vi "SBND_TST.vi"() -> ()   [LabVIEW 2014]
uses:
  D:/share/SBND/SBNE_SW/LBNE_DLL/LBNE_DLL/bin/Debug/LBNE_DLL.dll
  LBNE_DLL/LBNE_DLL/bin/Debug/LBNE_DLL.dll
  LBNE_Global .vi
  <vilib>/express/express analysis/Spectral/Block/exnSpectralBlock spectral measurements peak poly.vi
  <vilib>/express/express analysis/Spectral/Block/exnSpectralBlock spectral measurements peak WFM.vi
  <vilib>/express/express analysis/Spectral/XNode/ExpressSpectralMeasurementsBlockNode.xnode
  <vilib>/Analysis/NI_AAL_SigProc.lvlib
  <instrlib>/RIGOL DP1000 Series/RIGOL DP1000 Series.lvlib
panel:
  out "error out":errorcluster={"status"=TRUE, "code"=-1073807343, "source"="VISA Open in RIGOL DP1000 Series.lvlib:Initialize.vi->SBND_TST.vi"}
  out "VISA resource name out":refnum<visa-resource-name>
  out "ADC_hist":u32[][](array[numeric])
  out "FF_B_SHFT 2":u32 format="%x"
  out "TP_RES":u32=39382807
  out "FE RB":u32[](array[numeric])=[3368601800, 3368601800, 3368601800, 3368601800, 3368601800, 3368601800, 3368601800, 3368601800, 3355494400, 3368601800, 3368601800, 3368601800, 3368601800, 3368601800, 3368601800, 3368601800, 13107400, 3368602828, 3368602828, 3368602828, 3368602828, 3368602828, 3368602828, 3368602828, 3368602828, 3355495424, 3368602828, 3368602828, 3368602828, 3368602828, 3368602828, 3368602828, 3368602828, 13107404] format="%x"
  out "Array 2":u32[](array[numeric])=[3368601800, 3368601800, 3368601800, 3368601800, 3368601800, 3368601800, 3368601800, 3368601800, 3355494400, 3368601800, 3368601800, 3368601800, 3368601800, 3368601800, 3368601800, 3368601800, 13107400, 3368602828, 3368602828, 3368602828, 3368602828, 3368602828, 3368602828, 3368602828, 3368602828, 3355495424, 3368602828, 3368602828, 3368602828, 3368602828, 3368602828, 3368602828, 3368602828, 13107404] format="%x"
  out "ADC RB":u32[](array[numeric])=[202116108, 202116108, 202116108, 202116108, 202116620, 202116108, 202116108, 202116108, 422910261, 404232216, 404232216, 404232216, 404232216, 404232216, 404232216, 404232216, 1779984920, 808595506, 808464432, 808464432, 808464432, 808464432, 808464432, 808464432, 808464432, 1691641044, 1616928864, 1616928864, 1616928864, 1616928864, 1616928864, 1616928864, 1616928864, 2824906848, 589833] format="%x"
  out "Array":u32[](array[numeric])=[202116108, 202116108, 202116108, 202116108, 202116620, 202116108, 202116108, 202116108, 422910261, 404232216, 404232216, 404232216, 404232216, 404232216, 404232216, 404232216, 1779984920, 808595506, 808464432, 808464432, 808464432, 808464432, 808464432, 808464432, 808464432, 1691641044, 1616928864, 1616928864, 1616928864, 1616928864, 1616928864, 1616928864, 1616928864, 2824906848, 589833] format="%x"
  out "FF_B_SHFT":u32 format="%x"
  in  "stop":bool
  in  "Tab Control":T1(tab)=enum."UDP CONTROL"
  in  "RESET 6":bool
  in  "samples 3":i32
  in  "CHANNEL":u8(slide)=14
  in  "Tab Control 3":enum32{"CLOCK PHASE CONTROL", "DC CONTROL"}(tab)
  in  "DATA SHIFT":u8[](array[numeric])=[0, 0, 0, 0, 0, 0, 0, 0] format="%x"
  in  "ADC_TM EN":bool
  in  "TEST PAT":u32=273 format="%x"
  in  "TEST EN":u32 format="%x"
  out "result":u32=17891328
  in  "ADC  CLK \nPHASE":bool[](array[boolean])=[FALSE, TRUE, TRUE, TRUE, TRUE, TRUE, TRUE, TRUE]
  in  "ASIC/CHN READOUT":bool=TRUE
  in  "RESTART":bool
  in  "ENABLE/\n DISABLE":bool
  in  "Voltage Level":dbl=1.6160000000000012 caption="Voltage Level (0 V)" format="%.2f"
  in  "Enable Output":bool=TRUE caption="Enable Output (T: Enable)"
  in  "START VOLTAGE":dbl caption="Voltage Level (0 V)" format="%.2f"
  in  "STOP VOLTAGE":dbl=1.6 caption="Voltage Level (0 V)" format="%.2f"
  in  "STEPS":dbl=100.0 caption="Voltage Level (0 V)" format="%.2f"
  out "Elapsed Time (s)":dbl=4.0854082107543945
  in  "Time Target (s)":dbl=4.0
  in  "number_of_samples":u32=10000
  in  "FREQ":u16=600
  in  "DLY":u8=239
  in  "AMPL":u8=23 format="%x"
  in  "CHIP":u8(slide)=1 scale=0.0..7.0
  in  "STOP_DATA":bool
  in  "AUTO SCALE":bool
  in  "x":u32=100
  out "ADC_RMS":dbl=266.1273079482756
  out "ADC_MEAN":dbl=878.6148385161484
  out "ADC_CNT":u32=10001
  out "ADC_PEAK":u32=861
  out "Waveform Graph 4":u32[](graph)
  out "ADC HIST":u32[](graph)=[0, 0, 0, 0, 0, 0, 0, 0, 0, 0, 0, 0, 0, 0, 0, 0, 0, 0, 0, 0, 0, 0, 0, 0, 0, 0, 0, 0, 0, 0, 0, 0, 0, 0, 0, 0, 0, 0, 0, 0, 0, 0, 0, 0, 0, 0, 0, 0, 0, 0, 0, 0, 0, 0, 0, 0, 0, 0, 0, 0, 0, 0, 0, 0, 0, 0, 0, 0, 0, 0, 0, 0, 0, 0, 0, 0, 0, 0, 0, 0, 0, 0, 0, 0, 0, 0, 0, 0, 0, 0, 0, 3, 6, 14, 34, 77, 158, 218, 258, 291, 228, 164, 164, 168, 206, 287, 248, 250, 130, 89, 50, 19, 10, 1, 1, 1, 1, 0, 0, 0, 0, 0, 0, 0, 0, 0, 0, 1192, 0, 0, 0, 0, 13, 22, 54, 224, 504, 905, 1368, 2740, 1873, 2049, 2667, 2499, 2671, 2484, 1903, 2513, 2643, 2551, 4237, 7695, 9164, 11409, 12405, 9832, 11511, 10095, 5591, 4006, 2700, 1449, 1009, 1689, 2755, 2668, 2468, 1996, 1241, 770, 588, 245, 170, 240, 279, 310, 502, 281, 313, 266, 144, 101, 37, 16, 2, 1, 0, 0, 0, 0, 0, 1, 1, 2, 5, 22, 20, 108, 384, 374, 456, 2012, 1429, 1580, 2732, 1877, 2486, 1878, 1144, 1090, 1311, 994, 1135, 1240, 1593, 1908, 1396, 1330, 1168, 892, 905, 814, 483, 295, 160, 89, 33, 46, 24, 4, 2, 2, 0, 0, 0, 0, 0, 0, 0, 0, 0, 0, 0, 0, 0, 0, 0, 0, 0, 0, 0, 0, 0, 0, 0, 0, 0, 0, 0, 0, 0, 0, 0, 0, 0, 0, 0, 0, 0, 0, 0, 0, 0, 0, 0, 0, 0, 0, 0, 0, 0, 0, 0, 0, 0, 0, 0, 0, 0, 0, 0, 0, 0, 0, 0, 0, 0, 0, 0, 0, 0, 0, 0, 0, 0, 0, 0, 0, 0, 0, 0, 0, 0, 0, 0, 0, 0, 0, 0, 0, 0, 0, 0, 0, 0, 0, 0, 0, 0, 0, 0, 2, 0, 0, 0, 5, 5, 7, 13, 24, 53, 59, 57, 93, 90, 175, 151, 197, 231, 224, 185, 146, 154, 201, 194, 224, 298, 282, 356, 374, 409, 536, 727, 778, 721, 849, 740, 553, 700, 735, 1000, 603, 707, 1034, 1109, 821, 927, 785, 595, 567, 564, 330, 366, 679, 55, 1, 1, 1, 0, 0, 0, 0, 0, 0, 0, 0, 0, 0, 0, 0, 0, 0, 0, 0, 0, 0, 0, 0, 0, 0, 0, 0, 0, 0, 0, 0, 0, 0, 0, 0, 0, 0, 0, 0, 0, 0, 0, 0, 0, 0, 1, 0, 0, 0, 0, 0, 2, 2, 5, 4, 9, 7, 10, 26, 46, 40, 90, 1082, 322, 1088, 442, 836, 439, 891, 1626, 760, 547, 1757, 841, 554, 1030, 578, 730, 569, 318, 226, 242, 126, 107, 91, 115, 102, 124, 163, 170, 131, 182, 201, 203, 244, 369, 265, 317, 386, 487, 538, 624, 601, 665, 707, 820, 906, 953, 794, 673, 685, 469, 733, 626, 476, 385, 317, 328, 276, 263, 185, 130, 92, 60, 80, 64, 1093, 4, 168, 88, 166, 112, 193, 168, 236, 209, 214, 209, 218, 117, 119, 109, 117, 211, 200, 177, 224, 226, 217, 201, 197, 187, 254, 261, 262, 331, 401, 412, 458, 653, 682, 552, 817, 940, 903, 979, 991, 965, 1040, 1249, 1244, 1239, 1034, 1100, 711, 784, 894, 1195, 523, 649, 797, 987, 475, 685, 512, 204, 300, 331, 151, 221, 328, 637, 204, 39, 56, 84, 56, 40, 26, 19, 22, 22, 14, 13, 18, 7, 21, 8, 5, 6, 2, 2, 2, 2, 6, 7, 4, 7, 2, 9, 7, 2, 7, 13, 8, 9, 3, 8, 2, 3, 5, 3, 0, 3, 6, 1, 6, 0, 1, 1, 0, 0, 0, 3, 1, 0, 2, 0, 2, 2, 5, 7, 16, 25, 301, 112, 514, 193, 396, 270, 283, 249, 516, 499, 378, 223, 424, 114, 78, 143, 127, 98, 69, 87, 65, 52, 26, 12, 7, 4, 6, 2, 1, 0, 0, 0, 0, 0, 0, 1, 0, 0, 0, 1, 1, 2, 1, 2, 0, 6, 7, 14, 15, 17, 31, 43, 30, 73, 136, 223, 146, 325, 332, 217, 337, 577, 273, 709, 6565, 1020, 4028, 3190, 2670, 1367, 6064, 12963, 9682, 7447, 16075, 35640, 37568, 39568, 49342, 52439, 69153, 132918, 141159, 153723, 209388, 258329, 308095, 353864, 329546, 357993, 372338, 444794, 403668, 387789, 442035, 387599, 373766, 462530, 389136, 302585, 345607, 255765, 200030, 226602, 175065, 138775, 108854, 98961, 97466, 86035, 74698, 54581, 80731, 88694, 89089, 83800, 71862, 89184, 108548, 56989, 62075, 90008, 45061, 61853, 81792, 60331, 54353, 81241, 387831, 75572, 285158, 53776, 81654, 51495, 48849, 31904, 48817, 41495, 26095, 8387, 15990, 2815, 1498, 2528, 1399, 770, 476, 633, 523, 440, 398, 545, 737, 610, 628, 705, 501, 707, 954, 756, 687, 892, 578, 366, 779, 785, 594, 493, 404, 314, 394, 323, 222, 148, 104, 78, 32, 53, 38, 43, 18, 19, 26, 40, 74, 91, 86, 157, 201, 267, 148, 370, 3626, 628, 4250, 1896, 5374, 3547, 6713, 22196, 17972, 7155, 67075, 46912, 30392, 109706, 81820, 183064, 239866, 194477, 203621, 382631, 283708, 321162, 314384, 400619, 514366, 420790, 401774, 447681, 293012, 410139, 518465, 380312, 343262, 406642, 246054, 155890, 298769, 294920, 178359, 144732, 107398, 76592, 77281, 62194, 38478, 24710, 14754, 13399, 4397, 5646, 3688, 4994, 1182, 1748, 1773, 1489, 533, 710, 378, 154, 142, 250, 39, 119, 127, 0, 5, 2, 3, 0, 1, 1, 0, 0, 0, 0, 0, 0, 0, 0, 0, 0, 0, 0, 0, 0, 0, 0, 1, 0, 1, 2, 3, 1, 3, 7, 6, 24, 18, 20, 45, 83, 82, 108, 169, 158, 247, 377, 420, 467, 449, 601, 297, 575, 492, 1091, 351, 673, 974, 1000, 586, 969, 753, 351, 480, 821, 277, 691, 1794, 308, 823, 168, 281, 172, 140, 129, 176, 156, 74, 36, 78, 6, 7, 9, 5, 1, 0, 0, 0, 0, 1, 0, 1, 0, 0, 0, 0, 0, 0, 0, 0, 0, 0, 0, 0, 0, 0, 0, 0, 0, 0, 0, 0, 0, 0, 0, 0, 0, 0, 0, 0, 0, 0, 0, 0, 0, 0, 0, 0, 0, 0, 0, 0, 0, 0, 0, 0, 0, 0, 0, 0, 0, 0, 0, 0, 0, 0, 0, 0, 0, 0, 0, 0, 0, 0, 0, 0, 0, 0, 0, 0, 0, 0, 0, 0, 0, 0, 0, 0, 0, 0, 0, 0, 0, 0, 0, 0, 0, 0, 0, 0, 0, 0, 0, 0, 0, 0, 0, 0, 0, 0, 0, 0, 0, 1, 0, 0, 0, 4, 4, 5, 2, 11, 35, 22, 11, 96, 68, 49, 216, 167, 360, 420, 360, 363, 704, 566, 620, 575, 803, 1006, 863, 755, 814, 508, 817, 1036, 744, 619, 708, 410, 471, 513, 640, 272, 424, 253, 270, 202, 169, 281, 131, 115, 145, 23, 54, 37, 14, 15, 13, 5, 2, 1, 0, 0, 0, 0, 0, 0, 0, 0, 246, 0, 0, 0, 0, 0, 0, 0, 0, 0, 0, 0, 0, 0, 0, 2, 1, 2, 2, 2, 2, 4, 5, 10, 13, 13, 32, 39, 33, 100, 107, 123, 199, 247, 104, 202, 500, 531, 442, 602, 482, 531, 910, 885, 879, 695, 717, 824, 233, 845, 682, 592, 350, 602, 716, 348, 386, 444, 165, 113, 228, 76, 97, 257, 13, 87, 31, 102, 74, 83, 116, 249, 260, 175, 99, 458, 136, 101, 225, 148, 70, 38, 30, 22, 12, 4, 2, 2, 0, 1, 0, 0, 0, 0, 0, 0, 0, 0, 0, 0, 0, 0, 0, 0, 0, 0, 1, 0, 0, 0, 1, 0, 1, 2, 0, 1, 2, 2, 7, 4, 6, 3, 9, 12, 12, 16, 18, 746, 35, 1, 1, 0, 0, 2, 12, 22, 34, 80, 39, 36, 62, 54, 31, 22, 17, 16, 20, 7, 6, 6, 3, 2, 2, 1, 0, 0, 1, 1, 1, 8, 5, 10, 28, 28, 17, 10, 14, 13, 12, 7, 6, 6, 7, 8, 14, 19, 32, 38, 68, 83, 121, 141, 123, 159, 234, 100, 171, 193, 121, 142, 77, 160, 33, 0, 0, 0, 2, 0, 0, 0, 0, 0, 0, 0, 0, 0, 0, 0, 0, 0, 0, 0, 0, 0, 0, 0, 1, 0, 0, 1, 0, 0, 2, 4, 4, 9, 2, 3, 9, 16, 2, 21, 9, 5, 18, 23, 29, 44, 43, 50, 39, 63, 78, 44, 56, 114, 42, 97, 115, 139, 217, 156, 181, 203, 199, 6573, 195, 474, 303, 528, 388, 594, 913, 708, 452, 1655, 1032, 861, 2033, 1520, 2054, 2506, 1797, 2083, 1860, 1482, 1666, 1297, 1236, 1046, 827, 506, 401, 328, 258, 210, 80, 68, 82, 45, 21, 33, 65, 64, 68, 60, 73, 100, 65, 108, 115, 87, 134, 47, 115, 97, 81, 32, 39, 40, 47, 21, 19, 19, 1, 1, 5, 0, 0, 438, 0, 0, 0, 0, 1, 0, 0, 1, 1, 0, 0, 0, 0, 0, 0, 0, 0, 0, 0, 0, 0, 3, 3, 1, 11, 28, 30, 16, 23, 52, 20, 13, 8, 7, 8, 4, 6, 2, 1, 1, 0, 0, 0, 0, 0, 0, 0, 0, 0, 0, 0, 0, 0, 0, 0, 0, 0, 0, 0, 0, 0, 0, 0, 0, 0, 0, 0, 0, 0, 0, 0, 0, 0, 0, 0, 0, 0, 0, 0, 0, 0, 0, 0, 0, 0, 0, 0, 0, 0, 0, 0, 0, 0, 0, 0, 0, 0, 0, 0, 0, 0, 0, 0, 0, 0, 0, 0, 0, 0, 0, 0, 0, 0, 0, 0, 0, 0, 0, 0, 0, 0, 0, 0, 0, 0, 0, 0, 0, 0, 0, 0, 0, 0, 0, 0, 0, 0, 0, 0, 0, 0, 0, 0, 0, 0, 0, 0, 0, 0, 0, 0, 0, 0, 0, 0, 0, 0, 0, 0, 0, 0, 0, 0, 0, 0, 0, 0, 0, 0, 0, 0, 0, 0, 0, 0, 0, 0, 0, 1, 3, 3, 2, 10, 18, 17, 36, 108, 93, 76, 123, 184, 1105, 44, 250, 103, 200, 80, 74, 38, 45, 19, 14, 4, 4, 0, 0, 0, 1, 0, 0, 0, 0, 0, 0, 0, 0, 0, 0, 0, 0, 0, 0, 0, 0, 0, 0, 0, 0, 0, 0, 0, 0, 0, 0, 0, 0, 0, 0, 0, 0, 0, 0, 0, 0, 0, 0, 0, 0, 0, 0, 0, 0, 0, 0, 0, 0, 0, 0, 0, 0, 0, 0, 0, 0, 0, 0, 0, 0, 0, 0, 0, 0, 0, 0, 0, 0, 0, 0, 0, 0, 0, 0, 0, 0, 0, 0, 0, 0, 0, 0, 0, 0, 0, 0, 0, 0, 0, 0, 0, 0, 0, 0, 0, 0, 0, 0, 0, 0, 0, 0, 0, 0, 0, 0, 0, 0, 0, 0, 0, 0, 0, 0, 0, 0, 0, 0, 0, 0, 0, 0, 0, 0, 0, 0, 0, 0, 0, 0, 0, 0, 0, 0, 0, 0, 0, 0, 0, 0, 0, 0, 0, 0, 0, 0, 0, 0, 0, 0, 0, 0, 0, 0, 0, 0, 0, 0, 0, 0, 0, 0, 0, 0, 0, 0, 0, 0, 0, 0, 0, 0, 0, 0, 0, 0, 0, 0, 0, 0, 0, 0, 0, 0, 0, 0, 0, 0, 0, 0, 0, 0, 0, 0, 0, 0, 0, 0, 0, 0, 0, 0, 0, 0, 0, 0, 2, 0, 3, 1, 2, 1, 6, 6, 10, 17, 16, 24, 43, 70, 81, 111, 129, 99, 183, 228, 308, 225, 340, 615, 420, 565, 770, 492, 411, 825, 587, 642, 768, 1922, 498, 1701, 459, 688, 331, 449, 425, 210, 81, 282, 80, 35, 115, 29, 27, 15, 10, 5, 10, 3, 2, 3, 0, 1, 0, 0, 2, 0, 0, 0, 0, 0, 0, 0, 0, 0, 0, 0, 0, 0, 0, 0, 0, 0, 0, 0, 0, 0, 0, 0, 0, 0, 0, 0, 0, 0, 0, 0, 0, 0, 0, 0, 0, 0, 0, 0, 0, 0, 0, 0, 0, 0, 0, 0, 0, 0, 0, 0, 0, 0, 0, 0, 0, 0, 0, 0, 0, 0, 0, 0, 0, 0, 0, 0, 0, 0, 0, 0, 0, 0, 0, 0, 0, 0, 0, 0, 0, 0, 0, 0, 0, 0, 0, 0, 0, 0, 0, 0, 0, 0, 0, 0, 0, 0, 0, 0, 0, 0, 0, 0, 0, 0, 0, 0, 0, 0, 0, 0, 0, 0, 0, 0, 0, 0, 0, 0, 0, 0, 0, 0, 0, 0, 0, 0, 0, 0, 0, 0, 0, 0, 0, 0, 0, 0, 0, 0, 0, 0, 0, 0, 0, 0, 0, 0, 0, 0, 0, 0, 0, 0, 0, 0, 0, 0, 0, 0, 0, 0, 0, 0, 0, 0, 0, 0, 0, 0, 0, 0, 0, 0, 1, 0, 1, 0, 0, 1, 2, 14, 21, 19, 28, 52, 27, 97, 51, 62, 48, 83, 280, 155, 116, 308, 154, 96, 152, 63, 249, 131, 189, 21, 91, 30, 59, 16, 8, 17, 9, 3, 2, 3, 0, 1, 2, 7, 1, 7, 27, 22, 24, 60, 43, 33, 110, 112, 103, 3825, 0, 3, 12, 148, 194, 204, 1207, 883, 225, 887, 902, 399, 918, 329, 362, 991, 949, 364, 541, 316, 228, 206, 176, 210, 107, 85, 51, 49, 12, 16, 13, 5, 4, 4, 1, 0, 0, 0, 0, 0, 1, 0, 0, 0, 0, 0, 0, 0, 0, 0, 0, 0, 0, 0, 0, 0, 0, 0, 0, 0, 0, 0, 0, 0, 0, 0, 0, 0, 0, 0, 0, 0, 0, 0, 0, 0, 0, 0, 0, 0, 0, 0, 0, 0, 0, 0, 0, 0, 0, 0, 0, 0, 0, 0, 0, 0, 0, 0, 0, 0, 0, 0, 0, 1, 0, 1, 3, 4, 5, 11, 11, 15, 33, 45, 40, 97, 100, 103, 140, 244, 227, 223, 365, 242, 156, 125, 127, 256, 21, 49, 7, 2, 1, 0, 0, 1, 0, 0, 0, 0, 0, 0, 0, 0, 0, 0, 0, 0, 0, 0, 0, 0, 0, 0, 0, 0, 0, 0, 0, 0, 0, 0, 0, 0, 0, 0, 0, 0, 0, 0, 0, 0, 0, 0, 0, 0, 0, 0, 0, 0, 0, 0, 0, 0, 0, 0, 0, 0, 0, 0, 0, 0, 0, 0, 0, 0, 0, 0, 0, 0, 0, 0, 0, 0, 0, 0, 0, 0, 0, 0, 0, 0, 0, 0, 0, 0, 0, 0, 0, 0, 0, 0, 0, 0, 0, 0, 0, 0, 0, 0, 0, 0, 0, 0, 0, 0, 0, 0, 0, 0, 0, 0, 0, 0, 0, 0, 0, 0, 0, 0, 0, 0, 0, 0, 0, 0, 0, 0, 0, 0, 0, 0, 0, 0, 0, 0, 0, 0, 0, 0, 0, 0, 0, 0, 0, 0, 0, 0, 0, 0, 0, 0, 0, 0, 0, 0, 0, 0, 0, 0, 0, 0, 0, 0, 0, 0, 0, 0, 0, 0, 0, 0, 0, 0, 0, 0, 0, 0, 0, 0, 0, 0, 0, 0, 0, 0, 0, 0, 0, 0, 0, 0, 0, 0, 0, 0, 0, 0, 0, 0, 0, 0, 0, 0, 0, 0, 0, 0, 0, 0, 0, 0, 0, 0, 0, 0, 0, 0, 0, 0, 0, 0, 0, 0, 0, 0, 0, 0, 0, 0, 0, 0, 0, 0, 0, 0, 0, 0, 0, 0, 0, 0, 0, 0, 0, 0, 0, 0, 0, 0, 0, 0, 0, 0, 0, 0, 0, 2, 0, 1, 1, 4, 4, 18, 10, 23, 52, 54, 87, 124, 139, 164, 334, 266, 411, 354, 452, 682, 602, 649, 783, 633, 852, 980, 728, 603, 1049, 726, 563, 791, 782, 491, 475, 324, 240, 236, 186, 131, 116, 80, 37, 23, 36, 38, 16, 8, 8, 8, 1, 3, 0, 0, 0, 2, 1, 0, 1, 0, 0, 0, 0, 0, 0, 0, 0, 0, 0, 0, 0, 0, 0, 0, 0, 0, 0, 0, 0, 0, 0, 0, 0, 0, 0, 0, 0, 0, 0, 0, 0, 0, 0, 0, 0, 0, 0, 0, 0, 0, 0, 0, 0, 0, 0, 0, 0, 0, 0, 0, 0, 0, 0, 0, 0, 0, 0, 0, 0, 0, 0, 0, 0, 0, 0, 0, 0, 0, 0, 0, 0, 0, 0, 0, 0, 0, 0, 0, 0, 0, 0, 0, 0, 0, 0, 0, 0, 0, 0, 0, 0, 0, 0, 0, 0, 0, 0, 0, 0, 0, 0, 0, 0, 0, 0, 0, 0, 0, 0, 0, 0, 0, 0, 0, 0, 0, 0, 0, 0, 0, 0, 0, 0, 0, 0, 0, 0, 0, 0, 0, 0, 0, 0, 0, 0, 0, 0, 0, 0, 0, 0, 0, 0, 0, 0, 0, 0, 0, 0, 0, 0, 0, 0, 0, 0, 0, 0, 0, 0, 0, 0, 0, 0, 0, 0, 0, 0, 0, 0, 0, 0, 0, 0, 0, 0, 0, 0, 0, 0, 0, 0, 0, 0, 0, 0, 0, 0, 0, 0, 0, 0, 0, 0, 0, 0, 0, 0, 0, 0, 0, 0, 0, 0, 0, 0, 0, 0, 0, 0, 0, 0, 0, 0, 0, 0, 0, 0, 0, 0, 0, 0, 0, 0, 0, 0, 0, 0, 0, 0, 0, 0, 0, 0, 0, 0, 0, 0, 0, 0, 0, 0, 0, 0, 0, 0, 0, 0, 0, 0, 0, 0, 0, 0, 0, 0, 0, 0, 0, 0, 0, 0, 0, 0, 0, 0, 0, 0, 0, 0, 0, 0, 0, 0, 0, 0, 0, 0, 0, 0, 0, 0, 0, 0, 0, 0, 0, 0, 0, 0, 0, 0, 0, 0, 0, 0, 0, 0, 0, 0, 0, 0, 0, 0, 0, 0, 0, 0, 0, 0, 0, 0, 0, 0, 0, 0, 0, 0, 0, 0, 0, 0, 0, 0, 0, 0, 0, 0, 0, 0, 0, 0, 0, 0, 0, 0, 0, 0, 0, 0, 0, 0, 0, 0, 0, 0, 0, 0, 0, 0, 0, 0, 0, 0, 0, 0, 0, 0, 0, 0, 0, 0, 0, 0, 0, 0, 0, 0, 0, 0, 0, 0, 0, 0, 0, 0, 0, 0, 0, 0, 0, 0, 0, 0, 0, 0, 0, 0, 0, 0, 0, 0, 0, 0, 0, 0, 0, 0, 0, 0, 1, 0, 0, 0, 2, 6, 8, 6, 8, 18, 32, 39, 55, 124, 123, 166, 182, 171, 328, 273, 185, 182, 190, 181, 158, 87, 55, 16, 35, 7, 5, 7, 2, 1, 1, 0, 0, 0, 0, 1, 0, 0, 0, 0, 0, 0, 0, 0, 0, 0, 0, 0, 0, 0, 0, 0, 0, 0, 0, 0, 0, 0, 0, 0, 0, 0, 0, 0, 0, 0, 0, 0, 0, 0, 0, 0, 0, 0, 0, 0, 0, 0, 0, 0, 0, 0, 0, 0, 0, 0, 0, 0, 0, 0, 0, 0, 0, 0, 0, 0, 0, 0, 0, 0, 0, 0, 0, 0, 0, 0, 0, 0, 0, 0, 0, 0, 0, 0, 0, 0, 0, 0, 0, 0, 0, 0, 0, 0, 0, 0, 0, 0, 0, 0, 0, 0, 0, 0, 0, 0, 0, 0, 0, 0, 0, 0, 0, 0, 0, 0, 0, 0, 0, 0, 0, 0, 0, 0, 0, 0, 0, 0, 0, 0, 0, 0, 0, 0, 0, 0, 0, 0, 0, 0, 0, 0, 0, 0, 0, 0, 0, 0, 0, 0, 0, 0, 0, 0, 0, 0, 0, 0, 0, 0, 0, 0, 0, 0, 0, 0, 0, 1, 1, 0, 2, 1, 2, 11, 6, 16, 23, 81, 60, 89, 35, 105, 88, 176, 155, 118, 73, 40, 21, 25, 19, 14, 23, 13, 17, 26, 16, 12, 22, 12, 10, 3, 3, 0, 0, 1, 1, 1334, 0, 0, 0, 0, 0, 0, 0, 0, 0, 0, 0, 0, 0, 1, 1, 0, 0, 0, 0, 3, 0, 3, 4, 5, 8, 7, 14, 19, 38, 61, 56, 121, 142, 100, 173, 400, 369, 439, 502, 469, 510, 711, 666, 742, 727, 657, 732, 528, 689, 931, 474, 523, 813, 758, 410, 541, 490, 242, 235, 377, 136, 223, 732, 6, 417, 182, 734, 363, 366, 1072, 708, 292, 1128, 642, 507, 914, 663, 730, 1017, 636, 477, 925, 662, 530, 402, 375, 398, 255, 168, 158, 85, 61, 46, 32, 6, 11, 7, 3, 4, 3, 0, 0, 1, 0, 0, 0, 0, 0, 0, 0, 0, 0, 0, 0, 0, 0, 0, 0, 0, 0, 0, 0, 0, 0, 0, 0, 0, 0, 0, 0, 0, 0, 0, 0, 0, 0, 0, 0, 0, 0, 0, 0, 0, 0, 0, 0, 0, 0, 0, 0, 0, 0, 0, 0, 0, 0, 0, 0, 0, 0, 0, 0, 0, 0, 0, 0, 0, 0, 0, 0, 0, 0, 0, 0, 0, 0, 0, 0, 0, 0, 0, 0, 0, 0, 0, 0, 0, 0, 0, 0, 0, 0, 0, 0, 0, 0, 0, 0, 0, 0, 0, 0, 0, 0, 0, 0, 0, 0, 0, 0, 0, 0, 0, 0, 0, 0, 0, 0, 0, 1, 1, 1, 1, 5, 6, 5, 8, 16, 14, 22, 25, 38, 32, 40, 66, 77, 102, 103, 139, 184, 208, 262, 325, 297, 416, 420, 508, 481, 490, 370, 327, 238, 170, 165, 408, 867, 1745, 773, 605, 219, 189, 508, 231, 96, 57, 80, 63, 35, 17, 21, 7, 11, 5, 0, 1, 1, 1, 0, 0, 0, 0, 0, 0, 0, 0, 1, 0, 1, 0, 0, 0, 2, 2, 6, 2, 6, 16, 15, 15, 25, 33, 42, 45, 62, 56, 57, 43, 114, 109, 121, 180, 151, 148, 163, 113, 70, 36, 23, 60, 106, 441, 119, 48, 39, 42, 19, 17, 15, 16, 17, 7, 26, 20, 32, 117, 80, 126, 181, 151, 137, 140, 91, 203, 111, 45, 21, 18, 13, 3, 3, 1, 0, 0, 0, 1, 0, 0, 0, 0, 0, 0, 0, 0, 0, 0, 0, 0, 0, 0, 0, 0, 0, 0, 2, 1, 4, 9, 7, 19, 22, 30, 36, 191, 8, 249, 245, 354, 223, 260, 131, 211, 176, 129, 83, 122, 50, 23, 33, 23, 9, 2, 2, 0, 1, 0, 0, 0, 0, 0, 0, 0, 0, 0, 0, 0, 0, 0, 0, 0, 0, 0, 0, 0, 0, 0, 0, 0, 0, 0, 0, 0, 0, 0, 0, 0, 0, 0, 0, 0, 0, 0, 0, 0, 0, 0, 0, 0, 0, 0, 0, 0, 0, 0, 0, 0, 0, 0, 0, 0, 0, 0, 0, 0, 0, 0, 0, 0, 0, 0, 0, 0, 0, 0, 0, 0, 0, 0, 0, 0, 0, 0, 0, 0, 0, 0, 0, 0, 0, 0, 0, 0, 0, 0, 0, 0, 0, 0, 0, 0, 0, 0, 0, 0, 0, 0, 0, 0, 0, 0, 0, 0, 0, 0, 0, 0, 0, 1, 0, 4, 7, 18, 11, 51, 44, 55, 108, 152, 195, 154, 271, 267, 214, 259, 158, 179, 110, 143, 97, 33, 42, 39, 24, 10, 4, 2, 3, 0, 0, 0, 0, 0, 0, 0, 0, 0, 0, 0, 0, 0, 0, 0, 0, 0, 0, 0, 0, 0, 0, 0, 0, 0, 0, 0, 0, 1602, 0, 0, 0, 0, 0, 0, 0, 0, 0, 0, 0, 0, 0, 0, 0, 0, 0, 0, 0, 0, 0, 0, 0, 0, 0, 0, 1, 1, 3, 5, 1, 5, 12, 14, 5, 24, 42, 57, 57, 63, 78, 77, 100, 134, 195, 211, 170, 257, 278, 435, 412, 391, 475, 570, 447, 610, 593, 420, 373, 807, 443, 533, 508, 1825, 1306, 158, 165, 384, 133, 112, 202, 66, 13, 52, 16, 7, 6, 1, 0, 0, 0, 1, 0, 0, 0, 1, 1, 8, 11, 19, 38, 27, 45, 70, 95, 93, 247, 326, 307, 537, 854, 728, 587, 381, 262, 129, 74, 41, 55, 73, 71, 87, 79, 135, 108, 98, 104, 119, 82, 141, 140, 84, 51, 95, 46, 28, 22, 46, 9358, 1, 4, 1, 1, 2, 0, 0, 0, 0, 0, 0, 0, 0, 0, 0, 0, 0, 0, 0, 0, 0, 0, 0, 0, 0, 0, 0, 0, 0, 0, 0, 0, 0, 0, 0, 0, 0, 0, 0, 0, 0, 0, 0, 0, 0, 0, 0, 0, 0, 0, 0, 0, 0, 0, 0, 0, 0, 0, 0, 0, 0, 0, 0, 0, 0, 0, 0, 0, 0, 0, 0, 0, 0, 0, 0, 0, 0, 0, 0, 0, 0, 0, 0, 0, 0, 0, 0, 0, 0, 0, 0, 0, 0, 0, 0, 0, 0, 0, 0, 0, 0, 0, 0, 0, 0, 0, 0, 0, 0, 0, 0, 0, 0, 0, 0, 0, 0, 0, 0, 0, 0, 0, 0, 0, 0, 0, 0]
  out "samples 4":u32=20161263
  out "Waveform Graph 5":u32[](graph)=[871, 868, 866, 864, 864, 860, 861, 859, 860, 859, 858, 856, 857, 861, 864, 880, 1206, 2194, 3322, 3968, 3903, 3346, 2593, 1918, 1420, 1112, 951, 885, 863, 862, 861, 859, 855, 853, 852, 855, 856, 860, 861]
  in  "length":i32=39 min=10 max=65 step=1
  in  "SYNC":bool=TRUE
  in  "FILE PATH":path=path "C:/Users/jfried/Desktop/New folder (11)"
  in  "FILE NAME 2":string="1459002fff"
  in  "SAVE TO \nFILE":bool
  out "Store_Data":bool
  in  "SYNC 3":bool=TRUE
  out "Waveform Graph":cluster{"f0":dbl, "df":dbl, "magnitude":dbl[]}(graph)={"f0"=0.0, "df"=199.98000199980004, "magnitude"=array[5001 elements]}
  in  "Boolean":bool
  in  "EN peak":bool
  in  "peak upper limit":dbl=800.0
  in  "peak lower limit":dbl=700.0
  in  "EN mean":bool=TRUE
  in  "Start channel":u8
  in  "Start chip":u8
  out "CUR_CHP":u8=5 caption="CHIP"
  out "CUR_CHN":u8=7 caption="CHANNEL"
  in  "Tab Control 2":enum32{"Page 1", "Page 2"}(tab)=enum."Page 2"
  in  "length 2":i32=40 min=10 max=65 step=1
  out "Waveform Graph 6":u32[](graph)=[1526, 1518, 1514, 1520, 1526, 1528, 1520, 1518, 1524, 1526, 1522, 1516, 1516, 1516, 1514, 1512, 1790, 3620, 2450, 4094, 4094, 3966, 2180, 354, 3082, 2248, 1812, 1624, 1568, 1546, 1540, 1534, 1538, 1534, 1520, 1510, 1512, 1514, 1516, 1516]
  in  "AUTO SCALE 2":bool
  in  "x 2":u32=100
  out "ADC_RMS 2":dbl
  out "ADC_MEAN 2":dbl
  out "ADC_CNT 2":u32=6001
  out "ADC_PEAK 2":u32
  out "Waveform Graph 7":u32[](graph)
  out "ADC HIST  2":u32[](graph)=[877735, 0, 0, 0, 0, 0, 0, 0, 0, 0, 0, 0, 0, 0, 0, 0, 0, 0, 0, 0, 0, 0, 0, 0, 0, 0, 0, 0, 0, 0, 0, 0, 0, 0, 0, 0, 0, 0, 0, 0, 0, 0, 0, 0, 0, 0, 0, 0, 0, 0, 0, 0, 0, 0, 0, 0, 0, 0, 0, 0, 0, 0, 0, 0, 0, 0, 0, 0, 0, 0, 0, 0, 0, 0, 0, 0, 0, 0, 0, 0, 0, 0, 0, 0, 0, 0, 0, 0, 0, 0, 0, 0, 0, 0, 0, 0, 0, 0, 0, 0, 0, 0, 0, 0, 0, 0, 0, 0, 0, 0, 0, 0, 0, 0, 0, 0, 0, 0, 0, 0, 0, 0, 0, 0, 0, 0, 0, 0, 0, 0, 0, 0, 0, 0, 0, 0, 0, 0, 0, 0, 0, 0, 0, 0, 0, 0, 0, 0, 0, 0, 0, 0, 0, 0, 0, 0, 0, 0, 0, 0, 0, 0, 0, 0, 0, 0, 0, 0, 0, 0, 0, 0, 0, 0, 0, 0, 0, 0, 0, 0, 0, 0, 0, 0, 0, 0, 0, 0, 0, 0, 0, 0, 0, 0, 0, 0, 0, 0, 0, 0, 0, 0, 0, 0, 0, 0, 0, 0, 0, 0, 0, 0, 0, 0, 0, 0, 0, 0, 0, 0, 0, 0, 0, 0, 0, 0, 0, 0, 0, 0, 0, 0, 0, 0, 0, 0, 0, 0, 0, 0, 0, 0, 0, 0, 0, 0, 0, 0, 0, 0, 0, 0, 0, 0, 0, 0, 0, 0, 0, 0, 0, 0, 0, 0, 0, 0, 0, 0, 0, 0, 0, 0, 0, 0, 0, 0, 0, 0, 0, 0, 0, 0, 0, 0, 0, 0, 0, 0, 0, 0, 0, 0, 0, 0, 0, 0, 0, 0, 0, 0, 0, 0, 0, 0, 0, 0, 0, 0, 0, 0, 0, 0, 0, 0, 0, 0, 0, 0, 0, 0, 0, 0, 0, 0, 0, 0, 0, 0, 0, 0, 0, 0, 0, 0, 0, 0, 0, 0, 0, 0, 0, 0, 0, 0, 0, 0, 0, 0, 0, 0, 0, 0, 0, 0, 0, 0, 0, 0, 0, 0, 0, 0, 0, 0, 0, 0, 0, 0, 0, 0, 0, 0, 0, 0, 0, 0, 0, 0, 0, 0, 0, 0, 0, 0, 0, 0, 0, 0, 0, 0, 0, 0, 0, 0, 0, 0, 0, 0, 0, 0, 0, 0, 0, 0, 0, 0, 0, 0, 0, 0, 0, 0, 0, 0, 0, 0, 0, 0, 0, 0, 0, 0, 0, 0, 0, 0, 0, 0, 0, 0, 0, 0, 0, 0, 0, 0, 0, 0, 0, 0, 0, 0, 0, 0, 0, 0, 0, 0, 0, 0, 0, 0, 0, 0, 0, 0, 0, 0, 0, 0, 0, 0, 0, 0, 0, 0, 0, 0, 0, 0, 0, 0, 0, 0, 0, 0, 0, 0, 0, 0, 0, 0, 0, 0, 0, 0, 0, 0, 0, 0, 0, 0, 0, 0, 0, 0, 0, 0, 0, 0, 0, 0, 0, 0, 0, 0, 0, 0, 0, 0, 0, 0, 0, 0, 0, 0, 0, 0, 0, 0, 0, 0, 0, 0, 0, 0, 0, 0, 0, 0, 0, 0, 0, 0, 0, 0, 0, 0, 0, 0, 0, 0, 0, 0, 0, 0, 0, 0, 0, 0, 0, 0, 0, 0, 0, 0, 0, 0, 0, 0, 0, 0, 0, 0, 0, 0, 0, 0, 0, 0, 0, 0, 0, 0, 0, 0, 0, 0, 0, 0, 0, 0, 0, 0, 0, 0, 0, 0, 0, 0, 0, 0, 0, 0, 0, 0, 0, 0, 0, 0, 0, 0, 0, 0, 0, 0, 0, 0, 0, 0, 0, 0, 0, 0, 0, 0, 0, 0, 0, 0, 0, 0, 0, 0, 0, 0, 0, 0, 0, 0, 0, 0, 0, 0, 0, 0, 0, 0, 0, 0, 0, 0, 0, 0, 0, 0, 0, 0, 0, 0, 0, 0, 0, 0, 0, 0, 0, 0, 0, 0, 0, 0, 0, 0, 0, 0, 0, 0, 0, 0, 0, 0, 0, 0, 0, 0, 0, 0, 0, 0, 0, 0, 0, 0, 0, 0, 0, 0, 0, 0, 0, 0, 0, 0, 0, 0, 0, 0, 0, 0, 0, 0, 0, 0, 0, 0, 0, 0, 0, 0, 0, 0, 0, 0, 0, 0, 0, 0, 0, 0, 0, 0, 0, 0, 0, 0, 0, 0, 0, 0, 0, 0, 0, 0, 0, 0, 0, 0, 0, 0, 0, 0, 0, 0, 0, 0, 0, 0, 0, 0, 0, 0, 0, 0, 0, 0, 0, 0, 0, 0, 0, 0, 0, 0, 0, 0, 0, 0, 0, 0, 0, 0, 0, 0, 0, 0, 0, 0, 0, 0, 0, 0, 0, 0, 0, 0, 0, 0, 0, 0, 0, 0, 0, 0, 0, 0, 0, 0, 0, 0, 0, 0, 0, 0, 0, 0, 0, 0, 0, 0, 0, 0, 0, 0, 0, 0, 0, 0, 0, 0, 0, 0, 0, 0, 0, 0, 0, 0, 0, 0, 0, 0, 0, 0, 0, 0, 0, 0, 0, 0, 0, 0, 0, 0, 0, 0, 0, 0, 0, 0, 0, 0, 0, 0, 0, 0, 0, 0, 0, 0, 0, 0, 0, 0, 0, 0, 0, 0, 0, 0, 0, 0, 0, 0, 0, 0, 0, 0, 0, 0, 0, 0, 0, 0, 0, 0, 0, 0, 0, 0, 0, 0, 0, 0, 0, 0, 0, 0, 0, 0, 0, 0, 0, 0, 0, 0, 0, 0, 0, 0, 0, 0, 0, 0, 0, 0, 0, 0, 0, 0, 0, 0, 0, 0, 0, 0, 0, 0, 0, 0, 0, 0, 0, 0, 0, 0, 0, 0, 0, 0, 0, 0, 0, 0, 0, 0, 0, 0, 0, 0, 0, 0, 0, 0, 0, 0, 0, 0, 0, 0, 0, 0, 0, 0, 0, 0, 0, 0, 0, 0, 0, 0, 0, 0, 0, 0, 0, 0, 0, 0, 0, 0, 0, 0, 0, 0, 0, 0, 0, 0, 0, 0, 0, 0, 0, 0, 0, 0, 0, 0, 0, 0, 0, 0, 0, 0, 0, 0, 0, 0, 0, 0, 0, 0, 0, 0, 0, 0, 0, 0, 0, 0, 0, 0, 0, 0, 0, 0, 0, 0, 0, 0, 0, 0, 0, 0, 0, 0, 0, 0, 0, 0, 0, 0, 0, 0, 0, 0, 0, 0, 0, 0, 0, 0, 0, 0, 0, 0, 0, 0, 0, 0, 0, 0, 0, 0, 0, 0, 0, 0, 0, 0, 0, 0, 0, 0, 0, 0, 0, 0, 0, 0, 0, 0, 0, 0, 0, 0, 0, 0, 0, 0, 0, 0, 0, 0, 0, 0, 0, 0, 0, 0, 0, 0, 0, 0, 0, 0, 0, 0, 0, 0, 0, 0, 0, 0, 0, 0, 0, 0, 0, 0, 0, 0, 0, 0, 0, 0, 0, 0, 0, 0, 0, 0, 0, 0, 0, 0, 0, 0, 0, 0, 0, 0, 0, 0, 0, 0, 0, 0, 0, 0, 0, 0, 0, 0, 0, 0, 0, 0, 0, 0, 0, 0, 0, 0, 0, 0, 0, 0, 0, 0, 0, 0, 0, 0, 0, 0, 0, 0, 0, 0, 0, 0, 0, 0, 0, 0, 0, 0, 0, 0, 0, 0, 0, 0, 0, 0, 0, 0, 0, 0, 0, 0, 0, 0, 0, 0, 0, 0, 0, 0, 0, 0, 0, 0, 0, 0, 0, 0, 0, 0, 0, 0, 0, 0, 0, 0, 0, 0, 0, 0, 0, 0, 0, 0, 0, 0, 0, 0, 0, 0, 0, 0, 0, 0, 0, 0, 0, 0, 0, 0, 0, 0, 0, 0, 0, 0, 0, 0, 0, 0, 0, 0, 0, 0, 0, 0, 0, 0, 0, 0, 0, 0, 0, 0, 0, 0, 0, 0, 0, 0, 0, 0, 0, 0, 0, 0, 0, 0, 0, 0, 0, 0, 0, 0, 0, 0, 0, 0, 0, 0, 0, 0, 0, 0, 0, 0, 0, 0, 0, 0, 0, 0, 0, 0, 0, 0, 0, 0, 0, 0, 0, 0, 0, 0, 0, 0, 0, 0, 0, 0, 0, 0, 0, 0, 0, 0, 0, 0, 0, 0, 0, 0, 0, 0, 0, 0, 0, 0, 0, 0, 0, 0, 0, 0, 0, 0, 0, 0, 0, 0, 0, 0, 0, 0, 0, 0, 0, 0, 0, 0, 0, 0, 0, 0, 0, 0, 0, 0, 0, 0, 0, 0, 0, 0, 0, 0, 0, 0, 0, 0, 0, 0, 0, 0, 0, 0, 0, 0, 0, 0, 0, 0, 0, 0, 0, 0, 0, 0, 0, 0, 0, 0, 0, 0, 0, 0, 0, 0, 0, 0, 0, 0, 0, 0, 0, 0, 0, 0, 0, 0, 0, 0, 0, 0, 0, 0, 0, 0, 0, 0, 0, 0, 0, 0, 0, 0, 0, 0, 0, 0, 0, 0, 0, 0, 0, 0, 0, 0, 0, 0, 0, 0, 0, 0, 0, 0, 0, 0, 0, 0, 0, 0, 0, 0, 0, 0, 0, 0, 0, 0, 0, 0, 0, 0, 0, 0, 0, 0, 0, 0, 0, 0, 0, 0, 0, 0, 0, 0, 0, 0, 0, 0, 0, 0, 0, 0, 0, 0, 0, 0, 0, 0, 0, 0, 0, 0, 0, 0, 0, 0, 0, 0, 0, 0, 0, 0, 0, 0, 0, 0, 0, 0, 0, 0, 0, 0, 0, 0, 0, 0, 0, 0, 0, 0, 0, 0, 0, 0, 0, 0, 0, 0, 0, 0, 0, 0, 0, 0, 0, 0, 0, 0, 0, 0, 0, 0, 0, 0, 0, 0, 0, 0, 0, 0, 0, 0, 0, 0, 0, 0, 0, 0, 0, 0, 0, 0, 0, 0, 0, 0, 0, 0, 0, 0, 0, 0, 0, 0, 0, 0, 0, 0, 0, 0, 0, 0, 0, 0, 0, 0, 0, 0, 0, 0, 0, 0, 0, 0, 0, 0, 0, 0, 0, 0, 0, 0, 0, 0, 0, 0, 0, 0, 0, 0, 0, 0, 0, 0, 0, 0, 0, 0, 0, 0, 0, 0, 0, 0, 0, 0, 0, 0, 0, 0, 0, 0, 0, 0, 0, 0, 0, 0, 0, 0, 0, 0, 0, 0, 0, 0, 0, 0, 0, 0, 0, 0, 0, 0, 0, 0, 0, 0, 0, 0, 0, 0, 0, 0, 0, 0, 0, 0, 0, 0, 0, 0, 0, 0, 0, 0, 0, 0, 0, 0, 0, 0, 0, 0, 0, 0, 0, 0, 0, 0, 0, 0, 0, 0, 0, 0, 0, 0, 0, 0, 0, 0, 0, 0, 0, 0, 0, 0, 0, 0, 0, 0, 0, 0, 0, 0, 0, 0, 0, 0, 0, 0, 0, 0, 0, 0, 0, 0, 0, 0, 0, 0, 0, 0, 0, 0, 0, 0, 0, 0, 0, 0, 0, 0, 0, 0, 0, 0, 0, 0, 0, 0, 0, 0, 0, 0, 0, 0, 0, 0, 0, 0, 0, 0, 0, 0, 0, 0, 0, 0, 0, 0, 0, 0, 0, 0, 0, 0, 0, 0, 0, 0, 0, 0, 0, 0, 0, 0, 0, 0, 0, 0, 0, 0, 0, 0, 0, 0, 0, 0, 0, 0, 0, 0, 0, 0, 0, 0, 0, 0, 0, 0, 0, 0, 0, 0, 0, 0, 0, 0, 0, 0, 0, 0, 0, 0, 0, 0, 0, 0, 0, 0, 0, 0, 0, 0, 0, 0, 0, 0, 0, 0, 0, 0, 0, 0, 0, 0, 0, 0, 0, 0, 0, 0, 0, 0, 0, 0, 0, 0, 0, 0, 0, 0, 0, 0, 0, 0, 0, 0, 0, 0, 0, 0, 0, 0, 0, 0, 0, 0, 0, 0, 0, 0, 0, 0, 0, 0, 0, 0, 0, 0, 0, 0, 0, 0, 0, 0, 0, 0, 0, 0, 0, 0, 0, 0, 0, 0, 0, 0, 0, 0, 0, 0, 0, 0, 0, 0, 0, 0, 0, 0, 0, 0, 0, 0, 0, 0, 0, 0, 0, 0, 0, 0, 0, 0, 0, 0, 0, 0, 0, 0, 0, 0, 0, 0, 0, 0, 0, 0, 0, 0, 0, 0, 0, 0, 0, 0, 0, 0, 0, 0, 0, 0, 0, 0, 0, 0, 0, 0, 0, 0, 0, 0, 0, 0, 0, 0, 0, 0, 0, 0, 0, 0, 0, 0, 0, 0, 0, 0, 0, 0, 0, 0, 0, 0, 0, 0, 0, 0, 0, 0, 0, 0, 0, 0, 0, 0, 0, 0, 0, 0, 0, 0, 0, 0, 0, 0, 0, 0, 0, 0, 0, 0, 0, 0, 0, 0, 0, 0, 0, 0, 0, 0, 0, 0, 0, 0, 0, 0, 0, 0, 0, 0, 0, 0, 0, 0, 0, 0, 0, 0, 0, 0, 0, 0, 0, 0, 0, 0, 0, 0, 0, 0, 0, 0, 0, 0, 0, 0, 0, 0, 0, 0, 0, 0, 0, 0, 0, 0, 0, 0, 0, 0, 0, 0, 0, 0, 0, 0, 0, 0, 0, 0, 0, 0, 0, 0, 0, 0, 0, 0, 0, 0, 0, 0, 0, 0, 0, 0, 0, 0, 0, 0, 0, 0, 0, 0, 0, 0, 0, 0, 0, 0, 0, 0, 0, 0, 0, 0, 0, 0, 0, 0, 0, 0, 0, 0, 0, 0, 0, 0, 0, 0, 0, 0, 0, 0, 0, 0, 0, 0, 0, 0, 0, 0, 0, 0, 0, 0, 0, 0, 0, 0, 0, 0, 0, 0, 0, 0, 0, 0, 0, 0, 0, 0, 0, 0, 0, 0, 0, 0, 0, 0, 0, 0, 0, 0, 0, 0, 0, 0, 0, 0, 0, 0, 0, 0, 0, 0, 0, 0, 0, 0, 0, 0, 0, 0, 0, 0, 0, 0, 0, 0, 0, 0, 0, 0, 0, 0, 0, 0, 0, 0, 0, 0, 0, 0, 0, 0, 0, 0, 0, 0, 0, 0, 0, 0, 0, 0, 0, 0, 0, 0, 0, 0, 0, 0, 0, 0, 0, 0, 0, 0, 0, 0, 0, 0, 0, 0, 0, 0, 0, 0, 0, 0, 0, 0, 0, 0, 0, 0, 0, 0, 0, 0, 0, 0, 0, 0, 0, 0, 0, 0, 0, 0, 0, 0, 0, 0, 0, 0, 0, 0, 0, 0, 0, 0, 0, 0, 0, 0, 0, 0, 0, 0, 0, 0, 0, 0, 0, 0, 0, 0, 0, 0, 0, 0, 0, 0, 0, 0, 0, 0, 0, 0, 0, 0, 0, 0, 0, 0, 0, 0, 0, 0, 0, 0, 0, 0, 0, 0, 0, 0, 0, 0, 0, 0, 0, 0, 0, 0, 0, 0, 0, 0, 0, 0, 0, 0, 0, 0, 0, 0, 0, 0, 0, 0, 0, 0, 0, 0, 0, 0, 0, 0, 0, 0, 0, 0, 0, 0, 0, 0, 0, 0, 0, 0, 0, 0, 0, 0, 0, 0, 0, 0, 0, 0, 0, 0, 0, 0, 0, 0, 0, 0, 0, 0, 0, 0, 0, 0, 0, 0, 0, 0, 0, 0, 0, 0, 0, 0, 0, 0, 0, 0, 0, 0, 0, 0, 0, 0, 0, 0, 0, 0, 0, 0, 0, 0, 0, 0, 0, 0, 0, 0, 0, 0, 0, 0, 0, 0, 0, 0, 0, 0, 0, 0, 0, 0, 0, 0, 0, 0, 0, 0, 0, 0, 0, 0, 0, 0, 0, 0, 0, 0, 0, 0, 0, 0, 0, 0, 0, 0, 0, 0, 0, 0, 0, 0, 0, 0, 0, 0, 0, 0, 0, 0, 0, 0, 0, 0, 0, 0, 0, 0, 0, 0, 0, 0, 0, 0, 0, 0, 0, 0, 0, 0, 0, 0, 0, 0, 0, 0, 0, 0, 0, 0, 0, 0, 0, 0, 0, 0, 0, 0, 0, 0, 0, 0, 0, 0, 0, 0, 0, 0, 0, 0, 0, 0, 0, 0, 0, 0, 0, 0, 0, 0, 0, 0, 0, 0, 0, 0, 0, 0, 0, 0, 0, 0, 0, 0, 0, 0, 0, 0, 0, 0, 0, 0, 0, 0, 0, 0, 0, 0, 0, 0, 0, 0, 0, 0, 0, 0, 0, 0, 0, 0, 0, 0, 0, 0, 0, 0, 0, 0, 0, 0, 0, 0, 0, 0, 0, 0, 0, 0, 0, 0, 0, 0, 0, 0, 0, 0, 0, 0, 0, 0, 0, 0, 0, 0, 0, 0, 0, 0, 0, 0, 0, 0, 0, 0, 0, 0, 0, 0, 0, 0, 0, 0, 0, 0, 0, 0, 0, 0, 0, 0, 0, 0, 0, 0, 0, 0, 0, 0, 0, 0, 0, 0, 0, 0, 0, 0, 0, 0, 0, 0, 0, 0, 0, 0, 0, 0, 0, 0, 0, 0, 0, 0, 0, 0, 0, 0, 0, 0, 0, 0, 0, 0, 0, 0, 0, 0, 0, 0, 0, 0, 0, 0, 0, 0, 0, 0, 0, 0, 0, 0, 0, 0, 0, 0, 0, 0, 0, 0, 0, 0, 0, 0, 0, 0, 0, 0, 0, 0, 0, 0, 0, 0, 0, 0, 0, 0, 0, 0, 0, 0, 0, 0, 0, 0, 0, 0, 0, 0, 0, 0, 0, 0, 0, 0, 0, 0, 0, 0, 0, 0, 0, 0, 0, 0, 0, 0, 0, 0, 0, 0, 0, 0, 0, 0, 0, 0, 0, 0, 0, 0, 0, 0, 0, 0, 0, 0, 0, 0, 0, 0, 0, 0, 0, 0, 0, 0, 0, 0, 0, 0, 0, 0, 0, 0, 0, 0, 0, 0, 0, 0, 0, 0, 0, 0, 0, 0, 0, 0, 0, 0, 0, 0, 0, 0, 0, 0, 0, 0, 0, 0, 0, 0, 0, 0, 0, 0, 0, 0, 0, 0, 0, 0, 0, 0, 0, 0, 0, 0, 0, 0, 0, 0, 0, 0, 0, 0, 0, 0, 0, 0, 0, 0, 0, 0, 0, 0, 0, 0, 0, 0, 0, 0, 0, 0, 0, 0, 0, 0, 0, 0, 0, 0, 0, 0, 0, 0, 0, 0, 0, 0, 0, 0, 0, 0, 0, 0, 0, 0, 0, 0, 0, 0, 0, 0, 0, 0, 0, 0, 0, 0, 0, 0, 0, 0, 0, 0, 0, 0, 0, 0, 0, 0, 0, 0, 0, 0, 0, 0, 0, 0, 0, 0, 0, 0, 0, 0, 0, 0, 0, 0, 0, 0, 0, 0, 0, 0, 0, 0, 0, 0, 0, 0, 0, 0, 0, 0, 0, 0, 0, 0, 0, 0, 0, 0, 0, 0, 0, 0, 0, 0, 0, 0, 0, 0, 0, 0, 0, 0, 0, 0, 0, 0, 0, 0, 0, 0, 0, 0, 0, 0, 0, 0, 0, 0, 0, 0, 0, 0, 0, 0, 0, 0, 0, 0, 0, 0, 0, 0, 0, 0, 0, 0, 0, 0, 0, 0, 0, 0, 0, 0, 0, 0, 0, 0, 0, 0, 0, 0, 0, 0, 0, 0, 0, 0, 0, 0, 0, 0, 0, 0, 0, 0, 0, 0, 0, 0, 0, 0, 0, 0, 0, 0, 0, 0, 0, 0, 0, 0, 0, 0, 0, 0, 0, 0, 0, 0, 0, 0, 0, 0, 0, 0, 0, 0, 0, 0, 0, 0, 0, 0, 0, 0, 0, 0, 0, 0, 0, 0, 0, 0, 0, 0, 0, 0, 0, 0, 0, 0, 0, 0, 0, 0, 0, 0, 0, 0, 0, 0, 0, 0, 0, 0, 0, 0, 0, 0, 0, 0, 0, 0, 0, 0, 0, 0, 0, 0, 0, 0, 0, 0, 0, 0, 0, 0, 0, 0, 0, 0, 0, 0, 0, 0, 0, 0, 0, 0, 0, 0, 0, 0, 0, 0, 0, 0, 0, 0, 0, 0, 0, 0, 0, 0, 0, 0, 0, 0, 0, 0, 0, 0, 0, 0, 0, 0, 0, 0, 0, 0, 0, 0, 0, 0, 0, 0, 0, 0, 0, 0, 0, 0, 0, 0, 0, 0, 0, 0, 0, 0, 0, 0, 0, 0, 0, 0, 0, 0, 0, 0, 0, 0, 0, 0, 0, 0, 0, 0, 0, 0, 0, 0, 0, 0, 0, 0, 0, 0, 0, 0, 0, 0, 0, 0, 0, 0, 0, 0, 0, 0, 0, 0, 0, 0, 0, 0, 0, 0, 0, 0, 0, 0, 0, 0, 0, 0, 0, 0, 0, 0, 0, 0, 0, 0, 0, 0, 0, 0, 0, 0, 0, 0, 0, 0, 0, 0, 0, 0, 0, 0, 0, 0, 0, 0, 0, 0, 0, 0, 0, 0, 0, 0, 0, 0, 0, 0, 0, 0, 0, 0, 0, 0, 0, 0, 0, 0, 0, 0, 0, 0, 0, 0, 0, 0, 0, 0, 0, 0, 0, 0, 0, 0, 0, 0, 0, 0, 0, 0, 0, 0, 0, 0, 0, 0, 0, 0, 0, 0, 0, 0, 0, 0, 0, 0, 0, 0, 0, 0, 0, 0, 0, 0, 0, 0, 0, 0, 0, 0, 0, 0, 0, 0, 0, 0, 0, 0, 0, 0, 0, 0, 0, 0, 0, 0, 0, 0, 0, 0, 0, 0, 0, 0, 0, 0, 0, 0, 0, 0, 0, 0, 0, 0, 0, 0, 0, 0, 0, 0, 0, 0, 0, 0, 0, 0, 0, 0, 0, 0, 0, 0, 0, 0, 0, 0, 0, 0, 0, 0, 0, 0, 0, 0, 0, 0, 0, 0, 0, 0, 0, 0, 0, 0, 0, 0, 0, 0, 0, 0, 0, 0, 0, 0, 0, 0, 0, 0, 0, 0, 0, 0, 0, 0, 0, 0, 0, 0, 0, 0, 0, 0, 0, 0, 0, 0, 0, 0, 0, 0, 0, 0, 0, 0, 0, 0, 0, 0, 0, 0, 0, 0, 0, 0, 0, 0, 0, 0, 0, 0, 0, 0, 0, 0, 0, 0, 0, 0, 0, 0, 0, 0, 0, 0, 0, 0, 0, 0, 0, 0, 0, 0, 0, 0, 0, 0, 0, 0, 0, 0, 0, 0, 0, 0, 0, 0, 0, 0, 0, 0, 0, 0, 0, 0, 0, 0, 0, 0, 0, 0, 0, 0, 0, 0, 0, 0, 0, 0, 0, 0, 0, 0, 0, 0, 0, 0, 0, 0, 0, 0, 0, 0, 0, 0, 0, 0, 0, 0, 0, 0, 0, 0, 0, 0, 0, 0, 0, 0, 0, 0, 0, 0, 0, 0, 0, 0, 0, 0, 0, 0, 0, 0, 0, 0, 0, 0, 0, 0, 0, 0, 0, 0, 0, 0, 0, 0, 0, 0, 0, 0, 0, 0, 0, 0, 0, 0, 0, 0, 0, 0, 0, 0, 0, 0, 0, 0, 0, 0, 0, 0, 0, 0, 0, 0, 0, 0, 0, 0, 0, 0, 0, 0, 0, 0, 0, 0, 0, 0, 0, 0, 0, 0, 0, 0, 0, 0, 0, 0, 0, 0, 0, 0, 0, 0, 0, 0, 0, 0, 0, 0, 0, 0, 0, 0, 0, 0, 0, 0, 0, 0, 0, 0, 0, 0, 0, 0, 0, 0, 0, 0, 0, 0, 0, 0, 0, 0, 0, 0, 0, 0, 0, 0, 0, 0, 0, 0, 0, 0, 0, 0, 0, 0, 0, 0, 0, 0, 0, 0, 0, 0, 0, 0, 0, 0, 0, 0, 0, 0, 0, 0, 0, 0, 0, 0, 0, 0, 0, 0, 0, 0, 0, 0, 0, 0, 0, 0, 0, 0, 0, 0, 0, 0, 0, 0, 0, 0, 0, 0, 0, 0, 0, 0, 0, 0, 0, 0, 0, 0, 0, 0, 0, 0, 0, 0, 0, 0, 0, 0, 0, 0, 0, 0, 0, 0, 0, 0, 0, 0, 0, 0, 0, 0, 0, 0, 0, 0, 0, 0, 0, 0, 0, 0, 0, 0, 0, 0, 0, 0, 0, 0, 0, 0, 0, 0, 0, 0, 0, 0, 0, 0, 0, 0, 0, 0, 0, 0, 0, 0, 0, 0, 0, 0, 0, 0, 0, 0, 0, 0, 0, 0, 0, 0, 0, 0, 0, 0, 0, 0, 0, 0, 0, 0, 0, 0, 0, 0, 0, 0, 0, 0, 0, 0, 0, 0, 0, 0, 0, 0, 0, 0, 0, 0, 0, 0, 0, 0, 0, 0, 0, 0, 0, 0, 0, 0, 0, 0, 0, 0, 0, 0, 0, 0, 0, 0, 0, 0, 0, 0, 0, 0, 0, 0, 0, 0, 0, 0, 0, 0, 0, 0, 0, 0, 0, 0, 0, 0, 0, 0, 0, 0, 0, 0, 0, 0, 0, 0, 0, 0, 0, 0, 0, 0, 0, 0, 0, 0, 0, 0, 0, 0, 0, 0, 0, 0, 0, 0, 0, 0, 0, 0, 0, 0, 0, 0, 0, 0, 0, 0, 0, 0, 0, 0, 0, 0, 0, 0, 0, 0, 0, 0, 0, 0, 0, 0, 0, 0, 0, 0, 0, 0, 0, 0, 0, 0, 0, 0, 0, 0, 0, 0, 0, 0, 0, 0, 0, 0, 0, 0, 0, 0, 0, 0, 0, 0, 0, 0, 0, 0, 0, 0, 0, 0, 0, 0, 0, 0, 0, 0, 0, 0, 0, 0, 0, 0, 0, 0, 0, 0, 0, 0, 0, 0, 0, 0, 0, 0, 0, 0, 0, 0, 0, 0, 0, 0, 0, 0, 0, 0, 0, 0, 0, 0, 0, 0, 0, 0, 0, 0, 0, 0, 0, 0, 0, 0, 0, 0]
  out "PASS FAIL":bool[][](array[boolean])=[[TRUE, TRUE, FALSE, FALSE, FALSE, FALSE, FALSE, FALSE, FALSE, FALSE, FALSE, FALSE, FALSE, FALSE, FALSE, FALSE], [TRUE, TRUE, FALSE, FALSE, FALSE, FALSE, FALSE, FALSE, FALSE, FALSE, FALSE, FALSE, FALSE, FALSE, FALSE, FALSE], [TRUE, TRUE, FALSE, FALSE, FALSE, FALSE, FALSE, FALSE, FALSE, FALSE, FALSE, FALSE, FALSE, FALSE, FALSE, FALSE], [TRUE, TRUE, FALSE, FALSE, FALSE, FALSE, FALSE, FALSE, FALSE, FALSE, FALSE, FALSE, FALSE, FALSE, FALSE, FALSE], [TRUE, TRUE, FALSE, FALSE, FALSE, FALSE, FALSE, FALSE, FALSE, FALSE, FALSE, FALSE, FALSE, FALSE, FALSE, FALSE], [TRUE, TRUE, FALSE, FALSE, FALSE, FALSE, FALSE, FALSE, FALSE, FALSE, FALSE, FALSE, FALSE, FALSE, FALSE, FALSE], [TRUE, TRUE, FALSE, FALSE, FALSE, FALSE, FALSE, FALSE, FALSE, FALSE, FALSE, FALSE, FALSE, FALSE, FALSE, FALSE], [TRUE, TRUE, FALSE, FALSE, FALSE, FALSE, FALSE, FALSE, FALSE, FALSE, FALSE, FALSE, FALSE, FALSE, FALSE, FALSE], [TRUE, TRUE, FALSE, FALSE, FALSE, FALSE, FALSE, FALSE, FALSE, FALSE, FALSE, FALSE, FALSE, FALSE, FALSE, FALSE], [TRUE, FALSE, FALSE, FALSE, FALSE, FALSE, FALSE, FALSE, FALSE, FALSE, FALSE, FALSE, FALSE, FALSE, FALSE, FALSE], [TRUE, TRUE, FALSE, FALSE, FALSE, FALSE, FALSE, FALSE, FALSE, FALSE, FALSE, FALSE, FALSE, FALSE, FALSE, FALSE], [TRUE, TRUE, FALSE, FALSE, FALSE, FALSE, FALSE, FALSE, FALSE, FALSE, FALSE, FALSE, FALSE, FALSE, FALSE, FALSE], [TRUE, TRUE, FALSE, FALSE, FALSE, FALSE, FALSE, FALSE, FALSE, FALSE, FALSE, FALSE, FALSE, FALSE, FALSE, FALSE], [TRUE, TRUE, FALSE, FALSE, FALSE, FALSE, FALSE, FALSE, FALSE, FALSE, FALSE, FALSE, FALSE, FALSE, FALSE, FALSE], [TRUE, TRUE, FALSE, FALSE, FALSE, FALSE, FALSE, FALSE, FALSE, FALSE, FALSE, FALSE, FALSE, FALSE, FALSE, FALSE], [TRUE, TRUE, FALSE, FALSE, FALSE, FALSE, FALSE, FALSE, FALSE, FALSE, FALSE, FALSE, FALSE, FALSE, FALSE, FALSE]]
  out "PEAK":dbl[][](array[numeric])=[[742.0, 742.0, 1534.0, 0.0, 0.0, 0.0, 0.0, 0.0, 0.0, 0.0, 0.0, 0.0, 0.0, 0.0, 0.0, 0.0], [767.0, 732.0, 1534.0, 0.0, 0.0, 0.0, 0.0, 0.0, 0.0, 0.0, 0.0, 0.0, 0.0, 0.0, 0.0, 0.0], [731.0, 745.0, 1530.0, 0.0, 0.0, 0.0, 0.0, 0.0, 0.0, 0.0, 0.0, 0.0, 0.0, 0.0, 0.0, 0.0], [767.0, 761.0, 1534.0, 0.0, 0.0, 0.0, 0.0, 0.0, 0.0, 0.0, 0.0, 0.0, 0.0, 0.0, 0.0, 0.0], [716.0, 734.0, 1460.0, 0.0, 0.0, 0.0, 0.0, 0.0, 0.0, 0.0, 0.0, 0.0, 0.0, 0.0, 0.0, 0.0], [747.0, 736.0, 1466.0, 0.0, 0.0, 0.0, 0.0, 0.0, 0.0, 0.0, 0.0, 0.0, 0.0, 0.0, 0.0, 0.0], [744.0, 734.0, 1468.0, 0.0, 0.0, 0.0, 0.0, 0.0, 0.0, 0.0, 0.0, 0.0, 0.0, 0.0, 0.0, 0.0], [769.0, 767.0, 1466.0, 0.0, 0.0, 0.0, 0.0, 0.0, 0.0, 0.0, 0.0, 0.0, 0.0, 0.0, 0.0, 0.0], [727.0, 767.0, 1414.0, 0.0, 0.0, 0.0, 0.0, 0.0, 0.0, 0.0, 0.0, 0.0, 0.0, 0.0, 0.0, 0.0], [767.0, 769.0, 1534.0, 0.0, 0.0, 0.0, 0.0, 0.0, 0.0, 0.0, 0.0, 0.0, 0.0, 0.0, 0.0, 0.0], [764.0, 777.0, 1442.0, 0.0, 0.0, 0.0, 0.0, 0.0, 0.0, 0.0, 0.0, 0.0, 0.0, 0.0, 0.0, 0.0], [767.0, 769.0, 1456.0, 0.0, 0.0, 0.0, 0.0, 0.0, 0.0, 0.0, 0.0, 0.0, 0.0, 0.0, 0.0, 0.0], [767.0, 767.0, 1546.0, 0.0, 0.0, 0.0, 0.0, 0.0, 0.0, 0.0, 0.0, 0.0, 0.0, 0.0, 0.0, 0.0], [767.0, 775.0, 1466.0, 0.0, 0.0, 0.0, 0.0, 0.0, 0.0, 0.0, 0.0, 0.0, 0.0, 0.0, 0.0, 0.0], [767.0, 766.0, 1450.0, 0.0, 0.0, 0.0, 0.0, 0.0, 0.0, 0.0, 0.0, 0.0, 0.0, 0.0, 0.0, 0.0], [767.0, 725.0, 1488.0, 0.0, 0.0, 0.0, 0.0, 0.0, 0.0, 0.0, 0.0, 0.0, 0.0, 0.0, 0.0, 0.0]] format="%#_6p"
  out "RMS":dbl[][](array[numeric])=[[298.5701670490024, 302.01439686629885, 269.1660046874997, 0.0, 0.0, 0.0, 0.0, 0.0, 0.0, 0.0, 0.0, 0.0, 0.0, 0.0, 0.0, 0.0], [296.32358986552646, 299.978665884578, 268.13383609370084, 0.0, 0.0, 0.0, 0.0, 0.0, 0.0, 0.0, 0.0, 0.0, 0.0, 0.0, 0.0, 0.0], [301.1295103744998, 304.33549026025577, 276.03736966372725, 0.0, 0.0, 0.0, 0.0, 0.0, 0.0, 0.0, 0.0, 0.0, 0.0, 0.0, 0.0, 0.0], [296.55524149157094, 302.7276161750227, 274.81246439064233, 0.0, 0.0, 0.0, 0.0, 0.0, 0.0, 0.0, 0.0, 0.0, 0.0, 0.0, 0.0, 0.0], [300.3116744391091, 304.40784093722453, 275.6037599363065, 0.0, 0.0, 0.0, 0.0, 0.0, 0.0, 0.0, 0.0, 0.0, 0.0, 0.0, 0.0, 0.0], [297.900330420298, 305.0327362592443, 252.25983070233167, 0.0, 0.0, 0.0, 0.0, 0.0, 0.0, 0.0, 0.0, 0.0, 0.0, 0.0, 0.0, 0.0], [297.73678723520777, 303.497552304539, 264.0280972044936, 0.0, 0.0, 0.0, 0.0, 0.0, 0.0, 0.0, 0.0, 0.0, 0.0, 0.0, 0.0, 0.0], [293.8196119756943, 303.4943153875992, 273.2726872616018, 0.0, 0.0, 0.0, 0.0, 0.0, 0.0, 0.0, 0.0, 0.0, 0.0, 0.0, 0.0, 0.0], [300.1502097503072, 302.99025318403187, 270.0357113226809, 0.0, 0.0, 0.0, 0.0, 0.0, 0.0, 0.0, 0.0, 0.0, 0.0, 0.0, 0.0, 0.0], [298.81556953562585, 300.4928974483008, 280.19507618025455, 0.0, 0.0, 0.0, 0.0, 0.0, 0.0, 0.0, 0.0, 0.0, 0.0, 0.0, 0.0, 0.0], [298.0870443658607, 300.4683479751603, 274.4267581087389, 0.0, 0.0, 0.0, 0.0, 0.0, 0.0, 0.0, 0.0, 0.0, 0.0, 0.0, 0.0, 0.0], [297.24491243063284, 301.56680948462514, 275.39640906313224, 0.0, 0.0, 0.0, 0.0, 0.0, 0.0, 0.0, 0.0, 0.0, 0.0, 0.0, 0.0, 0.0], [296.277621525914, 301.7890654303612, 270.8710420601697, 0.0, 0.0, 0.0, 0.0, 0.0, 0.0, 0.0, 0.0, 0.0, 0.0, 0.0, 0.0, 0.0], [292.1989253261964, 300.94942815438094, 263.86363666398046, 0.0, 0.0, 0.0, 0.0, 0.0, 0.0, 0.0, 0.0, 0.0, 0.0, 0.0, 0.0, 0.0], [294.8627337299674, 299.80813966409073, 269.67680487707395, 0.0, 0.0, 0.0, 0.0, 0.0, 0.0, 0.0, 0.0, 0.0, 0.0, 0.0, 0.0, 0.0], [294.41641733583265, 299.9396078283432, 268.81952042425917, 0.0, 0.0, 0.0, 0.0, 0.0, 0.0, 0.0, 0.0, 0.0, 0.0, 0.0, 0.0, 0.0]] format="%#_6p"
  out "MEAN":dbl[][](array[numeric])=[[775.5197467088818, 775.0851524745875, 1512.630228295284, 0.0, 0.0, 0.0, 0.0, 0.0, 0.0, 0.0, 0.0, 0.0, 0.0, 0.0, 0.0, 0.0], [783.0701549741709, 760.5734044325945, 1513.6223962672889, 0.0, 0.0, 0.0, 0.0, 0.0, 0.0, 0.0, 0.0, 0.0, 0.0, 0.0, 0.0, 0.0], [765.5607398766872, 779.3631061489751, 1550.23496083986, 0.0, 0.0, 0.0, 0.0, 0.0, 0.0, 0.0, 0.0, 0.0, 0.0, 0.0, 0.0, 0.0], [777.8606898850192, 794.9476753874354, 1512.9168471921346, 0.0, 0.0, 0.0, 0.0, 0.0, 0.0, 0.0, 0.0, 0.0, 0.0, 0.0, 0.0, 0.0], [747.9770038326945, 769.3799366772205, 1483.886685552408, 0.0, 0.0, 0.0, 0.0, 0.0, 0.0, 0.0, 0.0, 0.0, 0.0, 0.0, 0.0, 0.0], [762.0616563906016, 768.4532577903683, 1496.6902182969504, 0.0, 0.0, 0.0, 0.0, 0.0, 0.0, 0.0, 0.0, 0.0, 0.0, 0.0, 0.0, 0.0], [777.9161806365606, 764.7957007165472, 1463.2621229795034, 0.0, 0.0, 0.0, 0.0, 0.0, 0.0, 0.0, 0.0, 0.0, 0.0, 0.0, 0.0, 0.0], [782.8906848858524, 782.6598900183303, 1487.7260456590568, 0.0, 0.0, 0.0, 0.0, 0.0, 0.0, 0.0, 0.0, 0.0, 0.0, 0.0, 0.0, 0.0], [760.8618563572738, 780.6432261289785, 1432.384602566239, 0.0, 0.0, 0.0, 0.0, 0.0, 0.0, 0.0, 0.0, 0.0, 0.0, 0.0, 0.0, 0.0], [779.0978170304949, 800.7080486585569, 1522.2942842859522, 0.0, 0.0, 0.0, 0.0, 0.0, 0.0, 0.0, 0.0, 0.0, 0.0, 0.0, 0.0, 0.0], [793.2297950341609, 794.5810698216964, 1476.9321779703382, 0.0, 0.0, 0.0, 0.0, 0.0, 0.0, 0.0, 0.0, 0.0, 0.0, 0.0, 0.0, 0.0], [781.4139310114981, 784.02416263956, 1444.9031828028662, 0.0, 0.0, 0.0, 0.0, 0.0, 0.0, 0.0, 0.0, 0.0, 0.0, 0.0, 0.0, 0.0], [795.0498250291618, 798.5709048491918, 1537.3587735377437, 0.0, 0.0, 0.0, 0.0, 0.0, 0.0, 0.0, 0.0, 0.0, 0.0, 0.0, 0.0, 0.0], [785.8066988835194, 792.0828195300783, 1488.6458923512748, 0.0, 0.0, 0.0, 0.0, 0.0, 0.0, 0.0, 0.0, 0.0, 0.0, 0.0, 0.0, 0.0], [781.1281453091151, 798.5714047658723, 1476.8091984669222, 0.0, 0.0, 0.0, 0.0, 0.0, 0.0, 0.0, 0.0, 0.0, 0.0, 0.0, 0.0, 0.0], [784.6795534077654, 756.6367272121313, 1509.0164972504583, 0.0, 0.0, 0.0, 0.0, 0.0, 0.0, 0.0, 0.0, 0.0, 0.0, 0.0, 0.0, 0.0]] format="%#_6p"
  in  "START":bool
  in  "samples 6":i32=1000000 caption="Number  of samples"
  in  "FILE PATH 2":path=path "D:/Users/jfried/Desktop/New folder (18)"
  in  "FILE NAME 3":string="junk_test" caption="FILE NAME 2"
  in  "SAVE TO \nFILE 2":bool
  in  "stop 2":bool
  out "samples 5":u32=889304 caption="SAMPLES"
  in  "SYNC 2":bool
  in  "FREQ 2":u16=600
  in  "DLY 2":u8=255
  in  "AMPL 2":u8=31 format="%x"
  in  "Mean upper limit":dbl=800.0
  in  "Mean lower limit":dbl=710.0
  out "Store_Data 2":bool
  in  "s 11":bool=TRUE
  in  "write_string":bool
  out "SDI 2":u16=16 format="%x"
  out "rst":u16=2
  out "cs":u16=4
  out "ck":u16=8
  out "SDI":u16=1
  in  "OK Button 2":bool
  in  "Slide":u8(slide)=2 scale=0.0..7.0
  in  "channel":T2={"sts"=TRUE, "snc"=TRUE, "SG"=0, "ST"=3, "SDC"=FALSE, "SDF"=FALSE} {"ST" items=["0.5us", "1us", "2us", "3us"]; "SG" items=["4.7 mV/fC", "7.8 mV/fC", "14 mV/fC", "25 mV/fC"]}
  in  "CHANNEL 4":T3={"D_offset"=0, "PDSR"=TRUE, "PCSR"=TRUE, "slp"=FALSE, "tst"=FALSE} {"D_offset" items=["0", "1", "2", "3", "4", "5", "6", "7", "8", "9", "10", "11", "12", "13", "14", "15"]}
  in  "QUICK SET":bool
  in  "s 10":bool=TRUE
  in  "s 9":bool=TRUE
  in  "s 8":bool=TRUE
  in  "s 7":bool=TRUE
  in  "s 6":bool=TRUE
  in  "s 5":bool=TRUE
  in  "s 4":bool=TRUE
  in  "s 3":bool=TRUE
  in  "s 2":bool=TRUE
  in  "s":bool=TRUE
  in  "CHANNEL 3":T4(array[cluster])=[[{"D_offset"=0, "PDSR"=TRUE, "PCSR"=TRUE, "slp"=FALSE, "tst"=FALSE}, {"D_offset"=0, "PDSR"=TRUE, "PCSR"=TRUE, "slp"=FALSE, "tst"=FALSE}, {"D_offset"=0, "PDSR"=TRUE, "PCSR"=TRUE, "slp"=FALSE, "tst"=FALSE}, {"D_offset"=0, "PDSR"=TRUE, "PCSR"=TRUE, "slp"=FALSE, "tst"=FALSE}, {"D_offset"=0, "PDSR"=TRUE, "PCSR"=TRUE, "slp"=FALSE, "tst"=FALSE}, {"D_offset"=0, "PDSR"=TRUE, "PCSR"=TRUE, "slp"=FALSE, "tst"=FALSE}, {"D_offset"=0, "PDSR"=TRUE, "PCSR"=TRUE, "slp"=FALSE, "tst"=FALSE}, {"D_offset"=0, "PDSR"=TRUE, "PCSR"=TRUE, "slp"=FALSE, "tst"=FALSE}], [{"D_offset"=0, "PDSR"=TRUE, "PCSR"=TRUE, "slp"=FALSE, "tst"=FALSE}, {"D_offset"=0, "PDSR"=TRUE, "PCSR"=TRUE, "slp"=FALSE, "tst"=FALSE}, {"D_offset"=0, "PDSR"=TRUE, "PCSR"=TRUE, "slp"=FALSE, "tst"=FALSE}, {"D_offset"=0, "PDSR"=TRUE, "PCSR"=TRUE, "slp"=FALSE, "tst"=FALSE}, {"D_offset"=0, "PDSR"=TRUE, "PCSR"=TRUE, "slp"=FALSE, "tst"=FALSE}, {"D_offset"=0, "PDSR"=TRUE, "PCSR"=TRUE, "slp"=FALSE, "tst"=FALSE}, {"D_offset"=0, "PDSR"=TRUE, "PCSR"=TRUE, "slp"=FALSE, "tst"=FALSE}, {"D_offset"=0, "PDSR"=TRUE, "PCSR"=TRUE, "slp"=FALSE, "tst"=FALSE}], [{"D_offset"=0, "PDSR"=TRUE, "PCSR"=TRUE, "slp"=FALSE, "tst"=FALSE}, {"D_offset"=0, "PDSR"=TRUE, "PCSR"=TRUE, "slp"=FALSE, "tst"=FALSE}, {"D_offset"=0, "PDSR"=TRUE, "PCSR"=TRUE, "slp"=FALSE, "tst"=FALSE}, {"D_offset"=0, "PDSR"=TRUE, "PCSR"=TRUE, "slp"=FALSE, "tst"=FALSE}, {"D_offset"=0, "PDSR"=TRUE, "PCSR"=TRUE, "slp"=FALSE, "tst"=FALSE}, {"D_offset"=0, "PDSR"=TRUE, "PCSR"=TRUE, "slp"=FALSE, "tst"=FALSE}, {"D_offset"=0, "PDSR"=TRUE, "PCSR"=TRUE, "slp"=FALSE, "tst"=FALSE}, {"D_offset"=0, "PDSR"=TRUE, "PCSR"=TRUE, "slp"=FALSE, "tst"=FALSE}], [{"D_offset"=0, "PDSR"=TRUE, "PCSR"=TRUE, "slp"=FALSE, "tst"=FALSE}, {"D_offset"=0, "PDSR"=TRUE, "PCSR"=TRUE, "slp"=FALSE, "tst"=FALSE}, {"D_offset"=0, "PDSR"=TRUE, "PCSR"=TRUE, "slp"=FALSE, "tst"=FALSE}, {"D_offset"=0, "PDSR"=TRUE, "PCSR"=TRUE, "slp"=FALSE, "tst"=FALSE}, {"D_offset"=0, "PDSR"=TRUE, "PCSR"=TRUE, "slp"=FALSE, "tst"=FALSE}, {"D_offset"=0, "PDSR"=TRUE, "PCSR"=TRUE, "slp"=FALSE, "tst"=FALSE}, {"D_offset"=0, "PDSR"=TRUE, "PCSR"=TRUE, "slp"=FALSE, "tst"=FALSE}, {"D_offset"=0, "PDSR"=TRUE, "PCSR"=TRUE, "slp"=FALSE, "tst"=FALSE}], [{"D_offset"=0, "PDSR"=TRUE, "PCSR"=TRUE, "slp"=FALSE, "tst"=FALSE}, {"D_offset"=0, "PDSR"=TRUE, "PCSR"=TRUE, "slp"=FALSE, "tst"=FALSE}, {"D_offset"=0, "PDSR"=TRUE, "PCSR"=TRUE, "slp"=FALSE, "tst"=FALSE}, {"D_offset"=0, "PDSR"=TRUE, "PCSR"=TRUE, "slp"=FALSE, "tst"=FALSE}, {"D_offset"=0, "PDSR"=TRUE, "PCSR"=TRUE, "slp"=FALSE, "tst"=FALSE}, {"D_offset"=0, "PDSR"=TRUE, "PCSR"=TRUE, "slp"=FALSE, "tst"=FALSE}, {"D_offset"=0, "PDSR"=TRUE, "PCSR"=TRUE, "slp"=FALSE, "tst"=FALSE}, {"D_offset"=0, "PDSR"=TRUE, "PCSR"=TRUE, "slp"=FALSE, "tst"=FALSE}], [{"D_offset"=0, "PDSR"=TRUE, "PCSR"=TRUE, "slp"=FALSE, "tst"=FALSE}, {"D_offset"=0, "PDSR"=TRUE, "PCSR"=TRUE, "slp"=FALSE, "tst"=FALSE}, {"D_offset"=0, "PDSR"=TRUE, "PCSR"=TRUE, "slp"=FALSE, "tst"=FALSE}, {"D_offset"=0, "PDSR"=TRUE, "PCSR"=TRUE, "slp"=FALSE, "tst"=FALSE}, {"D_offset"=0, "PDSR"=TRUE, "PCSR"=TRUE, "slp"=FALSE, "tst"=FALSE}, {"D_offset"=0, "PDSR"=TRUE, "PCSR"=TRUE, "slp"=FALSE, "tst"=FALSE}, {"D_offset"=0, "PDSR"=TRUE, "PCSR"=TRUE, "slp"=FALSE, "tst"=FALSE}, {"D_offset"=0, "PDSR"=TRUE, "PCSR"=TRUE, "slp"=FALSE, "tst"=FALSE}], [{"D_offset"=0, "PDSR"=TRUE, "PCSR"=TRUE, "slp"=TRUE, "tst"=FALSE}, {"D_offset"=0, "PDSR"=TRUE, "PCSR"=TRUE, "slp"=FALSE, "tst"=FALSE}, {"D_offset"=0, "PDSR"=TRUE, "PCSR"=TRUE, "slp"=FALSE, "tst"=FALSE}, {"D_offset"=0, "PDSR"=TRUE, "PCSR"=TRUE, "slp"=FALSE, "tst"=FALSE}, {"D_offset"=0, "PDSR"=TRUE, "PCSR"=TRUE, "slp"=FALSE, "tst"=FALSE}, {"D_offset"=0, "PDSR"=TRUE, "PCSR"=TRUE, "slp"=FALSE, "tst"=FALSE}, {"D_offset"=0, "PDSR"=TRUE, "PCSR"=TRUE, "slp"=FALSE, "tst"=FALSE}, {"D_offset"=0, "PDSR"=TRUE, "PCSR"=TRUE, "slp"=FALSE, "tst"=FALSE}], [{"D_offset"=0, "PDSR"=TRUE, "PCSR"=TRUE, "slp"=FALSE, "tst"=FALSE}, {"D_offset"=0, "PDSR"=TRUE, "PCSR"=TRUE, "slp"=FALSE, "tst"=FALSE}, {"D_offset"=0, "PDSR"=TRUE, "PCSR"=TRUE, "slp"=FALSE, "tst"=FALSE}, {"D_offset"=0, "PDSR"=TRUE, "PCSR"=TRUE, "slp"=FALSE, "tst"=FALSE}, {"D_offset"=0, "PDSR"=TRUE, "PCSR"=TRUE, "slp"=FALSE, "tst"=FALSE}, {"D_offset"=0, "PDSR"=TRUE, "PCSR"=TRUE, "slp"=FALSE, "tst"=FALSE}, {"D_offset"=0, "PDSR"=TRUE, "PCSR"=TRUE, "slp"=FALSE, "tst"=FALSE}, {"D_offset"=0, "PDSR"=TRUE, "PCSR"=TRUE, "slp"=FALSE, "tst"=FALSE}], [{"D_offset"=0, "PDSR"=TRUE, "PCSR"=TRUE, "slp"=FALSE, "tst"=FALSE}, {"D_offset"=0, "PDSR"=TRUE, "PCSR"=TRUE, "slp"=FALSE, "tst"=FALSE}, {"D_offset"=0, "PDSR"=TRUE, "PCSR"=TRUE, "slp"=FALSE, "tst"=FALSE}, {"D_offset"=0, "PDSR"=TRUE, "PCSR"=TRUE, "slp"=FALSE, "tst"=FALSE}, {"D_offset"=0, "PDSR"=TRUE, "PCSR"=TRUE, "slp"=FALSE, "tst"=FALSE}, {"D_offset"=0, "PDSR"=TRUE, "PCSR"=TRUE, "slp"=FALSE, "tst"=FALSE}, {"D_offset"=0, "PDSR"=TRUE, "PCSR"=TRUE, "slp"=FALSE, "tst"=FALSE}, {"D_offset"=0, "PDSR"=TRUE, "PCSR"=TRUE, "slp"=FALSE, "tst"=FALSE}], [{"D_offset"=0, "PDSR"=TRUE, "PCSR"=TRUE, "slp"=FALSE, "tst"=FALSE}, {"D_offset"=0, "PDSR"=TRUE, "PCSR"=TRUE, "slp"=FALSE, "tst"=FALSE}, {"D_offset"=0, "PDSR"=TRUE, "PCSR"=TRUE, "slp"=FALSE, "tst"=FALSE}, {"D_offset"=0, "PDSR"=TRUE, "PCSR"=TRUE, "slp"=FALSE, "tst"=FALSE}, {"D_offset"=0, "PDSR"=TRUE, "PCSR"=TRUE, "slp"=FALSE, "tst"=FALSE}, {"D_offset"=0, "PDSR"=TRUE, "PCSR"=TRUE, "slp"=FALSE, "tst"=FALSE}, {"D_offset"=0, "PDSR"=TRUE, "PCSR"=TRUE, "slp"=FALSE, "tst"=FALSE}, {"D_offset"=0, "PDSR"=TRUE, "PCSR"=TRUE, "slp"=FALSE, "tst"=FALSE}], [{"D_offset"=0, "PDSR"=TRUE, "PCSR"=TRUE, "slp"=FALSE, "tst"=FALSE}, {"D_offset"=0, "PDSR"=TRUE, "PCSR"=TRUE, "slp"=FALSE, "tst"=FALSE}, {"D_offset"=0, "PDSR"=TRUE, "PCSR"=TRUE, "slp"=FALSE, "tst"=FALSE}, {"D_offset"=0, "PDSR"=TRUE, "PCSR"=TRUE, "slp"=FALSE, "tst"=FALSE}, {"D_offset"=0, "PDSR"=TRUE, "PCSR"=TRUE, "slp"=FALSE, "tst"=FALSE}, {"D_offset"=0, "PDSR"=TRUE, "PCSR"=TRUE, "slp"=FALSE, "tst"=FALSE}, {"D_offset"=0, "PDSR"=TRUE, "PCSR"=TRUE, "slp"=FALSE, "tst"=FALSE}, {"D_offset"=0, "PDSR"=TRUE, "PCSR"=TRUE, "slp"=FALSE, "tst"=FALSE}], [{"D_offset"=0, "PDSR"=TRUE, "PCSR"=TRUE, "slp"=FALSE, "tst"=FALSE}, {"D_offset"=0, "PDSR"=TRUE, "PCSR"=TRUE, "slp"=FALSE, "tst"=FALSE}, {"D_offset"=0, "PDSR"=TRUE, "PCSR"=TRUE, "slp"=FALSE, "tst"=FALSE}, {"D_offset"=0, "PDSR"=TRUE, "PCSR"=TRUE, "slp"=FALSE, "tst"=FALSE}, {"D_offset"=0, "PDSR"=TRUE, "PCSR"=TRUE, "slp"=FALSE, "tst"=FALSE}, {"D_offset"=0, "PDSR"=TRUE, "PCSR"=TRUE, "slp"=FALSE, "tst"=FALSE}, {"D_offset"=0, "PDSR"=TRUE, "PCSR"=TRUE, "slp"=FALSE, "tst"=FALSE}, {"D_offset"=0, "PDSR"=TRUE, "PCSR"=TRUE, "slp"=FALSE, "tst"=FALSE}], [{"D_offset"=0, "PDSR"=TRUE, "PCSR"=TRUE, "slp"=FALSE, "tst"=FALSE}, {"D_offset"=0, "PDSR"=TRUE, "PCSR"=TRUE, "slp"=FALSE, "tst"=FALSE}, {"D_offset"=0, "PDSR"=TRUE, "PCSR"=TRUE, "slp"=FALSE, "tst"=FALSE}, {"D_offset"=0, "PDSR"=TRUE, "PCSR"=TRUE, "slp"=FALSE, "tst"=FALSE}, {"D_offset"=0, "PDSR"=TRUE, "PCSR"=TRUE, "slp"=FALSE, "tst"=FALSE}, {"D_offset"=0, "PDSR"=TRUE, "PCSR"=TRUE, "slp"=FALSE, "tst"=FALSE}, {"D_offset"=0, "PDSR"=TRUE, "PCSR"=TRUE, "slp"=FALSE, "tst"=FALSE}, {"D_offset"=0, "PDSR"=TRUE, "PCSR"=TRUE, "slp"=FALSE, "tst"=FALSE}], [{"D_offset"=0, "PDSR"=TRUE, "PCSR"=TRUE, "slp"=FALSE, "tst"=FALSE}, {"D_offset"=0, "PDSR"=TRUE, "PCSR"=TRUE, "slp"=FALSE, "tst"=FALSE}, {"D_offset"=0, "PDSR"=TRUE, "PCSR"=TRUE, "slp"=FALSE, "tst"=FALSE}, {"D_offset"=0, "PDSR"=TRUE, "PCSR"=TRUE, "slp"=FALSE, "tst"=FALSE}, {"D_offset"=0, "PDSR"=TRUE, "PCSR"=TRUE, "slp"=FALSE, "tst"=FALSE}, {"D_offset"=0, "PDSR"=TRUE, "PCSR"=TRUE, "slp"=FALSE, "tst"=FALSE}, {"D_offset"=0, "PDSR"=TRUE, "PCSR"=TRUE, "slp"=FALSE, "tst"=FALSE}, {"D_offset"=0, "PDSR"=TRUE, "PCSR"=TRUE, "slp"=FALSE, "tst"=FALSE}], [{"D_offset"=0, "PDSR"=TRUE, "PCSR"=TRUE, "slp"=FALSE, "tst"=FALSE}, {"D_offset"=0, "PDSR"=TRUE, "PCSR"=TRUE, "slp"=FALSE, "tst"=FALSE}, {"D_offset"=0, "PDSR"=TRUE, "PCSR"=TRUE, "slp"=FALSE, "tst"=FALSE}, {"D_offset"=0, "PDSR"=TRUE, "PCSR"=TRUE, "slp"=FALSE, "tst"=FALSE}, {"D_offset"=0, "PDSR"=TRUE, "PCSR"=TRUE, "slp"=FALSE, "tst"=FALSE}, {"D_offset"=0, "PDSR"=TRUE, "PCSR"=TRUE, "slp"=FALSE, "tst"=FALSE}, {"D_offset"=0, "PDSR"=TRUE, "PCSR"=TRUE, "slp"=FALSE, "tst"=FALSE}, {"D_offset"=0, "PDSR"=TRUE, "PCSR"=TRUE, "slp"=FALSE, "tst"=FALSE}], [{"D_offset"=0, "PDSR"=TRUE, "PCSR"=TRUE, "slp"=FALSE, "tst"=FALSE}, {"D_offset"=0, "PDSR"=TRUE, "PCSR"=TRUE, "slp"=FALSE, "tst"=FALSE}, {"D_offset"=0, "PDSR"=TRUE, "PCSR"=TRUE, "slp"=FALSE, "tst"=FALSE}, {"D_offset"=0, "PDSR"=TRUE, "PCSR"=TRUE, "slp"=FALSE, "tst"=FALSE}, {"D_offset"=0, "PDSR"=TRUE, "PCSR"=TRUE, "slp"=FALSE, "tst"=FALSE}, {"D_offset"=0, "PDSR"=TRUE, "PCSR"=TRUE, "slp"=FALSE, "tst"=FALSE}, {"D_offset"=0, "PDSR"=TRUE, "PCSR"=TRUE, "slp"=FALSE, "tst"=FALSE}, {"D_offset"=0, "PDSR"=TRUE, "PCSR"=TRUE, "slp"=FALSE, "tst"=FALSE}]] {"D_offset" items=["0", "1", "2", "3", "4", "5", "6", "7", "8", "9", "10", "11", "12", "13", "14", "15"]}
  out "ADC ARRAY":bool[](array[boolean])=[FALSE, FALSE, TRUE, TRUE, FALSE, FALSE, FALSE, FALSE, FALSE, FALSE, TRUE, TRUE, FALSE, FALSE, FALSE, FALSE, FALSE, FALSE, TRUE, TRUE, FALSE, FALSE, FALSE, FALSE, FALSE, FALSE, TRUE, TRUE, FALSE, FALSE, FALSE, FALSE, FALSE, FALSE, TRUE, TRUE, FALSE, FALSE, FALSE, FALSE, FALSE, FALSE, TRUE, TRUE, FALSE, FALSE, FALSE, FALSE, FALSE, FALSE, TRUE, TRUE, FALSE, FALSE, FALSE, FALSE, FALSE, FALSE, TRUE, TRUE, FALSE, FALSE, FALSE, FALSE, FALSE, FALSE, TRUE, TRUE, FALSE, FALSE, FALSE, FALSE, FALSE, TRUE, TRUE, TRUE, FALSE, FALSE, FALSE, FALSE, FALSE, FALSE, TRUE, TRUE, FALSE, FALSE, FALSE, FALSE, FALSE, FALSE, TRUE, TRUE, FALSE, FALSE, FALSE, FALSE, FALSE, FALSE, TRUE, TRUE, FALSE, FALSE, FALSE, FALSE, FALSE, FALSE, TRUE, TRUE, FALSE, FALSE, FALSE, FALSE, FALSE, FALSE, TRUE, TRUE, FALSE, FALSE, FALSE, FALSE, FALSE, FALSE, TRUE, TRUE, FALSE, FALSE, FALSE, FALSE, TRUE, FALSE, TRUE, FALSE, TRUE, TRUE, FALSE, FALSE, TRUE, FALSE, FALSE, TRUE, TRUE, FALSE, FALSE, FALSE, FALSE, FALSE, FALSE, TRUE, TRUE, FALSE, FALSE, FALSE, FALSE, FALSE, FALSE, TRUE, TRUE, FALSE, FALSE, FALSE, FALSE, FALSE, FALSE, TRUE, TRUE, FALSE, FALSE, FALSE, FALSE, FALSE, FALSE, TRUE, TRUE, FALSE, FALSE, FALSE, FALSE, FALSE, FALSE, TRUE, TRUE, FALSE, FALSE, FALSE, FALSE, FALSE, FALSE, TRUE, TRUE, FALSE, FALSE, FALSE, FALSE, FALSE, FALSE, TRUE, TRUE, FALSE, FALSE, FALSE, FALSE, FALSE, FALSE, TRUE, TRUE, FALSE, FALSE, FALSE, FALSE, FALSE, FALSE, TRUE, TRUE, FALSE, FALSE, FALSE, FALSE, FALSE, FALSE, TRUE, TRUE, FALSE, FALSE, FALSE, FALSE, FALSE, FALSE, TRUE, TRUE, FALSE, FALSE, FALSE, FALSE, FALSE, FALSE, TRUE, TRUE, FALSE, FALSE, FALSE, FALSE, FALSE, FALSE, TRUE, TRUE, FALSE, FALSE, FALSE, FALSE, FALSE, FALSE, TRUE, TRUE, FALSE, FALSE, FALSE, FALSE, FALSE, FALSE, TRUE, TRUE, FALSE, FALSE, FALSE, FALSE, TRUE, FALSE, TRUE, FALSE, TRUE, TRUE, FALSE, FALSE, TRUE, FALSE, FALSE, TRUE, TRUE, FALSE, FALSE, FALSE, FALSE, FALSE, FALSE, TRUE, TRUE, FALSE, FALSE, FALSE, FALSE, FALSE, FALSE, TRUE, TRUE, FALSE, FALSE, FALSE, FALSE, FALSE, FALSE, TRUE, TRUE, FALSE, FALSE, FALSE, FALSE, FALSE, FALSE, TRUE, TRUE, FALSE, FALSE, FALSE, FALSE, FALSE, FALSE, TRUE, TRUE, FALSE, FALSE, FALSE, FALSE, FALSE, FALSE, TRUE, TRUE, FALSE, FALSE, FALSE, FALSE, FALSE, FALSE, TRUE, TRUE, FALSE, FALSE, FALSE, FALSE, FALSE, FALSE, TRUE, TRUE, FALSE, FALSE, FALSE, FALSE, FALSE, FALSE, TRUE, TRUE, FALSE, FALSE, FALSE, FALSE, FALSE, FALSE, TRUE, TRUE, FALSE, FALSE, FALSE, FALSE, FALSE, FALSE, TRUE, TRUE, FALSE, FALSE, FALSE, FALSE, FALSE, FALSE, TRUE, TRUE, FALSE, FALSE, FALSE, FALSE, FALSE, FALSE, TRUE, TRUE, FALSE, FALSE, FALSE, FALSE, FALSE, FALSE, TRUE, TRUE, FALSE, FALSE, FALSE, FALSE, FALSE, FALSE, TRUE, TRUE, FALSE, FALSE, FALSE, FALSE, TRUE, FALSE, TRUE, FALSE, TRUE, TRUE, FALSE, FALSE, TRUE, FALSE, FALSE, TRUE, TRUE, FALSE, FALSE, FALSE, FALSE, FALSE, FALSE, TRUE, TRUE, FALSE, FALSE, FALSE, FALSE, FALSE, FALSE, TRUE, TRUE, FALSE, FALSE, FALSE, FALSE, FALSE, FALSE, TRUE, TRUE, FALSE, FALSE, FALSE, FALSE, FALSE, FALSE, TRUE, TRUE, FALSE, FALSE, FALSE, FALSE, FALSE, FALSE, TRUE, TRUE, FALSE, FALSE, FALSE, FALSE, FALSE, FALSE, TRUE, TRUE, FALSE, FALSE, FALSE, FALSE, FALSE, FALSE, TRUE, TRUE, FALSE, FALSE, FALSE, FALSE, FALSE, FALSE, TRUE, TRUE, FALSE, FALSE, FALSE, FALSE, FALSE, FALSE, TRUE, TRUE, FALSE, FALSE, FALSE, FALSE, FALSE, FALSE, TRUE, TRUE, FALSE, FALSE, FALSE, FALSE, FALSE, FALSE, TRUE, TRUE, FALSE, FALSE, FALSE, FALSE, FALSE, FALSE, TRUE, TRUE, FALSE, FALSE, FALSE, FALSE, FALSE, FALSE, TRUE, TRUE, FALSE, FALSE, FALSE, FALSE, FALSE, FALSE, TRUE, TRUE, FALSE, FALSE, FALSE, FALSE, FALSE, FALSE, TRUE, TRUE, FALSE, FALSE, FALSE, FALSE, TRUE, FALSE, TRUE, FALSE, TRUE, TRUE, FALSE, FALSE, TRUE, FALSE, FALSE, TRUE, TRUE, FALSE, FALSE, FALSE, FALSE, FALSE, FALSE, TRUE, TRUE, FALSE, FALSE, FALSE, FALSE, FALSE, FALSE, TRUE, TRUE, FALSE, FALSE, FALSE, FALSE, FALSE, FALSE, TRUE, TRUE, FALSE, FALSE, FALSE, FALSE, FALSE, FALSE, TRUE, TRUE, FALSE, FALSE, FALSE, FALSE, FALSE, FALSE, TRUE, TRUE, FALSE, FALSE, FALSE, FALSE, FALSE, FALSE, TRUE, TRUE, FALSE, FALSE, FALSE, FALSE, FALSE, FALSE, TRUE, TRUE, FALSE, FALSE, FALSE, FALSE, FALSE, FALSE, TRUE, TRUE, FALSE, FALSE, FALSE, FALSE, FALSE, FALSE, TRUE, TRUE, FALSE, FALSE, FALSE, FALSE, FALSE, FALSE, TRUE, TRUE, FALSE, FALSE, FALSE, FALSE, FALSE, FALSE, TRUE, TRUE, FALSE, FALSE, FALSE, FALSE, FALSE, FALSE, TRUE, TRUE, FALSE, FALSE, FALSE, FALSE, FALSE, FALSE, TRUE, TRUE, FALSE, FALSE, FALSE, FALSE, FALSE, FALSE, TRUE, TRUE, FALSE, FALSE, FALSE, FALSE, FALSE, FALSE, TRUE, TRUE, FALSE, FALSE, FALSE, FALSE, TRUE, FALSE, TRUE, FALSE, TRUE, TRUE, FALSE, FALSE, TRUE, FALSE, FALSE, TRUE, TRUE, FALSE, FALSE, FALSE, FALSE, FALSE, FALSE, TRUE, TRUE, FALSE, FALSE, FALSE, FALSE, FALSE, FALSE, TRUE, TRUE, FALSE, FALSE, FALSE, FALSE, FALSE, FALSE, TRUE, TRUE, FALSE, FALSE, FALSE, FALSE, FALSE, FALSE, TRUE, TRUE, FALSE, FALSE, FALSE, FALSE, FALSE, FALSE, TRUE, TRUE, FALSE, FALSE, FALSE, FALSE, FALSE, FALSE, TRUE, TRUE, FALSE, FALSE, FALSE, FALSE, FALSE, FALSE, TRUE, TRUE, FALSE, FALSE, FALSE, FALSE, FALSE, FALSE, TRUE, TRUE, FALSE, FALSE, FALSE, FALSE, FALSE, FALSE, TRUE, TRUE, FALSE, FALSE, FALSE, FALSE, FALSE, FALSE, TRUE, TRUE, FALSE, FALSE, FALSE, FALSE, FALSE, FALSE, TRUE, TRUE, FALSE, FALSE, FALSE, FALSE, FALSE, FALSE, TRUE, TRUE, FALSE, FALSE, FALSE, FALSE, FALSE, FALSE, TRUE, TRUE, FALSE, FALSE, FALSE, FALSE, FALSE, FALSE, TRUE, TRUE, FALSE, FALSE, FALSE, FALSE, FALSE, FALSE, TRUE, TRUE, FALSE, FALSE, FALSE, FALSE, TRUE, FALSE, TRUE, FALSE, TRUE, TRUE, FALSE, FALSE, TRUE, FALSE, FALSE, TRUE, TRUE, FALSE, FALSE, FALSE, FALSE, FALSE, FALSE, TRUE, TRUE, FALSE, FALSE, FALSE, FALSE, FALSE, FALSE, TRUE, TRUE, FALSE, FALSE, FALSE, FALSE, FALSE, FALSE, TRUE, TRUE, FALSE, FALSE, FALSE, FALSE, FALSE, FALSE, TRUE, TRUE, FALSE, FALSE, FALSE, FALSE, FALSE, FALSE, TRUE, TRUE, FALSE, FALSE, FALSE, FALSE, FALSE, FALSE, TRUE, TRUE, FALSE, FALSE, FALSE, FALSE, FALSE, FALSE, TRUE, TRUE, FALSE, FALSE, FALSE, FALSE, FALSE, FALSE, TRUE, TRUE, FALSE, FALSE, FALSE, FALSE, FALSE, FALSE, TRUE, TRUE, FALSE, FALSE, FALSE, FALSE, FALSE, FALSE, TRUE, TRUE, FALSE, FALSE, FALSE, FALSE, FALSE, FALSE, TRUE, TRUE, FALSE, FALSE, FALSE, FALSE, FALSE, FALSE, TRUE, TRUE, FALSE, FALSE, FALSE, FALSE, FALSE, FALSE, TRUE, TRUE, FALSE, FALSE, FALSE, FALSE, FALSE, FALSE, TRUE, TRUE, FALSE, FALSE, FALSE, FALSE, FALSE, FALSE, TRUE, TRUE, FALSE, FALSE, FALSE, FALSE, TRUE, FALSE, TRUE, FALSE, TRUE, TRUE, FALSE, FALSE, TRUE, FALSE, FALSE, TRUE, TRUE, FALSE, FALSE, FALSE, FALSE, FALSE, FALSE, TRUE, TRUE, FALSE, FALSE, FALSE, FALSE, FALSE, FALSE, TRUE, TRUE, FALSE, FALSE, FALSE, FALSE, FALSE, FALSE, TRUE, TRUE, FALSE, FALSE, FALSE, FALSE, FALSE, FALSE, TRUE, TRUE, FALSE, FALSE, FALSE, FALSE, FALSE, FALSE, TRUE, TRUE, FALSE, FALSE, FALSE, FALSE, FALSE, FALSE, TRUE, TRUE, FALSE, FALSE, FALSE, FALSE, FALSE, FALSE, TRUE, TRUE, FALSE, FALSE, FALSE, FALSE, FALSE, FALSE, TRUE, TRUE, FALSE, FALSE, FALSE, FALSE, FALSE, FALSE, TRUE, TRUE, FALSE, FALSE, FALSE, FALSE, FALSE, FALSE, TRUE, TRUE, FALSE, FALSE, FALSE, FALSE, FALSE, FALSE, TRUE, TRUE, FALSE, FALSE, FALSE, FALSE, FALSE, FALSE, TRUE, TRUE, FALSE, FALSE, FALSE, FALSE, FALSE, FALSE, TRUE, TRUE, FALSE, FALSE, FALSE, FALSE, FALSE, FALSE, TRUE, TRUE, FALSE, FALSE, FALSE, FALSE, FALSE, FALSE, TRUE, TRUE, FALSE, FALSE, FALSE, FALSE, TRUE, FALSE, TRUE, FALSE, TRUE, TRUE, FALSE, FALSE, TRUE]
  out "FE ARRAY":bool[](array[boolean])=[FALSE, FALSE, FALSE, TRUE, FALSE, FALSE, TRUE, TRUE, FALSE, FALSE, FALSE, TRUE, FALSE, FALSE, TRUE, TRUE, FALSE, FALSE, FALSE, TRUE, FALSE, FALSE, TRUE, TRUE, FALSE, FALSE, FALSE, TRUE, FALSE, FALSE, TRUE, TRUE, FALSE, FALSE, FALSE, TRUE, FALSE, FALSE, TRUE, TRUE, FALSE, FALSE, FALSE, TRUE, FALSE, FALSE, TRUE, TRUE, FALSE, FALSE, FALSE, TRUE, FALSE, FALSE, TRUE, TRUE, FALSE, FALSE, FALSE, TRUE, FALSE, FALSE, TRUE, TRUE, FALSE, FALSE, FALSE, TRUE, FALSE, FALSE, TRUE, TRUE, FALSE, FALSE, FALSE, TRUE, FALSE, FALSE, TRUE, TRUE, FALSE, FALSE, FALSE, TRUE, FALSE, FALSE, TRUE, TRUE, FALSE, FALSE, FALSE, TRUE, FALSE, FALSE, TRUE, TRUE, FALSE, FALSE, FALSE, TRUE, FALSE, FALSE, TRUE, TRUE, FALSE, FALSE, FALSE, TRUE, FALSE, FALSE, TRUE, TRUE, FALSE, FALSE, FALSE, TRUE, FALSE, FALSE, TRUE, TRUE, FALSE, FALSE, FALSE, TRUE, FALSE, FALSE, TRUE, TRUE, FALSE, FALSE, FALSE, FALSE, FALSE, FALSE, FALSE, FALSE, FALSE, FALSE, FALSE, TRUE, FALSE, FALSE, TRUE, TRUE, FALSE, FALSE, FALSE, TRUE, FALSE, FALSE, TRUE, TRUE, FALSE, FALSE, FALSE, TRUE, FALSE, FALSE, TRUE, TRUE, FALSE, FALSE, FALSE, TRUE, FALSE, FALSE, TRUE, TRUE, FALSE, FALSE, FALSE, TRUE, FALSE, FALSE, TRUE, TRUE, FALSE, FALSE, FALSE, TRUE, FALSE, FALSE, TRUE, TRUE, FALSE, FALSE, FALSE, TRUE, FALSE, FALSE, TRUE, TRUE, FALSE, FALSE, FALSE, TRUE, FALSE, FALSE, TRUE, TRUE, FALSE, FALSE, FALSE, TRUE, FALSE, FALSE, TRUE, TRUE, FALSE, FALSE, FALSE, TRUE, FALSE, FALSE, TRUE, TRUE, FALSE, FALSE, FALSE, TRUE, FALSE, FALSE, TRUE, TRUE, FALSE, FALSE, FALSE, TRUE, FALSE, FALSE, TRUE, TRUE, FALSE, FALSE, FALSE, TRUE, FALSE, FALSE, TRUE, TRUE, FALSE, FALSE, FALSE, TRUE, FALSE, FALSE, TRUE, TRUE, FALSE, FALSE, FALSE, TRUE, FALSE, FALSE, TRUE, TRUE, FALSE, FALSE, FALSE, TRUE, FALSE, FALSE, TRUE, TRUE, FALSE, FALSE, FALSE, FALSE, FALSE, FALSE, FALSE, FALSE, FALSE, FALSE, TRUE, TRUE, FALSE, FALSE, TRUE, TRUE, FALSE, FALSE, TRUE, TRUE, FALSE, FALSE, TRUE, TRUE, FALSE, FALSE, TRUE, TRUE, FALSE, FALSE, TRUE, TRUE, FALSE, FALSE, TRUE, TRUE, FALSE, FALSE, TRUE, TRUE, FALSE, FALSE, TRUE, TRUE, FALSE, FALSE, TRUE, TRUE, FALSE, FALSE, TRUE, TRUE, FALSE, FALSE, TRUE, TRUE, FALSE, FALSE, TRUE, TRUE, FALSE, FALSE, TRUE, TRUE, FALSE, FALSE, TRUE, TRUE, FALSE, FALSE, TRUE, TRUE, FALSE, FALSE, TRUE, TRUE, FALSE, FALSE, TRUE, TRUE, FALSE, FALSE, TRUE, TRUE, FALSE, FALSE, TRUE, TRUE, FALSE, FALSE, TRUE, TRUE, FALSE, FALSE, TRUE, TRUE, FALSE, FALSE, TRUE, TRUE, FALSE, FALSE, TRUE, TRUE, FALSE, FALSE, TRUE, TRUE, FALSE, FALSE, TRUE, TRUE, FALSE, FALSE, TRUE, TRUE, FALSE, FALSE, TRUE, TRUE, FALSE, FALSE, TRUE, TRUE, FALSE, FALSE, TRUE, TRUE, FALSE, FALSE, TRUE, TRUE, FALSE, FALSE, TRUE, TRUE, FALSE, FALSE, FALSE, FALSE, FALSE, FALSE, FALSE, FALSE, FALSE, FALSE, TRUE, TRUE, FALSE, FALSE, TRUE, TRUE, FALSE, FALSE, TRUE, TRUE, FALSE, FALSE, TRUE, TRUE, FALSE, FALSE, TRUE, TRUE, FALSE, FALSE, TRUE, TRUE, FALSE, FALSE, TRUE, TRUE, FALSE, FALSE, TRUE, TRUE, FALSE, FALSE, TRUE, TRUE, FALSE, FALSE, TRUE, TRUE, FALSE, FALSE, TRUE, TRUE, FALSE, FALSE, TRUE, TRUE, FALSE, FALSE, TRUE, TRUE, FALSE, FALSE, TRUE, TRUE, FALSE, FALSE, TRUE, TRUE, FALSE, FALSE, TRUE, TRUE, FALSE, FALSE, TRUE, TRUE, FALSE, FALSE, TRUE, TRUE, FALSE, FALSE, TRUE, TRUE, FALSE, FALSE, TRUE, TRUE, FALSE, FALSE, TRUE, TRUE, FALSE, FALSE, TRUE, TRUE, FALSE, FALSE, TRUE, TRUE, FALSE, FALSE, TRUE, TRUE, FALSE, FALSE, TRUE, TRUE, FALSE, FALSE, TRUE, TRUE, FALSE, FALSE, TRUE, TRUE, FALSE, FALSE, TRUE, TRUE, FALSE, FALSE, TRUE, TRUE, FALSE, FALSE, TRUE, TRUE, FALSE, FALSE, TRUE, TRUE, FALSE, FALSE, TRUE, TRUE, FALSE, FALSE, FALSE, FALSE, FALSE, FALSE, FALSE, FALSE, FALSE, FALSE, FALSE, TRUE, FALSE, FALSE, TRUE, TRUE, FALSE, FALSE, FALSE, TRUE, FALSE, FALSE, TRUE, TRUE, FALSE, FALSE, FALSE, TRUE, FALSE, FALSE, TRUE, TRUE, FALSE, FALSE, FALSE, TRUE, FALSE, FALSE, TRUE, TRUE, FALSE, FALSE, FALSE, TRUE, FALSE, FALSE, TRUE, TRUE, FALSE, FALSE, FALSE, TRUE, FALSE, FALSE, TRUE, TRUE, FALSE, FALSE, FALSE, TRUE, FALSE, FALSE, TRUE, TRUE, FALSE, FALSE, FALSE, TRUE, FALSE, FALSE, TRUE, TRUE, FALSE, FALSE, FALSE, TRUE, FALSE, FALSE, TRUE, TRUE, FALSE, FALSE, FALSE, TRUE, FALSE, FALSE, TRUE, TRUE, FALSE, FALSE, FALSE, TRUE, FALSE, FALSE, TRUE, TRUE, FALSE, FALSE, FALSE, TRUE, FALSE, FALSE, TRUE, TRUE, FALSE, FALSE, FALSE, TRUE, FALSE, FALSE, TRUE, TRUE, FALSE, FALSE, FALSE, TRUE, FALSE, FALSE, TRUE, TRUE, FALSE, FALSE, FALSE, TRUE, FALSE, FALSE, TRUE, TRUE, FALSE, FALSE, FALSE, TRUE, FALSE, FALSE, TRUE, TRUE, FALSE, FALSE, FALSE, FALSE, FALSE, FALSE, FALSE, FALSE, FALSE, FALSE, FALSE, TRUE, FALSE, FALSE, TRUE, TRUE, FALSE, FALSE, FALSE, TRUE, FALSE, FALSE, TRUE, TRUE, FALSE, FALSE, FALSE, TRUE, FALSE, FALSE, TRUE, TRUE, FALSE, FALSE, FALSE, TRUE, FALSE, FALSE, TRUE, TRUE, FALSE, FALSE, FALSE, TRUE, FALSE, FALSE, TRUE, TRUE, FALSE, FALSE, FALSE, TRUE, FALSE, FALSE, TRUE, TRUE, FALSE, FALSE, FALSE, TRUE, FALSE, FALSE, TRUE, TRUE, FALSE, FALSE, FALSE, TRUE, FALSE, FALSE, TRUE, TRUE, FALSE, FALSE, FALSE, TRUE, FALSE, FALSE, TRUE, TRUE, FALSE, FALSE, FALSE, TRUE, FALSE, FALSE, TRUE, TRUE, FALSE, FALSE, FALSE, TRUE, FALSE, FALSE, TRUE, TRUE, FALSE, FALSE, FALSE, TRUE, FALSE, FALSE, TRUE, TRUE, FALSE, FALSE, FALSE, TRUE, FALSE, FALSE, TRUE, TRUE, FALSE, FALSE, FALSE, TRUE, FALSE, FALSE, TRUE, TRUE, FALSE, FALSE, FALSE, TRUE, FALSE, FALSE, TRUE, TRUE, FALSE, FALSE, FALSE, TRUE, FALSE, FALSE, TRUE, TRUE, FALSE, FALSE, FALSE, FALSE, FALSE, FALSE, FALSE, FALSE, FALSE, FALSE, FALSE, TRUE, FALSE, FALSE, TRUE, TRUE, FALSE, FALSE, FALSE, TRUE, FALSE, FALSE, TRUE, TRUE, FALSE, FALSE, FALSE, TRUE, FALSE, FALSE, TRUE, TRUE, FALSE, FALSE, FALSE, TRUE, FALSE, FALSE, TRUE, TRUE, FALSE, FALSE, FALSE, TRUE, FALSE, FALSE, TRUE, TRUE, FALSE, FALSE, FALSE, TRUE, FALSE, FALSE, TRUE, TRUE, FALSE, FALSE, FALSE, TRUE, FALSE, FALSE, TRUE, TRUE, FALSE, FALSE, FALSE, TRUE, FALSE, FALSE, TRUE, TRUE, FALSE, FALSE, FALSE, TRUE, FALSE, FALSE, TRUE, TRUE, FALSE, FALSE, FALSE, TRUE, FALSE, FALSE, TRUE, TRUE, FALSE, FALSE, FALSE, TRUE, FALSE, FALSE, TRUE, TRUE, FALSE, FALSE, FALSE, TRUE, FALSE, FALSE, TRUE, TRUE, FALSE, FALSE, FALSE, TRUE, FALSE, FALSE, TRUE, TRUE, FALSE, FALSE, FALSE, TRUE, FALSE, FALSE, TRUE, TRUE, FALSE, FALSE, FALSE, TRUE, FALSE, FALSE, TRUE, TRUE, FALSE, FALSE, FALSE, TRUE, FALSE, FALSE, TRUE, TRUE, FALSE, FALSE, FALSE, FALSE, FALSE, FALSE, FALSE, FALSE, FALSE, FALSE, FALSE, TRUE, FALSE, FALSE, TRUE, TRUE, FALSE, FALSE, FALSE, TRUE, FALSE, FALSE, TRUE, TRUE, FALSE, FALSE, FALSE, TRUE, FALSE, FALSE, TRUE, TRUE, FALSE, FALSE, FALSE, TRUE, FALSE, FALSE, TRUE, TRUE, FALSE, FALSE, FALSE, TRUE, FALSE, FALSE, TRUE, TRUE, FALSE, FALSE, FALSE, TRUE, FALSE, FALSE, TRUE, TRUE, FALSE, FALSE, FALSE, TRUE, FALSE, FALSE, TRUE, TRUE, FALSE, FALSE, FALSE, TRUE, FALSE, FALSE, TRUE, TRUE, FALSE, FALSE, FALSE, TRUE, FALSE, FALSE, TRUE, TRUE, FALSE, FALSE, FALSE, TRUE, FALSE, FALSE, TRUE, TRUE, FALSE, FALSE, FALSE, TRUE, FALSE, FALSE, TRUE, TRUE, FALSE, FALSE, FALSE, TRUE, FALSE, FALSE, TRUE, TRUE, FALSE, FALSE, FALSE, TRUE, FALSE, FALSE, TRUE, TRUE, FALSE, FALSE, FALSE, TRUE, FALSE, FALSE, TRUE, TRUE, FALSE, FALSE, FALSE, TRUE, FALSE, FALSE, TRUE, TRUE, FALSE, FALSE, FALSE, TRUE, FALSE, FALSE, TRUE, TRUE, FALSE, FALSE, FALSE, FALSE, FALSE, FALSE, FALSE, FALSE]
  in  "SLK":bool
  in  "STB":u16(ring) items=["Monitor Analog"=0, "Monitor Temp"=1, "Monitor Bandgap"=3]
  in  "Array 3":T5(array[cluster])=[[{"sts"=TRUE, "snc"=TRUE, "SG"=0, "ST"=1, "SDC"=FALSE, "SDF"=FALSE}, {"sts"=TRUE, "snc"=TRUE, "SG"=0, "ST"=1, "SDC"=FALSE, "SDF"=FALSE}, {"sts"=TRUE, "snc"=TRUE, "SG"=0, "ST"=3, "SDC"=FALSE, "SDF"=FALSE}, {"sts"=TRUE, "snc"=TRUE, "SG"=0, "ST"=3, "SDC"=FALSE, "SDF"=FALSE}, {"sts"=TRUE, "snc"=TRUE, "SG"=0, "ST"=1, "SDC"=FALSE, "SDF"=FALSE}, {"sts"=TRUE, "snc"=TRUE, "SG"=0, "ST"=1, "SDC"=FALSE, "SDF"=FALSE}, {"sts"=TRUE, "snc"=TRUE, "SG"=0, "ST"=1, "SDC"=FALSE, "SDF"=FALSE}, {"sts"=TRUE, "snc"=TRUE, "SG"=0, "ST"=1, "SDC"=FALSE, "SDF"=FALSE}], [{"sts"=TRUE, "snc"=TRUE, "SG"=0, "ST"=1, "SDC"=FALSE, "SDF"=FALSE}, {"sts"=TRUE, "snc"=TRUE, "SG"=0, "ST"=1, "SDC"=FALSE, "SDF"=FALSE}, {"sts"=TRUE, "snc"=TRUE, "SG"=0, "ST"=3, "SDC"=FALSE, "SDF"=FALSE}, {"sts"=TRUE, "snc"=TRUE, "SG"=0, "ST"=3, "SDC"=FALSE, "SDF"=FALSE}, {"sts"=TRUE, "snc"=TRUE, "SG"=0, "ST"=1, "SDC"=FALSE, "SDF"=FALSE}, {"sts"=TRUE, "snc"=TRUE, "SG"=0, "ST"=1, "SDC"=FALSE, "SDF"=FALSE}, {"sts"=TRUE, "snc"=TRUE, "SG"=0, "ST"=1, "SDC"=FALSE, "SDF"=FALSE}, {"sts"=TRUE, "snc"=TRUE, "SG"=0, "ST"=1, "SDC"=FALSE, "SDF"=FALSE}], [{"sts"=TRUE, "snc"=TRUE, "SG"=0, "ST"=1, "SDC"=FALSE, "SDF"=FALSE}, {"sts"=TRUE, "snc"=TRUE, "SG"=0, "ST"=1, "SDC"=FALSE, "SDF"=FALSE}, {"sts"=TRUE, "snc"=TRUE, "SG"=0, "ST"=3, "SDC"=FALSE, "SDF"=FALSE}, {"sts"=TRUE, "snc"=TRUE, "SG"=0, "ST"=3, "SDC"=FALSE, "SDF"=FALSE}, {"sts"=TRUE, "snc"=TRUE, "SG"=0, "ST"=1, "SDC"=FALSE, "SDF"=FALSE}, {"sts"=TRUE, "snc"=TRUE, "SG"=0, "ST"=1, "SDC"=FALSE, "SDF"=FALSE}, {"sts"=TRUE, "snc"=TRUE, "SG"=0, "ST"=1, "SDC"=FALSE, "SDF"=FALSE}, {"sts"=TRUE, "snc"=TRUE, "SG"=0, "ST"=1, "SDC"=FALSE, "SDF"=FALSE}], [{"sts"=TRUE, "snc"=TRUE, "SG"=0, "ST"=1, "SDC"=FALSE, "SDF"=FALSE}, {"sts"=TRUE, "snc"=TRUE, "SG"=0, "ST"=1, "SDC"=FALSE, "SDF"=FALSE}, {"sts"=TRUE, "snc"=TRUE, "SG"=0, "ST"=3, "SDC"=FALSE, "SDF"=FALSE}, {"sts"=TRUE, "snc"=TRUE, "SG"=0, "ST"=3, "SDC"=FALSE, "SDF"=FALSE}, {"sts"=TRUE, "snc"=TRUE, "SG"=0, "ST"=1, "SDC"=FALSE, "SDF"=FALSE}, {"sts"=TRUE, "snc"=TRUE, "SG"=0, "ST"=1, "SDC"=FALSE, "SDF"=FALSE}, {"sts"=TRUE, "snc"=TRUE, "SG"=0, "ST"=1, "SDC"=FALSE, "SDF"=FALSE}, {"sts"=TRUE, "snc"=TRUE, "SG"=0, "ST"=1, "SDC"=FALSE, "SDF"=FALSE}], [{"sts"=TRUE, "snc"=TRUE, "SG"=0, "ST"=1, "SDC"=FALSE, "SDF"=FALSE}, {"sts"=TRUE, "snc"=TRUE, "SG"=0, "ST"=1, "SDC"=FALSE, "SDF"=FALSE}, {"sts"=TRUE, "snc"=TRUE, "SG"=0, "ST"=3, "SDC"=FALSE, "SDF"=FALSE}, {"sts"=TRUE, "snc"=TRUE, "SG"=0, "ST"=3, "SDC"=FALSE, "SDF"=FALSE}, {"sts"=TRUE, "snc"=TRUE, "SG"=0, "ST"=1, "SDC"=FALSE, "SDF"=FALSE}, {"sts"=TRUE, "snc"=TRUE, "SG"=0, "ST"=1, "SDC"=FALSE, "SDF"=FALSE}, {"sts"=TRUE, "snc"=TRUE, "SG"=0, "ST"=1, "SDC"=FALSE, "SDF"=FALSE}, {"sts"=TRUE, "snc"=TRUE, "SG"=0, "ST"=1, "SDC"=FALSE, "SDF"=FALSE}], [{"sts"=TRUE, "snc"=TRUE, "SG"=0, "ST"=1, "SDC"=FALSE, "SDF"=FALSE}, {"sts"=TRUE, "snc"=TRUE, "SG"=0, "ST"=1, "SDC"=FALSE, "SDF"=FALSE}, {"sts"=TRUE, "snc"=TRUE, "SG"=0, "ST"=3, "SDC"=FALSE, "SDF"=FALSE}, {"sts"=TRUE, "snc"=TRUE, "SG"=0, "ST"=3, "SDC"=FALSE, "SDF"=FALSE}, {"sts"=TRUE, "snc"=TRUE, "SG"=0, "ST"=1, "SDC"=FALSE, "SDF"=FALSE}, {"sts"=TRUE, "snc"=TRUE, "SG"=0, "ST"=1, "SDC"=FALSE, "SDF"=FALSE}, {"sts"=TRUE, "snc"=TRUE, "SG"=0, "ST"=1, "SDC"=FALSE, "SDF"=FALSE}, {"sts"=TRUE, "snc"=TRUE, "SG"=0, "ST"=1, "SDC"=FALSE, "SDF"=FALSE}], [{"sts"=TRUE, "snc"=TRUE, "SG"=0, "ST"=1, "SDC"=FALSE, "SDF"=FALSE}, {"sts"=TRUE, "snc"=TRUE, "SG"=0, "ST"=1, "SDC"=FALSE, "SDF"=FALSE}, {"sts"=TRUE, "snc"=TRUE, "SG"=0, "ST"=3, "SDC"=FALSE, "SDF"=FALSE}, {"sts"=TRUE, "snc"=TRUE, "SG"=0, "ST"=3, "SDC"=FALSE, "SDF"=FALSE}, {"sts"=TRUE, "snc"=TRUE, "SG"=0, "ST"=1, "SDC"=FALSE, "SDF"=FALSE}, {"sts"=TRUE, "snc"=TRUE, "SG"=0, "ST"=1, "SDC"=FALSE, "SDF"=FALSE}, {"sts"=TRUE, "snc"=TRUE, "SG"=0, "ST"=1, "SDC"=FALSE, "SDF"=FALSE}, {"sts"=TRUE, "snc"=TRUE, "SG"=0, "ST"=1, "SDC"=FALSE, "SDF"=FALSE}], [{"sts"=TRUE, "snc"=TRUE, "SG"=0, "ST"=1, "SDC"=FALSE, "SDF"=FALSE}, {"sts"=TRUE, "snc"=TRUE, "SG"=0, "ST"=1, "SDC"=FALSE, "SDF"=FALSE}, {"sts"=TRUE, "snc"=TRUE, "SG"=0, "ST"=3, "SDC"=FALSE, "SDF"=FALSE}, {"sts"=TRUE, "snc"=TRUE, "SG"=0, "ST"=3, "SDC"=FALSE, "SDF"=FALSE}, {"sts"=TRUE, "snc"=TRUE, "SG"=0, "ST"=1, "SDC"=FALSE, "SDF"=FALSE}, {"sts"=TRUE, "snc"=TRUE, "SG"=0, "ST"=1, "SDC"=FALSE, "SDF"=FALSE}, {"sts"=TRUE, "snc"=TRUE, "SG"=0, "ST"=1, "SDC"=FALSE, "SDF"=FALSE}, {"sts"=TRUE, "snc"=TRUE, "SG"=0, "ST"=1, "SDC"=FALSE, "SDF"=FALSE}], [{"sts"=TRUE, "snc"=TRUE, "SG"=0, "ST"=1, "SDC"=FALSE, "SDF"=FALSE}, {"sts"=TRUE, "snc"=TRUE, "SG"=0, "ST"=1, "SDC"=FALSE, "SDF"=FALSE}, {"sts"=TRUE, "snc"=TRUE, "SG"=0, "ST"=3, "SDC"=FALSE, "SDF"=FALSE}, {"sts"=TRUE, "snc"=TRUE, "SG"=0, "ST"=3, "SDC"=FALSE, "SDF"=FALSE}, {"sts"=TRUE, "snc"=TRUE, "SG"=0, "ST"=1, "SDC"=FALSE, "SDF"=FALSE}, {"sts"=TRUE, "snc"=TRUE, "SG"=0, "ST"=1, "SDC"=FALSE, "SDF"=FALSE}, {"sts"=TRUE, "snc"=TRUE, "SG"=0, "ST"=1, "SDC"=FALSE, "SDF"=FALSE}, {"sts"=TRUE, "snc"=TRUE, "SG"=0, "ST"=1, "SDC"=FALSE, "SDF"=FALSE}], [{"sts"=TRUE, "snc"=TRUE, "SG"=0, "ST"=1, "SDC"=FALSE, "SDF"=FALSE}, {"sts"=TRUE, "snc"=TRUE, "SG"=0, "ST"=1, "SDC"=FALSE, "SDF"=FALSE}, {"sts"=TRUE, "snc"=TRUE, "SG"=0, "ST"=3, "SDC"=FALSE, "SDF"=FALSE}, {"sts"=TRUE, "snc"=TRUE, "SG"=0, "ST"=3, "SDC"=FALSE, "SDF"=FALSE}, {"sts"=TRUE, "snc"=TRUE, "SG"=0, "ST"=1, "SDC"=FALSE, "SDF"=FALSE}, {"sts"=TRUE, "snc"=TRUE, "SG"=0, "ST"=1, "SDC"=FALSE, "SDF"=FALSE}, {"sts"=TRUE, "snc"=TRUE, "SG"=0, "ST"=1, "SDC"=FALSE, "SDF"=FALSE}, {"sts"=TRUE, "snc"=TRUE, "SG"=0, "ST"=1, "SDC"=FALSE, "SDF"=FALSE}], [{"sts"=TRUE, "snc"=TRUE, "SG"=0, "ST"=1, "SDC"=FALSE, "SDF"=FALSE}, {"sts"=TRUE, "snc"=TRUE, "SG"=0, "ST"=1, "SDC"=FALSE, "SDF"=FALSE}, {"sts"=TRUE, "snc"=TRUE, "SG"=0, "ST"=3, "SDC"=FALSE, "SDF"=FALSE}, {"sts"=TRUE, "snc"=TRUE, "SG"=0, "ST"=3, "SDC"=FALSE, "SDF"=FALSE}, {"sts"=TRUE, "snc"=TRUE, "SG"=0, "ST"=1, "SDC"=FALSE, "SDF"=FALSE}, {"sts"=TRUE, "snc"=TRUE, "SG"=0, "ST"=1, "SDC"=FALSE, "SDF"=FALSE}, {"sts"=TRUE, "snc"=TRUE, "SG"=0, "ST"=1, "SDC"=FALSE, "SDF"=FALSE}, {"sts"=TRUE, "snc"=TRUE, "SG"=0, "ST"=1, "SDC"=FALSE, "SDF"=FALSE}], [{"sts"=TRUE, "snc"=TRUE, "SG"=0, "ST"=1, "SDC"=FALSE, "SDF"=FALSE}, {"sts"=TRUE, "snc"=TRUE, "SG"=0, "ST"=1, "SDC"=FALSE, "SDF"=FALSE}, {"sts"=TRUE, "snc"=TRUE, "SG"=0, "ST"=3, "SDC"=FALSE, "SDF"=FALSE}, {"sts"=TRUE, "snc"=TRUE, "SG"=0, "ST"=3, "SDC"=FALSE, "SDF"=FALSE}, {"sts"=TRUE, "snc"=TRUE, "SG"=0, "ST"=1, "SDC"=FALSE, "SDF"=FALSE}, {"sts"=TRUE, "snc"=TRUE, "SG"=0, "ST"=1, "SDC"=FALSE, "SDF"=FALSE}, {"sts"=TRUE, "snc"=TRUE, "SG"=0, "ST"=1, "SDC"=FALSE, "SDF"=FALSE}, {"sts"=TRUE, "snc"=TRUE, "SG"=0, "ST"=1, "SDC"=FALSE, "SDF"=FALSE}], [{"sts"=TRUE, "snc"=TRUE, "SG"=0, "ST"=1, "SDC"=FALSE, "SDF"=FALSE}, {"sts"=TRUE, "snc"=TRUE, "SG"=0, "ST"=1, "SDC"=FALSE, "SDF"=FALSE}, {"sts"=TRUE, "snc"=TRUE, "SG"=0, "ST"=3, "SDC"=FALSE, "SDF"=FALSE}, {"sts"=TRUE, "snc"=TRUE, "SG"=0, "ST"=3, "SDC"=FALSE, "SDF"=FALSE}, {"sts"=TRUE, "snc"=TRUE, "SG"=0, "ST"=1, "SDC"=FALSE, "SDF"=FALSE}, {"sts"=TRUE, "snc"=TRUE, "SG"=0, "ST"=1, "SDC"=FALSE, "SDF"=FALSE}, {"sts"=TRUE, "snc"=TRUE, "SG"=0, "ST"=1, "SDC"=FALSE, "SDF"=FALSE}, {"sts"=TRUE, "snc"=TRUE, "SG"=0, "ST"=1, "SDC"=FALSE, "SDF"=FALSE}], [{"sts"=TRUE, "snc"=TRUE, "SG"=0, "ST"=1, "SDC"=FALSE, "SDF"=FALSE}, {"sts"=TRUE, "snc"=TRUE, "SG"=0, "ST"=1, "SDC"=FALSE, "SDF"=FALSE}, {"sts"=TRUE, "snc"=TRUE, "SG"=0, "ST"=3, "SDC"=FALSE, "SDF"=FALSE}, {"sts"=TRUE, "snc"=TRUE, "SG"=0, "ST"=3, "SDC"=FALSE, "SDF"=FALSE}, {"sts"=TRUE, "snc"=TRUE, "SG"=0, "ST"=1, "SDC"=FALSE, "SDF"=FALSE}, {"sts"=TRUE, "snc"=TRUE, "SG"=0, "ST"=1, "SDC"=FALSE, "SDF"=FALSE}, {"sts"=TRUE, "snc"=TRUE, "SG"=0, "ST"=1, "SDC"=FALSE, "SDF"=FALSE}, {"sts"=TRUE, "snc"=TRUE, "SG"=0, "ST"=1, "SDC"=FALSE, "SDF"=FALSE}], [{"sts"=TRUE, "snc"=TRUE, "SG"=0, "ST"=1, "SDC"=FALSE, "SDF"=FALSE}, {"sts"=TRUE, "snc"=TRUE, "SG"=0, "ST"=1, "SDC"=FALSE, "SDF"=FALSE}, {"sts"=TRUE, "snc"=TRUE, "SG"=0, "ST"=3, "SDC"=FALSE, "SDF"=FALSE}, {"sts"=TRUE, "snc"=TRUE, "SG"=0, "ST"=3, "SDC"=FALSE, "SDF"=FALSE}, {"sts"=TRUE, "snc"=TRUE, "SG"=0, "ST"=1, "SDC"=FALSE, "SDF"=FALSE}, {"sts"=TRUE, "snc"=TRUE, "SG"=0, "ST"=1, "SDC"=FALSE, "SDF"=FALSE}, {"sts"=TRUE, "snc"=TRUE, "SG"=0, "ST"=1, "SDC"=FALSE, "SDF"=FALSE}, {"sts"=TRUE, "snc"=TRUE, "SG"=0, "ST"=1, "SDC"=FALSE, "SDF"=FALSE}], [{"sts"=TRUE, "snc"=TRUE, "SG"=0, "ST"=1, "SDC"=FALSE, "SDF"=FALSE}, {"sts"=TRUE, "snc"=TRUE, "SG"=0, "ST"=1, "SDC"=FALSE, "SDF"=FALSE}, {"sts"=TRUE, "snc"=TRUE, "SG"=0, "ST"=3, "SDC"=FALSE, "SDF"=FALSE}, {"sts"=TRUE, "snc"=TRUE, "SG"=0, "ST"=3, "SDC"=FALSE, "SDF"=FALSE}, {"sts"=TRUE, "snc"=TRUE, "SG"=0, "ST"=1, "SDC"=FALSE, "SDF"=FALSE}, {"sts"=TRUE, "snc"=TRUE, "SG"=0, "ST"=1, "SDC"=FALSE, "SDF"=FALSE}, {"sts"=TRUE, "snc"=TRUE, "SG"=0, "ST"=1, "SDC"=FALSE, "SDF"=FALSE}, {"sts"=TRUE, "snc"=TRUE, "SG"=0, "ST"=1, "SDC"=FALSE, "SDF"=FALSE}]] {"ST" items=["0.5us", "1us", "2us", "3us"]; "SG" items=["4.7 mV/fC", "7.8 mV/fC", "14 mV/fC", "25 mV/fC"]}
  out "size(s)":i32=1096
  out "size(s) 2":i32=1088
  out "ADC SPI OK":bool=TRUE
  out "FE SPI OK":bool=TRUE
  out "ADC FIFO SYNC":u16 format="%016b"
  in  "Array 4":T6(array[cluster])=[{"EN_GR"=0, "CLKG"=2, "FRQC"=1, "F2"=0, "F1"=0}, {"EN_GR"=0, "CLKG"=2, "FRQC"=1, "F2"=0, "F1"=0}, {"EN_GR"=0, "CLKG"=2, "FRQC"=1, "F2"=0, "F1"=0}, {"EN_GR"=0, "CLKG"=2, "FRQC"=1, "F2"=1, "F1"=0}, {"EN_GR"=0, "CLKG"=2, "FRQC"=1, "F2"=0, "F1"=0}, {"EN_GR"=0, "CLKG"=2, "FRQC"=1, "F2"=0, "F1"=0}, {"EN_GR"=0, "CLKG"=2, "FRQC"=1, "F2"=0, "F1"=0}, {"EN_GR"=0, "CLKG"=2, "FRQC"=1, "F2"=0, "F1"=0}] {"F1" items=["FIFO write clock is the ADC write clock", "FIFO write clock is on pin IdxMp/n.  "]; "F2" items=["FIFO clock generator off", "FIFO clock generator  on."]; "FRQC" items=["1 MHz", "2 MHz "]; "CLKG" items=["ADC clocks from monostable", "External clocks", "ADC clocks from digital generator of FIFO", "ADC clocks from monostable"]; "EN_GR" items=["Disables offset current absorption", "Enables the offset current absorption"]}
  in  "EN V6":bool=TRUE
  in  "UDP READ":bool
  in  "UDP WRITE":bool
  out "DATA 3":u32=2031872 format="%x"
  in  "ADDRESS 3":u16=257 format="%x"
  in  "DATA":u32=305419896 format="%x"
  in  "ADDRESS":u16=514 format="%x"
  in  "Remote Host":string="192.168.121.1"
  out "start_udp_IO":string="OK"
  out "UDP_CLEANUP":string="ok"
  in  "ADDRESS 4":u16=514 format="%x"
  out "DATA 4":u32=290 format="%x"
  in  "DATA 2":u32=290 format="%x"
  in  "ADDRESS 2":u16=514 format="%x"
  in  "SBND I2C WRITE":bool
  in  "SBND I2C READ":bool
  in  "UDP/I2C":bool
  in  "LBNE READ BLK":bool
  in  "BLK ADDRESS":u16=8
  out "BLK RD DATA":u32[](array[numeric]) format="%x"
  out "LBNE_DLL_VERSION":u32=102
  in  "Voltage Level (0.0 V) 3":dbl caption="Voltage Level (0.0 V)" format="%.2f"
  in  "Channel (0: +6V Channel)":i32(ring) caption="Channel (0: +6V)" items=["+6V Channel", "+25V Channel", "-25V Channel"]
  in  "Enable OVP (T: Enable)":bool=TRUE
  in  "Behavior (0: Regulate)":u16(ring) items=["Regulate", "Trip"]
  in  "Voltage Limit (0V)":dbl=1.75 format="%.2f"
  in  "Current Limit (0A)":dbl format="%.2f"
  in  "VISA resource name":refnum<visa-resource-name>="USB0::0x1AB1::0x0E10::DP1A154500408::INSTR"
  out "FIMWARE VERSION":u32 format="%x"
  in  "Tab Control 4":T7(tab)
  in  "program \nFLASH":bool
  in  "Numeric":i32
  out "Meter":dbl(knob) scale=0.0..100.0
  out "PAGE 3":i32=15217
  out "READ ARRAY 2":u32[](array[numeric])=[0, 0, 0, 0, 0, 0, 0, 0, 0, 0, 17, 0, 268501009, 268500992, 4352, 268500992, 0, 0, 0, 1114112, 0, 0, 0, 0, 0, 0, 0, 4097, 0, 0, 0, 0, 0, 0, 0, 0, 0, 0, 0, 0, 0, 0, 0, 0, 0, 0, 0, 0, 49346, 3752002095, 1846345728, 0, 2961253394, 1410483634, 2170847556, 2219156004, 304223960, 313009179, 1210598437, 1361318696, 1363678808, 608862849, 1652632961, 1108584484] format="%x"
  out "WRITE ARRAY":u32[](array[numeric])=[2236879429, 310464840, 374875202, 715203606, 3625093268, 2169131592, 626074644, 709969942, 411345938, 1247969573, 2705857704, 612701202, 1410476625, 1209419940, 1210753316, 304159560, 763447890, 1210336293, 2702344466, 2243199396, 306872897, 2994852882, 672421924, 2236879402, 1099452744, 457712194, 709960731, 1210941768, 2219135560, 622944897, 709969947, 1210599466, 1361318744, 311059585, 1163020321, 672573458, 2234810698, 2722638417, 605102474, 1686193490, 1210337890, 2167017881, 2166039579, 1209733701, 1376855178, 1686192513, 1168253974, 2819757512, 2166039579, 1209209428, 323334785, 1686193284, 1168253970, 571922450, 2820938568, 675554641, 605235281, 1209423908, 1250066786, 2167243074, 330842450, 1211453732, 428364104, 374875202] format="%x"
  out "x = y?":bool
  out "pages 2":dbl=15292.25390625
  in  "LOAD RPD":bool
  out "DATA 5":u32 format="%x"
  in  "READ STATUS":bool
  in  "erase flash":bool
  in  "START FROM":i32=15217
  in  "STOP WRITE":bool
  out "DATA 6":u32 format="%x"
  out "NUM ATTEMP":i32=15217
  out "ONE_MORE":i32=15217
  out "x = y? 3":bool
  in  "verify\nFLASH":bool
  out "Meter 2":dbl(knob) scale=0.0..100.0
  out "PAGE 2":i32=15217
  out "READ ARRAY 3":u32[](array[numeric])=[0, 0, 0, 0, 0, 0, 0, 0, 0, 0, 17, 0, 268501009, 268500992, 4352, 268500992, 0, 0, 0, 1114112, 0, 0, 0, 0, 0, 0, 0, 4097, 0, 0, 0, 0, 0, 0, 0, 0, 0, 0, 0, 0, 0, 0, 0, 0, 0, 0, 0, 0, 49346, 3752002095, 1846345728, 0, 2961253394, 1410483634, 2170847556, 2219156004, 304223960, 313009179, 1210598437, 1361318696, 1363678808, 608862849, 1652632961, 1108584484] format="%x"
  out "WRITE ARRAY 2":u32[](array[numeric])=[2236879429, 310464840, 374875202, 715203606, 3625093268, 2169131592, 626074644, 709969942, 411345938, 1247969573, 2705857704, 612701202, 1410476625, 1209419940, 1210753316, 304159560, 763447890, 1210336293, 2702344466, 2243199396, 306872897, 2994852882, 672421924, 2236879402, 1099452744, 457712194, 709960731, 1210941768, 2219135560, 622944897, 709969947, 1210599466, 1361318744, 311059585, 1163020321, 672573458, 2234810698, 2722638417, 605102474, 1686193490, 1210337890, 2167017881, 2166039579, 1209733701, 1376855178, 1686192513, 1168253974, 2819757512, 2166039579, 1209209428, 323334785, 1686193284, 1168253970, 571922450, 2820938568, 675554641, 605235281, 1209423908, 1250066786, 2167243074, 330842450, 1211453732, 428364104, 374875202] format="%x"
  out "x = y? 2":bool
  in  "STOP VERIFY":bool
  in  "blank check":bool
  in  "start from":i32=15217
  in  "read flash":bool
  in  "P OFFSET":i32=15210
  in  "PAGES":i32=10
  out "PAGE":i32=104
  out "READ FROM FLASH":u32[][](array[numeric]) format="%x"
  out "FROM FILE":u32[][](array[numeric]) format="%x"
  in  "SAVE FLASH DATA":bool
  out "error out 2":errorcluster
  # "RAW \nBIN FILE"
  # "1"
  # "1"
  # "2"
  # "2"
  # "3"
  # "3"
  # "4"
  # "4"
  # "5"
  # "5"
  # "6"
  # "6"
  # "7"
  # "7"
  # "8"
  # "8"
  # "STATUS"
  # "0"
  # "1"
  # "2"
  # "3"
  # "4"
  # "5"
  # "6"
  # "7"
  # "8"
  # "9"
  # "10"
  # "11"
  # "12"
  # "13"
  # "14"
  # "15"
  # "STEP 1"
  # "STEP 2"
  # "STEP 3"
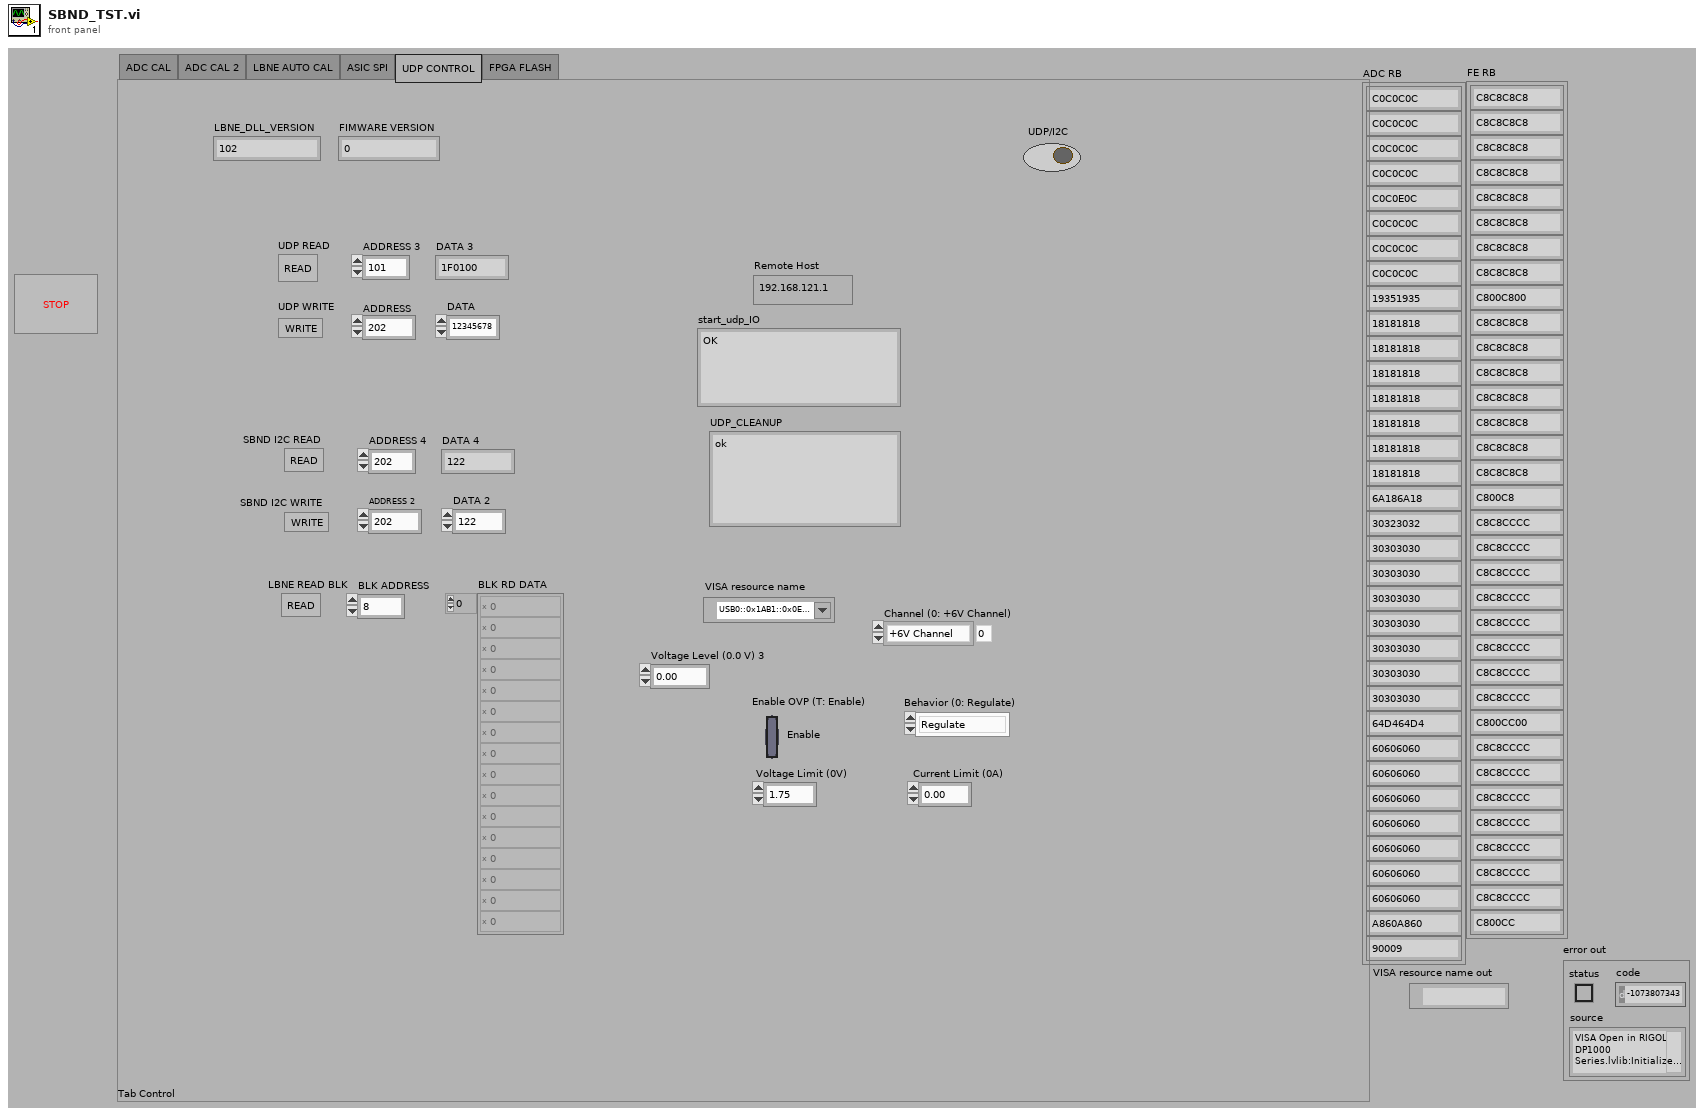
[diagram p1: front panel]
types:
  T1 = enum32{"ADC CAL", "ADC CAL 2", "LBNE AUTO CAL", "ASIC SPI", "UDP CONTROL", "FPGA FLASH"}
  T2 = cluster{"sts":bool, "snc":bool, "SG":u16, "ST":u16, "SDC":bool, "SDF":bool}
  T3 = cluster{"D_offset":u16, "PDSR":bool, "PCSR":bool, "slp":bool, "tst":bool}
  T4 = cluster{"D_offset":u16, "PDSR":bool, "PCSR":bool, "slp":bool, "tst":bool}[][]
  T5 = cluster{"sts":bool, "snc":bool, "SG":u16, "ST":u16, "SDC":bool, "SDF":bool}[][]
  T6 = cluster{"EN_GR":u16, "CLKG":u16, "FRQC":u16, "F2":u16, "F1":u16}[]
  T7 = enum32{"PROGRAM FPGA", "VERIFY FPGA", "READ BACK AND SAVE"}
  T8 = cluster{"averaging mode":u16, "weighting mode":u16, "number of averages":u32}
  T9 = cluster{"dB On (F)":bool, "unwrap phase (F)":bool, "convert to degree (F)":bool}
  T10 = enum16{"open", "replace", "create", "open or create", "replace or create", "replace or create with confirmation"}
  T11 = enum16{"deny read/write", "deny write-only", "deny none"}
  T12 = cluster{"D_offset":u16, "PDSR":bool, "PCSR":bool, "slp":bool, "tst":bool}[]
  T13 = cluster{"sts":bool, "snc":bool, "SG":u16, "ST":u16, "SDC":bool, "SDF":bool}[]
  T14 = cluster{"EN_GR":u16, "CLKG":u16, "FRQC":u16, "F2":u16, "F1":u16}
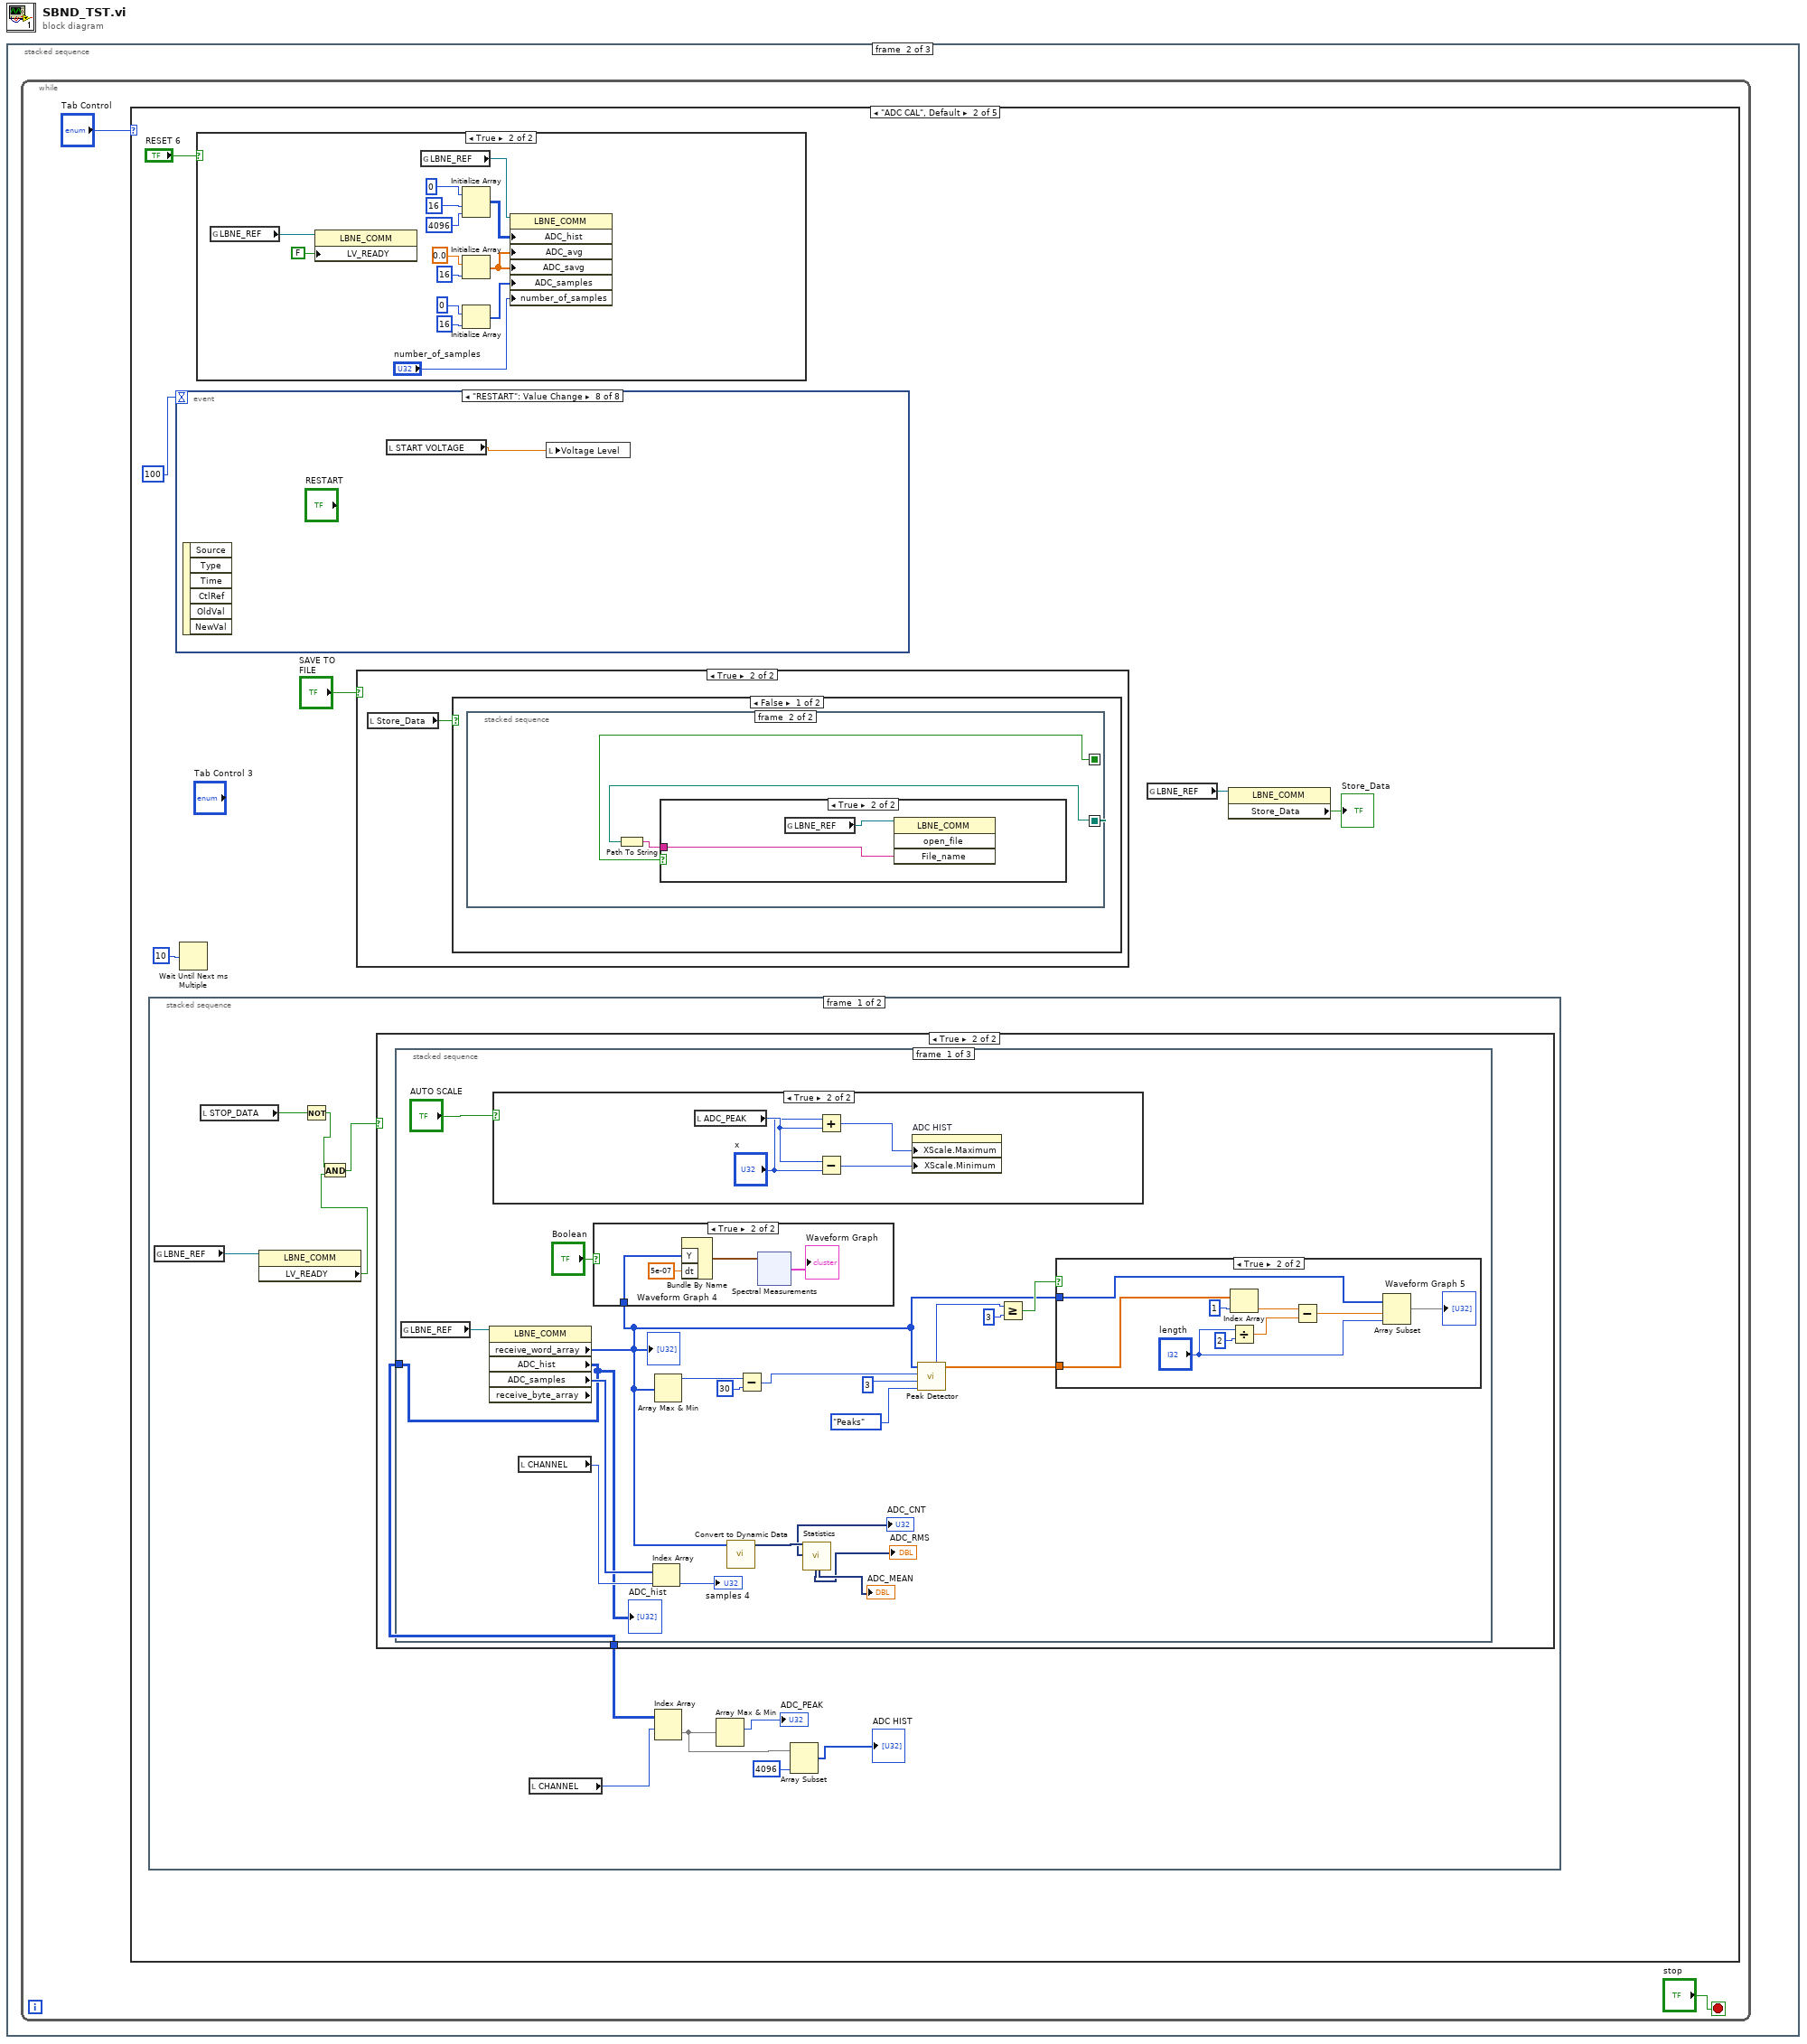
[diagram p0: block diagram]
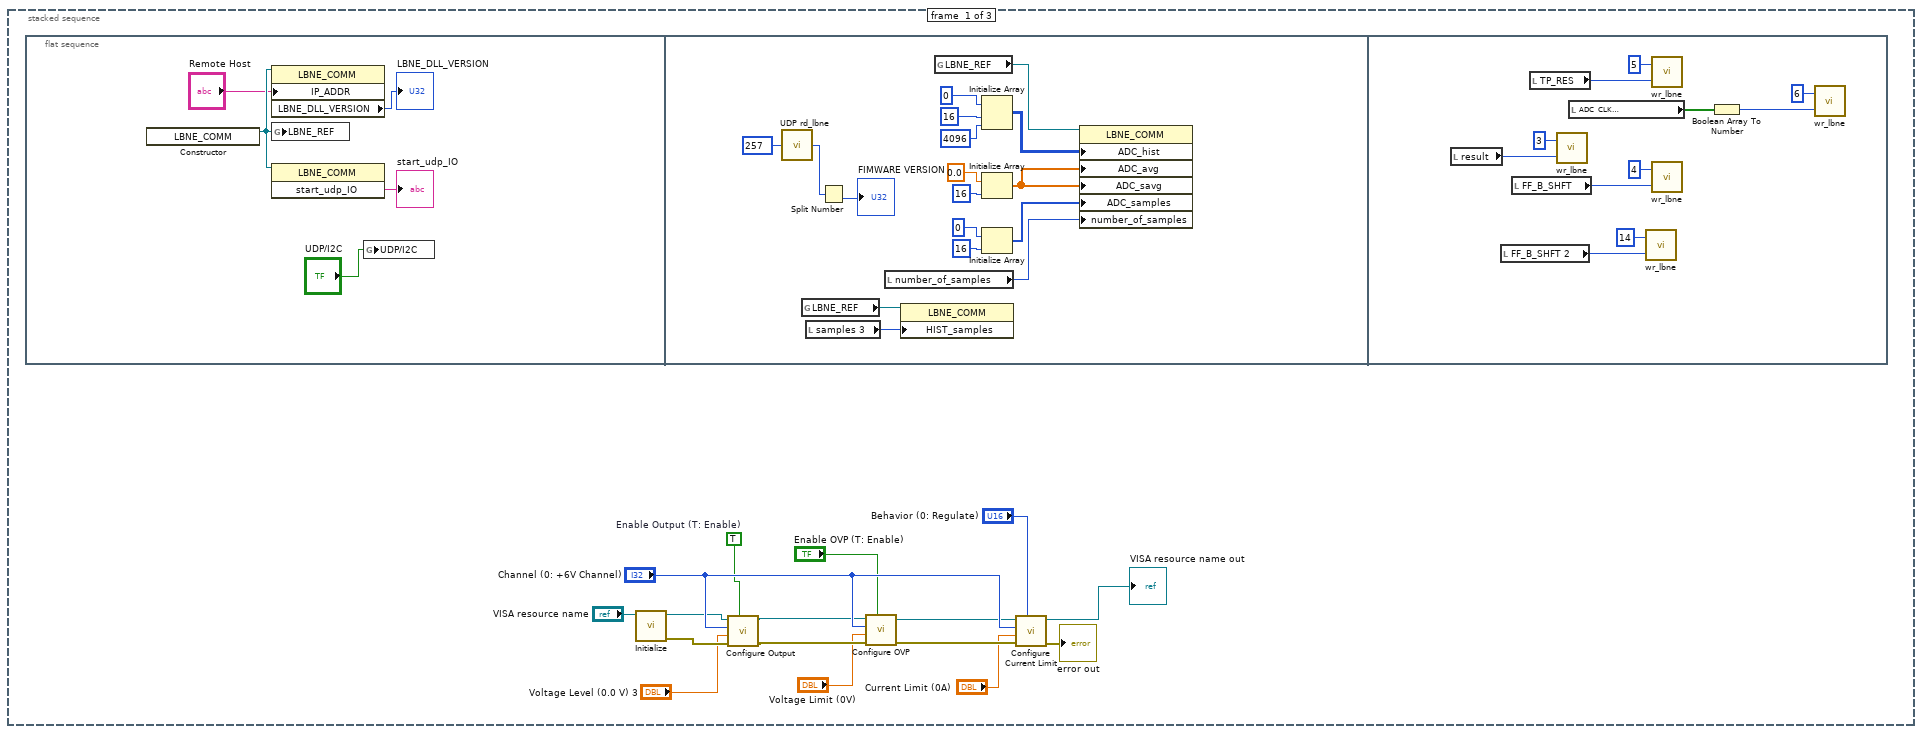
[diagram p2: hidden frame]
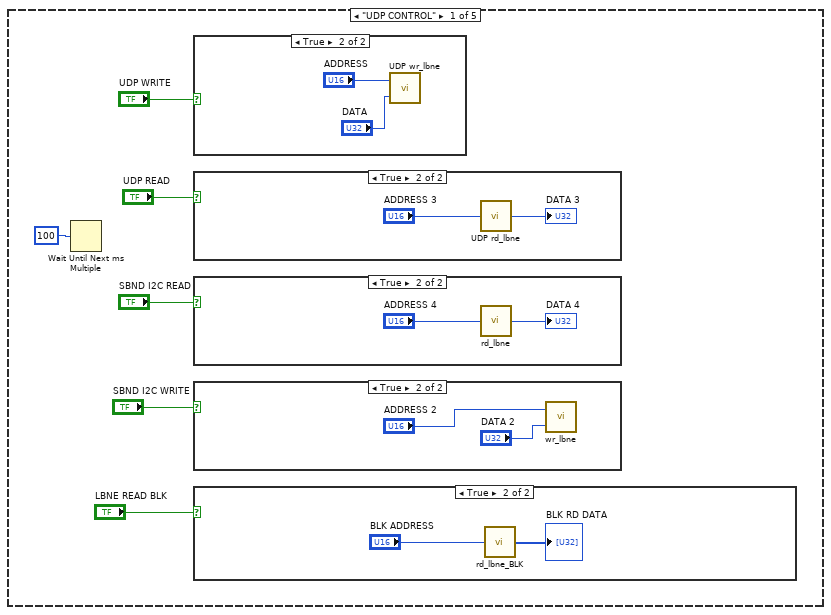
[diagram p3: hidden frame]
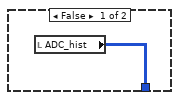
[diagram p9: hidden frame]
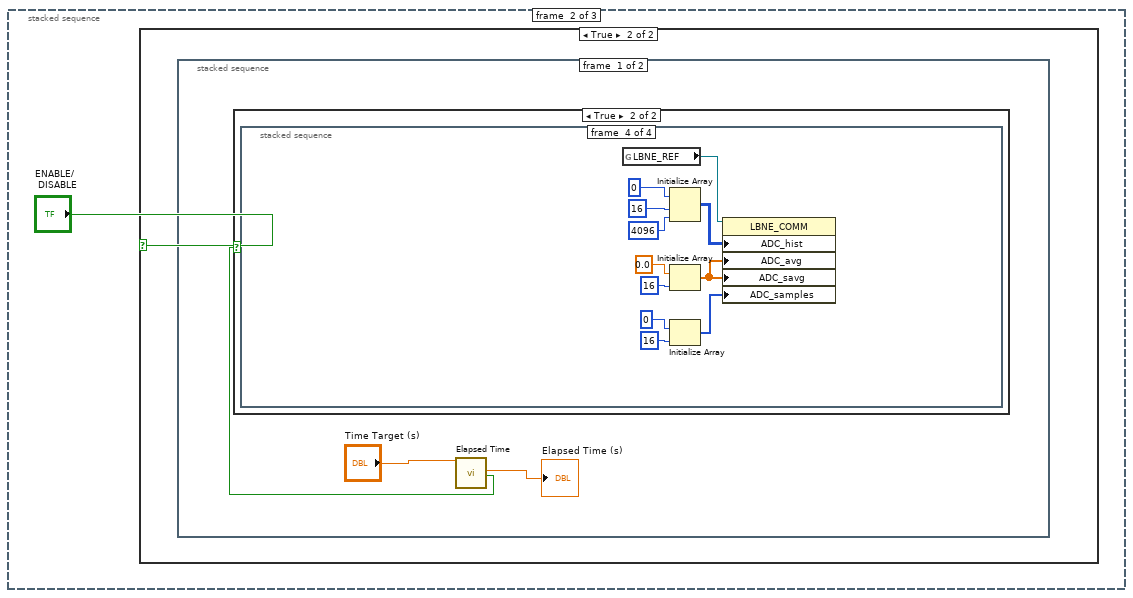
[diagram p13: hidden frame]
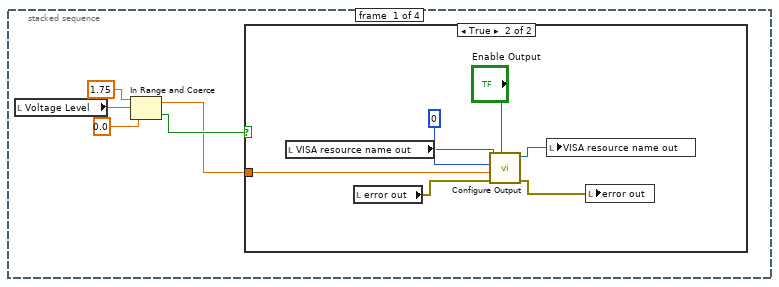
[diagram p16: hidden frame]
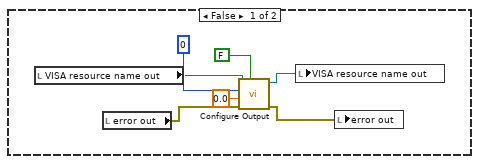
[diagram p17: hidden frame]
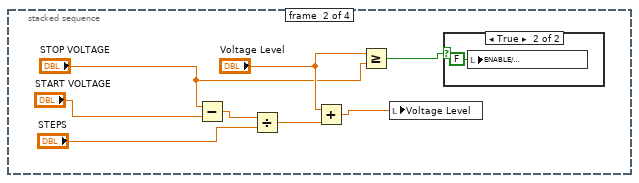
[diagram p18: hidden frame]
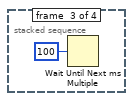
[diagram p20: hidden frame]
diagram:
  n1 = stacked-sequence {
    frame #0 {
      w10 = TRUE  # Enable Output (T: Enable)
      n2 = flat-sequence {
        frame #0 {
          n3 = constructor class="LBNE_COMM"() -> (reference out=w21:refnum<k24>)  [unwired: 3 in, 2 out]
          n4 = property class="LBNE_COMM"(reference=w21, "IP_ADDR"="Remote Host") -> ("LBNE_DLL_VERSION"=→"LBNE_DLL_VERSION":u32)  [unwired: 1 in, 2 out]
          n5 = global write "LBNE_Global .vi" "LBNE_REF"(w21) -> ()
          n6 = invoke class="LBNE_COMM" method="start_udp_IO"(reference=w21) -> ("start_udp_IO"=→"start_udp_IO":string)  [unwired: 2 in, 2 out]
          n7 = global write "LBNE_Global .vi" "UDP/I2C"("UDP/I2C") -> ()
        }
        frame #1 {
          n8 = call "UDP rd_lbne.vi"("ADDRESS 2"=i16 257) -> ("DATA 2"=w22:u32)
          n9 = global read "LBNE_Global .vi" "LBNE_REF"() -> (w37:refnum<k24>)
          n10 = local read "samples 3"() -> (w38:i32)
          n11 = Split Number(x=w22) -> (lo(x)=→"FIMWARE VERSION":u16)  [unwired: 1 out]
          n12 = local read "number_of_samples"() -> (w36:u32)
          n13 = property class="LBNE_COMM"(reference=w37, "HIST_samples"=w38) -> ()  [unwired: 1 in, 2 out]
          n14 = global read "LBNE_Global .vi" "LBNE_REF"() -> (w25:refnum<k24>)
          n15 = Initialize Array(u32 0 ("element"), 16 ("dimension size"), 4096 ("dimension size")) -> (w29:u32[][])
          n16 = Initialize Array(0.0 ("element"), 16 ("dimension size")) -> (w32:dbl[])
          n17 = Initialize Array(u32 0 ("element"), 16 ("dimension size")) -> (w34:u32[])
          n18 = property class="LBNE_COMM"(reference=w25, "ADC_hist"=w29, "ADC_avg"=w32, "ADC_savg"=w32, "ADC_samples"=w34, "number_of_samples"=w36) -> ()  [unwired: 1 in, 2 out]
        }
        frame #2 {
          n19 = local read "result"() -> (w46:u32)
          n20 = local read "FF_B_SHFT 2"() -> (w40:u32)
          n21 = local read "FF_B_SHFT"() -> (w49:u32)
          n22 = local read "TP_RES"() -> (w41:u32)
          n23 = call "wr_lbne.vi"("DATA"=w46, "ADDRESS"=u16 3) -> ()  [unwired: 1 out]
          n24 = local read "ADC  CLK \nPHASE"() -> (w43:bool[])
          n25 = call "wr_lbne.vi"("DATA"=w40, "ADDRESS"=u16 14) -> ()  [unwired: 1 out]
          n26 = call "wr_lbne.vi"("DATA"=w41, "ADDRESS"=u16 5) -> ()  [unwired: 1 out]
          n27 = call "wr_lbne.vi"("DATA"=w49, "ADDRESS"=u16 4) -> ()  [unwired: 1 out]
          n28 = Boolean Array To Number(Boolean array=w43) -> (number=w45:u32)
          n29 = call "wr_lbne.vi"("DATA"=w45, "ADDRESS"=u16 6 ("address")) -> ()  [unwired: 1 out]
        }
      }
      n30 = call <instrlib>:"Initialize.vi"("VISA resource name"="VISA resource name") -> ("error out"=w14:errorcluster, "VISA resource name out"=w15:refnum<visa-resource-name>)  [unwired: 4 in, 5 out]
      n31 = call <instrlib>:"Configure Output.vi"("Enable Output (T: Enable)"=w10, "error in (no error)"=w14, "Voltage Level (0.0 V)"="Voltage Level (0.0 V) 3", "Channel (0: +6V Channel)"="Channel (0: +6V Channel)", "VISA resource name"=w15) -> ("error out"=w13:errorcluster, "VISA resource name out"=w12:refnum<visa-resource-name>)  [unwired: 5 out]
      n32 = call <instrlib>:"Configure OVP.vi"("Enable OVP (T: Enable)"="Enable OVP (T: Enable)", "error in (no error)"=w13, "Voltage Limit (6.5 V)"="Voltage Limit (0V)", "Channel (0: +6V Channel)"="Channel (0: +6V Channel)", "VISA resource name"=w12) -> ("error out"=w5:errorcluster, "VISA resource name out"=w6:refnum<visa-resource-name>)  [unwired: 5 out]
      n33 = call <instrlib>:"Configure Current Limit.vi"("Behavior (0: Regulate)"="Behavior (0: Regulate)", "error in (no error)"=w5, "Current Limit (5.0 A)"="Current Limit (0A)", "Channel (0: +6V Channel)"="Channel (0: +6V Channel)", "VISA resource name"=w6) -> ("error out"=→"error out":errorcluster, "VISA resource name out"=→"VISA resource name out":refnum<visa-resource-name>)  [unwired: 5 out]
    }
    frame #1 {
      n34 = while {
        stop <- "stop" stop-if-true
        n35 = case shown="\"ADC CAL\", Default" "Tab Control" {
          frame "UDP CONTROL" {
            n36 = Wait Until Next ms Multiple(millisecond multiple=u32 100) -> ()  [unwired: 1 out]
            n37 = case shown="True" "UDP WRITE" {
              frame False {
              }
              frame True {
                n38 = call "UDP wr_lbne.vi"("DATA"="DATA", "ADDRESS"="ADDRESS") -> ()  [unwired: 1 out]
              }
            }
            n39 = case shown="True" "UDP READ" {
              frame False {
              }
              frame True {
                n40 = call "UDP rd_lbne.vi"("ADDRESS 2"="ADDRESS 3") -> ("DATA 2"=→"DATA 3":u32)
              }
            }
            n41 = case shown="True" "SBND I2C READ" {
              frame False {
              }
              frame True {
                n42 = call "rd_lbne.vi"("ADDRESS 2"="ADDRESS 4") -> ("DATA 2"=→"DATA 4":u32)
              }
            }
            n43 = case shown="True" "SBND I2C WRITE" {
              frame False {
              }
              frame True {
                n44 = call "wr_lbne.vi"("DATA"="DATA 2", "ADDRESS"="ADDRESS 2") -> ()  [unwired: 1 out]
              }
            }
            n45 = case shown="True" "LBNE READ BLK" {
              frame False {
              }
              frame True {
                n46 = call "rd_lbne_BLK.vi"("ADDRESS 2"="BLK ADDRESS") -> ("Array"=→"BLK RD DATA":u32[])
              }
            }
          }
          frame "ADC CAL", Default {
            n47 = stacked-sequence {
              frame #0 {
                n48 = global read "LBNE_Global .vi" "LBNE_REF"() -> (w77:refnum<k24>)
                n49 = local read "STOP_DATA"() -> (w84:bool)
                n50 = property class="LBNE_COMM"(reference=w77) -> ("LV_READY"=w75:bool)  [unwired: 1 in, 2 out]
                n51 = Not(x=w84) -> (.not. x?=w76:bool)
                n52 = And(x=w76, y=w75) -> (x .and. y?=w74:bool)
                n53 = case shown="True" w74 {
                  tunnel: [w85 w86] -> w78
                  frame False {
                    n54 = local read "ADC_hist"() -> (w85:u32[][])
                  }
                  frame True {
                    n55 = stacked-sequence {
                      tunnel: [w90 _ _] -> w86
                      frame #0 {
                        n56 = global read "LBNE_Global .vi" "LBNE_REF"() -> (w103:refnum<k24>)
                        n57 = property class="LBNE_COMM" props=["receive_word_array", "ADC_hist", "ADC_samples", "receive_byte_array"](reference=w103) -> ("receive_word_array"=w89:u32[], "ADC_hist"=w90:u32[][], "ADC_samples"=w98:u32[])  [unwired: 1 in, 3 out]
                        "Waveform Graph 4" <- w89
                        "ADC_hist" <- w90
                        n58 = case shown="True" "AUTO SCALE" {
                          frame False {
                          }
                          frame True {
                            n59 = local read "ADC_PEAK"() -> (w135:u32)
                            n60 = Add(x="x", y=w135) -> (x+y=w134:u32)
                            n61 = Subtract(x=w135, y="x") -> (x-y=w133:u32)
                            n62 = property on="ADC HIST" class="WFGraph (strict)"("XScale.Maximum"=w134, "XScale.Minimum"=w133) -> ()  [unwired: 2 in, 2 out]
                          }
                        }
                        n63 = local read "CHANNEL"() -> (w97:u8)
                        n64 = case shown="True" "Boolean" {
                          tunnel: w89 -> [_ w110]
                          frame False {
                          }
                          frame True {
                            n65 = Bundle By Name("Y"=w110, "dt"=5e-07) -> (w109:waveform(u32))  [unwired: 1 in]
                            n66 = xnode "Spectral Measurements"("Signals"=w109) -> ("FFT - (Peak)"=→"Waveform Graph":cluster{"f0":dbl, "df":dbl, "magnitude":dbl[]})  [unwired: 2 in, 3 out]
                          }
                        }
                        n67 = Index Array(array=w98, index=w97) -> (element=→"samples 4":u32)
                        n68 = Array Max & Min(array=w89) -> (max value=w104:u32)  [unwired: 3 out]
                        n69 = call "Convert to Dynamic Data"("Array"=w89) -> ("Dynamic Data Type"=w101:dynamicdata)  [unwired: 3 in]
                        n70 = Subtract(x=w104, y=30) -> (x-y=w105:u32)
                        n71 = call "Statistics"("Signals"=w101) -> ("Total Samples"=→"ADC_CNT":dynamicdata, "Standard Dev"=→"ADC_RMS":dynamicdata, "Arithmetic Mean"=→"ADC_MEAN":dynamicdata)  [unwired: 23 in, 1 out]
                        n72 = call <vilib>:"Peak Detector.vi"("peaks/valleys"=enum32{"Peaks", "Valleys"}."Peaks", "width"=3, "threshold"=w105, "X"=w89) -> ("Locations"=w95:dbl[], "# found"=w93:i32)  [unwired: 3 in, 3 out]
                        n73 = Greater Or Equal?(x=w93, y=3 ("x")) -> (x >= y?=w96:bool)
                        n74 = case shown="True" w96 {
                          tunnel: w95 -> [_ w131]
                          tunnel: w89 -> [_ w127]
                          frame False {
                          }
                          frame True {
                            n75 = Index Array(array=w131, index=1) -> (element=w128:dbl)
                            n76 = Divide(x="length", y=2) -> (x/y=w125:dbl)
                            n77 = Subtract(x=w128, y=w125) -> (x-y=w126:dbl)
                            n78 = Array Subset(array=w127, index=w126, length="length") -> (→"Waveform Graph 5":u32[])
                          }
                        }
                      }
                      frame #1 {
                        n79 = case shown="True" "ENABLE/\n DISABLE" {
                          frame False {
                          }
                          frame True {
                            n80 = stacked-sequence {
                              frame #0 {
                                n81 = call "Elapsed Time"("Time Target (s)"="Time Target (s)") -> ("Elapsed Time (s)"=→"Elapsed Time (s)":dbl, "Time has Elapsed"=w137:bool)  [unwired: 11 in, 6 out]
                                n82 = case shown="True" w137 {
                                frame False {
                                }
                                frame True {
                                n83 = stacked-sequence {
                                frame #0 {
                                n84 = local read "Voltage Level"() -> (w141:dbl)
                                n85 = In Range and Coerce(upper limit=1.75, x=w141, lower limit=0.0) -> (coerced(x)=w140:dbl, In Range?=w144:bool)
                                n86 = case shown="True" w144 {
                                tunnel: w140 -> [_ w152]
                                frame False {
                                n87 = local read "VISA resource name out"() -> (w149:refnum<visa-resource-name>)
                                n88 = local read "error out"() -> (w150:errorcluster)
                                n89 = call <instrlib>:"Configure Output.vi"("Enable Output (T: Enable)"=FALSE, "error in (no error)"=w150, "Voltage Level (0.0 V)"=0.0, "Channel (0: +6V Channel)"=0, "VISA resource name"=w149) -> ("error out"=w147:errorcluster, "VISA resource name out"=w148:refnum<visa-resource-name>)  [unwired: 5 out]
                                n90 = local write "VISA resource name out"(w148) -> ()
                                n91 = local write "error out"(w147) -> ()
                                }
                                frame True {
                                n92 = local read "VISA resource name out"() -> (w156:refnum<visa-resource-name>)
                                n93 = local read "error out"() -> (w157:errorcluster)
                                n94 = call <instrlib>:"Configure Output.vi"("Enable Output (T: Enable)"="Enable Output", "error in (no error)"=w157, "Voltage Level (0.0 V)"=w152, "Channel (0: +6V Channel)"=0, "VISA resource name"=w156) -> ("error out"=w153:errorcluster, "VISA resource name out"=w154:refnum<visa-resource-name>)  [unwired: 5 out]
                                n95 = local write "VISA resource name out"(w154) -> ()
                                n96 = local write "error out"(w153) -> ()
                                }
                                }
                                }
                                frame #1 {
                                n97 = Subtract(x="STOP VOLTAGE", y="START VOLTAGE") -> (x-y=w163:dbl)
                                n98 = Divide(x=w163, y="STEPS") -> (x/y=w165:dbl)
                                n99 = Add(x="Voltage Level", y=w165) -> (x+y=w166:dbl)
                                n100 = Greater Or Equal?(x="Voltage Level", y="STOP VOLTAGE") -> (x >= y?=w159:bool)
                                n101 = local write "Voltage Level"(w166) -> ()
                                n102 = case shown="True" w159 {
                                frame False {
                                }
                                frame True {
                                n103 = local write "ENABLE/\n DISABLE"(FALSE ("ENABLE/\n DISABLE")) -> ()
                                }
                                }
                                }
                                frame #2 {
                                n104 = Wait Until Next ms Multiple(millisecond multiple=u32 100) -> ()  [unwired: 1 out]
                                }
                                frame #3 {
                                n105 = global read "LBNE_Global .vi" "LBNE_REF"() -> (w169:refnum<k24>)
                                n106 = Initialize Array(u32 0 ("element"), 16 ("dimension size"), 4096 ("dimension size")) -> (w173:u32[][])
                                n107 = Initialize Array(0.0 ("element"), 16 ("dimension size")) -> (w176:dbl[])
                                n108 = Initialize Array(u32 0 ("element"), 16 ("dimension size")) -> (w178:u32[])
                                n109 = property class="LBNE_COMM"(reference=w169, "ADC_hist"=w173, "ADC_avg"=w176, "ADC_savg"=w176, "ADC_samples"=w178) -> ()  [unwired: 1 in, 2 out]
                                }
                                }
                                }
                                }
                              }
                              frame #1 {
                              }
                            }
                          }
                        }
                      }
                      frame #2 {
                        n110 = global read "LBNE_Global .vi" "LBNE_REF"() -> (w180:refnum<k24>)
                        n111 = property class="LBNE_COMM"(reference=w180, "LV_READY"=FALSE) -> ()  [unwired: 1 in, 2 out]
                      }
                    }
                  }
                }
                n112 = local read "CHANNEL"() -> (w82:u8)
                n113 = Index Array(array=w78, index (row)=w82) -> (element=w83:u32[])  [unwired: 1 in]
                n114 = Array Max & Min(array=w83) -> (max index (indices)=→"ADC_PEAK":i32)  [unwired: 3 out]
                n115 = Array Subset(array=w83, length=4096) -> (→"ADC HIST":u32[])  [unwired: 1 in]
              }
              frame #1 {
              }
            }
            n116 = event shown="[7] \"RESTART\": Value Change" {
              selector: _ -> [_ _ _ _ _ _ _ _]
              dyn-events: _ -> [_ _ _ _ _ _ _ _]
              timeout: 100 -> [_ _ _ _ _ _ _ _]
              event Timeout {
                n117 = event-data() -> ()  [unwired: 1 in, 2 out]
              }
              event "ADC_TM EN", "TEST PAT", "TEST EN", "ADC  CLK \nPHASE", "DATA SHIFT": Value Change {
                n118 = event-data() -> ()  [unwired: 1 in, 6 out]
                n119 = for {
                  tunnel: "DATA SHIFT" -> [w231] mode=indexing
                  shift-right: [w226] -> _
                  shift-left: bool[] [] -> [w228]
                  tunnel: [w227] -> w205
                  tunnel: [w224] -> w203
                  w225 = 32 ("length")
                  n120 = Number To Boolean Array(number=w231) -> (Boolean array=w230:bool[])
                  n121 = Array Subset(array=w230, length=8) -> (w229:bool[])  [unwired: 1 in]
                  n122 = Build Array (concatenate)(w228, w229) -> (w226:bool[])
                  n123 = Array Subset(array=w226, length=w225) -> (w227:bool[])  [unwired: 1 in]
                  n124 = Array Subset(array=w226, index=w225, length=w225) -> (w224:bool[])
                }
                n125 = Boolean Array To Number(Boolean array="ADC  CLK \nPHASE") -> (number=w209:u32)
                n126 = Boolean To (0,1)(Boolean="ADC_TM EN") -> (0, 1=w214:i16)
                n127 = call "wr_lbne.vi"("DATA"=w209, "ADDRESS"=u16 6 ("address")) -> ()  [unwired: 1 out]
                n128 = To Unsigned Long Integer(number=w214) -> (unsigned 32bit integer=w215:u32)
                n129 = Boolean Array To Number(Boolean array=w205) -> (number=w206:u32)
                "FF_B_SHFT" <- w206
                n130 = Boolean Array To Number(Boolean array=w203) -> (number=w202:u32)
                "FF_B_SHFT 2" <- w202
                n131 = Logical Shift(y=i16 16, x="TEST PAT") -> (x << y=w218:u32)
                n132 = Logical Shift(y=i16 31, x=w215) -> (x << y=w217:u32)
                n133 = call "wr_lbne.vi"("DATA"=w206, "ADDRESS"=u16 4 ("address")) -> ()  [unwired: 1 out]
                n134 = call "wr_lbne.vi"("DATA"=w202, "ADDRESS"=u16 14 ("address")) -> ()  [unwired: 1 out]
                n135 = Compound Arithmetic op=OR("TEST EN", w218, w217) -> (w212:u32)
                "result" <- w212
                n136 = call "wr_lbne.vi"("DATA"=w212, "ADDRESS"=u16 3 ("address")) -> ()  [unwired: 1 out]
              }
              event "STOP_DATA": Value Change {
                n137 = event-data() -> ()  [unwired: 1 in, 6 out]
                n138 = Select(t=2.0, s="STOP_DATA", f=0.0) -> (s? t:f=w236:dbl)
                n139 = call "wr_lbne.vi"("DATA"=w236, "ADDRESS"=u16 30 ("address")) -> ()  [unwired: 1 out]
              }
              event "FREQ", "DLY", "AMPL": Value Change {
                n140 = event-data() -> ()  [unwired: 1 in, 6 out]
                n141 = Join Numbers(hi="DLY", lo="AMPL") -> ((hi.lo)=w240:u16)
                n142 = Join Numbers(hi="FREQ", lo=w240) -> ((hi.lo)=w238:u32)
                "TP_RES" <- w238
                n143 = call "wr_lbne.vi"("DATA"=w238, "ADDRESS"=u16 5) -> ()  [unwired: 1 out]
              }
              event "SYNC": Value Change {
                n144 = event-data() -> ()  [unwired: 1 in, 6 out]
                n145 = Boolean To (0,1)(Boolean="SYNC 3") -> (0, 1=w245:i16)
                n146 = Boolean To (0,1)(Boolean="SYNC") -> (0, 1=w247:i16)
                n147 = To Unsigned Byte Integer(number=w247) -> (unsigned 8bit integer=w246:u8)
                n148 = To Unsigned Byte Integer(number=w245) -> (unsigned 8bit integer=w244:u8)
                n149 = Join Numbers(hi=w244, lo=w246) -> ((hi.lo)=w248:u16)
                n150 = call "wr_lbne.vi"("DATA"=w248, "ADDRESS"=u16 16) -> ()  [unwired: 1 out]
              }
              event "samples 3": Value Change {
                n151 = event-data() -> ()  [unwired: 1 in, 6 out]
                n152 = global read "LBNE_Global .vi" "LBNE_REF"() -> (w253:refnum<k24>)
                n153 = property class="LBNE_COMM"(reference=w253, "HIST_samples"="samples 3") -> ()  [unwired: 1 in, 2 out]
              }
              event "CHANNEL", "CHIP", "ASIC/CHN READOUT": Value Change {
                n154 = event-data() -> ()  [unwired: 1 in, 6 out]
                n155 = global read "LBNE_Global .vi" "LBNE_REF"() -> (w258:refnum<k24>)
                n156 = property class="LBNE_COMM"(reference=w258, "CHN_SEL"="CHANNEL") -> ()  [unwired: 1 in, 2 out]
                n157 = Join Numbers(hi="CHANNEL", lo="CHIP") -> ((hi.lo)=w260:u16)
                n158 = Boolean To (0,1)(Boolean="ASIC/CHN READOUT") -> (0, 1=w255:i16)
                n159 = call "wr_lbne.vi"("DATA"=w255, "ADDRESS"=u16 17 ("address")) -> ()  [unwired: 1 out]
                n160 = call "wr_lbne.vi"("DATA"=w260, "ADDRESS"=u16 7 ("address")) -> ()  [unwired: 1 out]
              }
              event "RESTART": Value Change {
                n161 = event-data() -> ()  [unwired: 1 in, 6 out]
                n162 = local read "START VOLTAGE"() -> (w262:dbl)
                n163 = local write "Voltage Level"(w262) -> ()
              }
            }
            n164 = Wait Until Next ms Multiple(millisecond multiple=u32 10) -> ()  [unwired: 1 out]
            n165 = case shown="True" "RESET 6" {
              frame False {
              }
              frame True {
                n166 = global read "LBNE_Global .vi" "LBNE_REF"() -> (w263:refnum<k24>)
                n167 = property class="LBNE_COMM"(reference=w263, "LV_READY"=FALSE) -> ()  [unwired: 1 in, 2 out]
                n168 = global read "LBNE_Global .vi" "LBNE_REF"() -> (w266:refnum<k24>)
                n169 = Initialize Array(u32 0 ("element"), 16 ("dimension size"), 4096 ("dimension size")) -> (w270:u32[][])
                n170 = Initialize Array(0.0 ("element"), 16 ("dimension size")) -> (w273:dbl[])
                n171 = Initialize Array(u32 0 ("element"), 16 ("dimension size")) -> (w275:u32[])
                n172 = property class="LBNE_COMM"(reference=w266, "ADC_hist"=w270, "ADC_avg"=w273, "ADC_savg"=w273, "ADC_samples"=w275, "number_of_samples"="number_of_samples") -> ()  [unwired: 1 in, 2 out]
              }
            }
            n173 = case shown="True" "SAVE TO \nFILE" {
              frame False {
              }
              frame True {
                n174 = local read "Store_Data"() -> (w182:bool)
                n175 = case shown="False" w182 {
                  frame False {
                    n176 = stacked-sequence {
                      seq-local: [w184 _] -> [_ w196]
                      seq-local: [w183 _] -> [_ w195]
                      frame #0 {
                        n177 = Concatenate Strings("FILE NAME 2", ".txt" ("string")) -> (w186:string)
                        n178 = Build Path(base path="FILE PATH", name or relative path=w186) -> (appended path=w184:path)
                        n179 = call <vilib>:"Check if File or Folder Exists.vi"("path"=w184) -> ("file or folder exists?"=w187:bool)  [unwired: 8 in, 2 out]
                        n180 = case shown="False" w187 {
                          tunnel: [TRUE ("T button?") w193] -> w183
                          frame False {
                          }
                          frame True {
                            n181 = Two Button Dialog(message="FILE EXISTS DO YOU \nWANT TO OVERWRITE", 1:"NO" ("F button name (\"Cancel\")"), 2:"YES" ("T button name (\"OK\")")) -> (T button?=w193:bool)
                          }
                        }
                      }
                      frame #1 {
                        n182 = Path To String(path=w196) -> (string=w197:string)
                        n183 = case shown="True" w195 {
                          tunnel: w197 -> [_ w199]
                          frame False {
                          }
                          frame True {
                            n184 = global read "LBNE_Global .vi" "LBNE_REF"() -> (w198:refnum<k24>)
                            n185 = invoke class="LBNE_COMM" method="open_file"(reference=w198, "File_name"=w199) -> ()  [unwired: 2 in, 4 out]
                          }
                        }
                      }
                    }
                  }
                  frame True {
                    n186 = global read "LBNE_Global .vi" "LBNE_REF"() -> (w200:refnum<k24>)
                    n187 = invoke class="LBNE_COMM" method="open_file"(reference=w200, "File_name"="") -> ()  [unwired: 2 in, 4 out]
                  }
                }
              }
            }
            n188 = global read "LBNE_Global .vi" "LBNE_REF"() -> (w70:refnum<k24>)
            n189 = property class="LBNE_COMM"(reference=w70) -> ("Store_Data"=→"Store_Data":bool)  [unwired: 1 in, 2 out]
          }
          frame "LBNE AUTO CAL" {
            n190 = case shown="True" "START" {
              frame False {
                n191 = global read "LBNE_Global .vi" "LBNE_REF"() -> (w279:refnum<k24>)
                n192 = property class="LBNE_COMM"(reference=w279) -> ("Store_Data"=w278:bool)  [unwired: 1 in, 2 out]
                n193 = local write "Store_Data 2"(w278) -> ()
                n194 = case shown="True" w278 {
                  frame False {
                  }
                  frame True {
                    n195 = global read "LBNE_Global .vi" "LBNE_REF"() -> (w281:refnum<k24>)
                    n196 = invoke class="LBNE_COMM" method="open_file"(reference=w281, "File_name"="") -> ()  [unwired: 2 in, 4 out]
                  }
                }
              }
              frame True {
                n197 = stacked-sequence {
                  frame #0 {
                    w284 = 16 ("dimension size")
                    w286 = 16 ("dimension size")
                    n198 = Join Numbers(hi="DLY 2", lo="AMPL 2") -> ((hi.lo)=w293:u16)
                    n199 = Boolean To (0,1)(Boolean="SYNC 2") -> (0, 1=w297:i16)
                    n200 = Join Numbers(hi="FREQ 2", lo=w293) -> ((hi.lo)=w295:u32)
                    n201 = call "wr_lbne.vi"("DATA"=w297, "ADDRESS"=u16 13) -> ()  [unwired: 1 out]
                    n202 = call "wr_lbne.vi"("DATA"=w295, "ADDRESS"=u16 5) -> ()  [unwired: 1 out]
                    n203 = global read "LBNE_Global .vi" "LBNE_REF"() -> (w299:refnum<k24>)
                    n204 = global read "LBNE_Global .vi" "LBNE_REF"() -> (w300:refnum<k24>)
                    n205 = property class="LBNE_COMM"(reference=w299) -> ("Store_Data"=w298:bool)  [unwired: 1 in, 2 out]
                    "Store_Data 2" <- w298
                    n206 = Initialize Array(FALSE ("Store_Data"), w284, w284) -> (w283:bool[][])
                    n207 = Initialize Array(0.0 ("element"), w286, w286) -> (w287:dbl[][])
                    n208 = property class="LBNE_COMM"(reference=w300, "HIST_samples"=u32 0) -> ()  [unwired: 1 in, 2 out]
                    n209 = local write "MEAN"(w287) -> ()
                    n210 = local write "PEAK"(w287) -> ()
                    n211 = local write "RMS"(w287) -> ()
                    n212 = local write "PASS FAIL"(w283) -> ()
                    n213 = case shown="True" w298 {
                      frame False {
                      }
                      frame True {
                        n214 = global read "LBNE_Global .vi" "LBNE_REF"() -> (w304:refnum<k24>)
                        n215 = invoke class="LBNE_COMM" method="open_file"(reference=w304, "File_name"="") -> ()  [unwired: 2 in, 4 out]
                      }
                    }
                    "CUR_CHN" <- "Start channel"
                    "CUR_CHP" <- "Start chip"
                  }
                  frame #1 {
                    n216 = while {
                      stop <- w307 stop-if-true
                      n217 = stacked-sequence {
                        tunnel: [_ _ w346 _ _] -> w306
                        tunnel: [_ _ _ _ w424] -> w305
                        frame #0 {
                          n218 = case shown="True" "SAVE TO \nFILE 2" {
                            frame False {
                            }
                            frame True {
                              n219 = local read "CUR_CHN"() -> (w315:u8)
                              n220 = Equal To 0?(x=w315) -> (x = 0?=w314:bool)
                              n221 = case shown="True" w314 {
                                frame False {
                                }
                                frame True {
                                n222 = stacked-sequence {
                                frame #0 {
                                n223 = global read "LBNE_Global .vi" "LBNE_REF"() -> (w317:refnum<k24>)
                                n224 = property class="LBNE_COMM"(reference=w317) -> ("Store_Data"=w316:bool)  [unwired: 1 in, 2 out]
                                n225 = case shown="True" w316 {
                                frame False {
                                }
                                frame True {
                                n226 = global read "LBNE_Global .vi" "LBNE_REF"() -> (w318:refnum<k24>)
                                n227 = invoke class="LBNE_COMM" method="open_file"(reference=w318, "File_name"="") -> ()  [unwired: 2 in, 4 out]
                                }
                                }
                                }
                                frame #1 {
                                n228 = Wait Until Next ms Multiple(millisecond multiple=u32 100) -> ()  [unwired: 1 out]
                                }
                                frame #2 {
                                n229 = local read "CUR_CHP"() -> (w322:u8)
                                n230 = Format Into String(format string="_CHIP_%d.bin", initial string="FILE NAME 3", w322) -> (resulting string=w324:string)  [unwired: 1 in, 1 out]
                                n231 = Build Path(base path="FILE PATH 2", name or relative path=w324) -> (appended path=w325:path)
                                n232 = global read "LBNE_Global .vi" "LBNE_REF"() -> (w327:refnum<k24>)
                                n233 = Path To String(path=w325) -> (string=w326:string)
                                n234 = invoke class="LBNE_COMM" method="open_file"(reference=w327, "File_name"=w326) -> ()  [unwired: 2 in, 4 out]
                                }
                                frame #3 {
                                n235 = Wait Until Next ms Multiple(millisecond multiple=u32 50) -> ()  [unwired: 1 out]
                                }
                                }
                                }
                              }
                            }
                          }
                          n236 = local read "CUR_CHN"() -> (w310:u8)
                          n237 = local read "CUR_CHP"() -> (w309:u8)
                          n238 = global read "LBNE_Global .vi" "LBNE_REF"() -> (w311:refnum<k24>)
                          n239 = property class="LBNE_COMM"(reference=w311, "CHN_SEL"=w310) -> ()  [unwired: 1 in, 2 out]
                          n240 = Join Numbers(hi=w310, lo=w309) -> ((hi.lo)=w312:u16)
                          n241 = call "wr_lbne.vi"("DATA"=w312, "ADDRESS"=u16 7 ("address")) -> ()  [unwired: 1 out]
                        }
                        frame #1 {
                          n242 = global read "LBNE_Global .vi" "LBNE_REF"() -> (w331:refnum<k24>)
                          n243 = global read "LBNE_Global .vi" "LBNE_REF"() -> (w332:refnum<k24>)
                          n244 = property class="LBNE_COMM"(reference=w331) -> ("Store_Data"=w330:bool)  [unwired: 1 in, 2 out]
                          n245 = global read "LBNE_Global .vi" "LBNE_REF"() -> (w335:refnum<k24>)
                          n246 = Initialize Array(u32 0 ("element"), 16 ("dimension size"), 4096 ("dimension size")) -> (w339:u32[][])
                          n247 = Initialize Array(0.0 ("element"), 16 ("dimension size")) -> (w342:dbl[])
                          n248 = Initialize Array(u32 0 ("element"), 16 ("dimension size")) -> (w344:u32[])
                          n249 = property class="LBNE_COMM"(reference=w332, "LV_READY"=FALSE) -> ()  [unwired: 1 in, 2 out]
                          n250 = property class="LBNE_COMM"(reference=w335, "ADC_hist"=w339, "ADC_avg"=w342, "ADC_savg"=w342, "ADC_samples"=w344, "number_of_samples"=u32 6000 ("number_of_samples 2")) -> ()  [unwired: 1 in, 2 out]
                          n251 = local write "Store_Data 2"(w330) -> ()
                        }
                        frame #2 {
                          n252 = while {
                            tunnel: ["stop 2"] -> w346
                            stop <- w351 stop-if-true
                            n253 = global read "LBNE_Global .vi" "LBNE_REF"() -> (w348:refnum<k24>)
                            n254 = property class="LBNE_COMM"(reference=w348) -> ("LV_READY"=w347:bool)  [unwired: 1 in, 2 out]
                            n255 = case shown="True" w347 {
                              tunnel: [FALSE w353] -> w349
                              frame False {
                              }
                              frame True {
                                n256 = stacked-sequence {
                                tunnel: [w358 _] -> w354
                                frame #0 {
                                n257 = global read "LBNE_Global .vi" "LBNE_REF"() -> (w375:refnum<k24>)
                                n258 = property class="LBNE_COMM"(reference=w375) -> ("receive_word_array"=w357:u32[], "ADC_hist"=w373:u32[][], "ADC_samples"=w367:u32[])  [unwired: 1 in, 2 out]
                                "Waveform Graph 7" <- w357
                                n259 = local read "CUR_CHN"() -> (w359:u8)
                                n260 = Index Array(array=w367, index=w359) -> (element=w358:u32)
                                "samples 5" <- w358
                                n261 = Array Max & Min(array=w357) -> (max value=w376:u32)  [unwired: 3 out]
                                n262 = Index Array(array=w373, index (row)=w359) -> (element=w361:u32[])  [unwired: 1 in]
                                n263 = Array Max & Min(array=w361) -> (max index (indices)=→"ADC_PEAK 2":i32)  [unwired: 3 out]
                                n264 = Subtract(x=w376, y=30) -> (x-y=w377:u32)
                                n265 = Array Subset(array=w361, length=4096) -> (→"ADC HIST  2":u32[])  [unwired: 1 in]
                                n266 = call "Collector"() -> ()  [unwired: 10 in, 2 out]
                                n267 = case shown="True" "AUTO SCALE 2" {
                                frame False {
                                }
                                frame True {
                                n268 = local read "ADC_PEAK 2"() -> (w393:u32)
                                n269 = Add(x="x 2", y=w393) -> (x+y=w392:u32)
                                n270 = Subtract(x=w393, y="x 2") -> (x-y=w391:u32)
                                n271 = property on="ADC HIST  2" class="WFGraph (strict)"("XScale.Maximum"=w392, "XScale.Minimum"=w391) -> ()  [unwired: 2 in, 2 out]
                                }
                                }
                                n272 = call "Convert to Dynamic Data2"("Array"=w357) -> ("Dynamic Data Type"=w371:dynamicdata)  [unwired: 3 in]
                                n273 = call <vilib>:"Peak Detector.vi"("peaks/valleys"=enum32{"Peaks", "Valleys"}."Peaks", "width"=5, "threshold"=w377, "X"=w357) -> ("Locations"=w365:dbl[], "# found"=w363:i32)  [unwired: 3 in, 3 out]
                                n274 = call "Statistics2"("Signals"=w371) -> ("Total Samples"=→"ADC_CNT 2":dynamicdata, "Standard Dev"=→"ADC_RMS 2":dynamicdata, "Arithmetic Mean"=→"ADC_MEAN 2":dynamicdata)  [unwired: 23 in, 1 out]
                                n275 = Greater Or Equal?(x=w363, y=3 ("x")) -> (x >= y?=w366:bool)
                                n276 = case shown="True" w366 {
                                tunnel: w365 -> [_ w389]
                                tunnel: w357 -> [_ w385]
                                frame False {
                                }
                                frame True {
                                n277 = Index Array(array=w389, index=1) -> (element=w386:dbl)
                                n278 = Divide(x="length 2", y=2) -> (x/y=w383:dbl)
                                n279 = Subtract(x=w386, y=w383) -> (x-y=w384:dbl)
                                n280 = Array Subset(array=w385, index=w384, length="length 2") -> (→"Waveform Graph 6":u32[])
                                }
                                }
                                n281 = Wait Until Next ms Multiple(millisecond multiple=u32 10) -> ()  [unwired: 1 out]
                                }
                                frame #1 {
                                n282 = global read "LBNE_Global .vi" "LBNE_REF"() -> (w394:refnum<k24>)
                                n283 = property class="LBNE_COMM"(reference=w394, "LV_READY"=FALSE) -> ()  [unwired: 1 in, 2 out]
                                }
                                }
                                n284 = local read "samples 6"() -> (w355:i32)
                                n285 = Less Or Equal?(x=w355, y=w354) -> (x <= y?=w353:bool)
                              }
                            }
                            n286 = Or(x=w349, y="stop 2") -> (x .or. y?=w351:bool)
                          }
                        }
                        frame #3 {
                          n287 = local read "ADC_PEAK 2"() -> (w401:u32)
                          n288 = local read "ADC_MEAN 2"() -> (w412:dbl)
                          n289 = In Range and Coerce(upper limit="peak upper limit", x=w401, lower limit="peak lower limit") -> (In Range?=w404:bool)  [unwired: 1 out]
                          n290 = In Range and Coerce(upper limit="Mean upper limit", x=w412, lower limit="Mean lower limit") -> (In Range?=w407:bool)  [unwired: 1 out]
                          n291 = Not(x="EN peak") -> (.not. x?=w396:bool)
                          n292 = Not(x="EN mean") -> (.not. x?=w398:bool)
                          n293 = Or(x=w396, y=w404) -> (x .or. y?=w400:bool)
                          n294 = Or(x=w398, y=w407) -> (x .or. y?=w406:bool)
                          n295 = local read "ADC_RMS 2"() -> (w415:dbl)
                          n296 = local read "ADC_PEAK 2"() -> (w416:u32)
                          n297 = local read "ADC_MEAN 2"() -> (w417:dbl)
                          n298 = local read "CUR_CHN"() -> (w408:u8)
                          n299 = local read "CUR_CHP"() -> (w409:u8)
                          n300 = local read "MEAN"() -> (w422:dbl[][])
                          n301 = local read "PASS FAIL"() -> (w413:bool[][])
                          n302 = local read "PEAK"() -> (w421:dbl[][])
                          n303 = Compound Arithmetic op=AND(w406, w400) -> (w405:bool)
                          n304 = local read "RMS"() -> (w419:dbl[][])
                          n305 = Replace Array Subset(array=w422, new element=w417, index (row)=w408, index (col)=w409) -> (→"MEAN":dbl[][])
                          n306 = Replace Array Subset(array=w413, new element=w405, index (row)=w408, index (col)=w409) -> (→"PASS FAIL":bool[][])
                          n307 = Replace Array Subset(array=w421, new element=w416, index (row)=w408, index (col)=w409) -> (→"PEAK":dbl[][])
                          n308 = Replace Array Subset(array=w419, new element=w415, index (row)=w408, index (col)=w409) -> (→"RMS":dbl[][])
                        }
                        frame #4 {
                          n309 = flat-sequence {
                            tunnel: [w434] -> w424
                            frame #0 {
                              n310 = local read "CUR_CHN"() -> (w428:u8)
                              n311 = Increment(x=w428) -> (x+1=w427:u8)
                              n312 = Greater Or Equal?(x=w427, y=u8 16) -> (x >= y?=w426:bool)
                              n313 = case shown="True" w426 {
                                frame False {
                                n314 = local read "CUR_CHN"() -> (w430:u8)
                                n315 = Increment(x=w430) -> (x+1=w429:u8)
                                n316 = local write "CUR_CHN"(w429) -> ()
                                }
                                frame True {
                                n317 = local read "CUR_CHP"() -> (w432:u8)
                                n318 = local write "CUR_CHN"(u8 0 ("CUR_CHN")) -> ()
                                n319 = Increment(x=w432) -> (x+1=w431:u8)
                                n320 = local write "CUR_CHP"(w431) -> ()
                                }
                              }
                            }
                            frame #1 {
                              n321 = local read "CUR_CHP"() -> (w436:u8)
                              n322 = Greater Or Equal?(x=w436, y=u8 8) -> (x >= y?=w434:bool)
                            }
                          }
                        }
                      }
                      n323 = Or(x=w306, y=w305) -> (x .or. y?=w307:bool)
                    }
                  }
                }
              }
            }
          }
          frame "FPGA FLASH" {
            n324 = case shown="False" "verify\nFLASH" {
              frame False {
              }
              frame True {
                n325 = local read "FROM FILE"() -> (w475:u32[][])
                n326 = for {
                  tunnel: w475 -> [w481]
                  tunnel: "start from" -> [w477]
                  tunnel: w475 -> [_] mode=indexing
                  i -> [w479]
                  stop <- w483 continue-if-true
                  n327 = local read "pages 2"() -> (w489:dbl)
                  n328 = Index Array(array=w481) -> (element=w480:u32[])  [unwired: 2 in]
                  n329 = Add(x=w477, y=w479) -> (x+y=w478:i32)
                  "PAGE 2" <- w478
                  n330 = Divide(x=w478, y=w489) -> (x/y=w487:dbl)
                  n331 = Multiply(x=100.0, y=w487) -> (x*y=→"Meter 2":dbl)
                  n332 = Multiply(x=256 ("length"), y=w478) -> (x*y=w491:i32)
                  n333 = stacked-sequence {
                    seq-local: [_ w494 _] -> [_ _ w517]
                    tunnel: w480 -> [_ _ w514]
                    tunnel: w491 -> [w492 _ _]
                    tunnel: [_ _ w518] -> w482
                    frame #0 {
                      n334 = call "wr_lbne.vi"("DATA"=w492, "ADDRESS"=u16 11) -> ()  [unwired: 1 out]
                    }
                    frame #1 {
                      n335 = stacked-sequence {
                        tunnel: [_ _ _ _ w502] -> w494
                        frame #0 {
                          w495 = u32 3  # opcode
                          n336 = call "wr_lbne.vi"("DATA"=w495, "ADDRESS"=u16 10) -> ()  [unwired: 1 out]
                        }
                        frame #1 {
                          w497 = u32 259  # opcode
                          n337 = call "wr_lbne.vi"("DATA"=w497, "ADDRESS"=u16 10) -> ()  [unwired: 1 out]
                        }
                        frame #2 {
                          w499 = u32 0  # opcode
                          n338 = call "wr_lbne.vi"("DATA"=w499, "ADDRESS"=u16 10) -> ()  [unwired: 1 out]
                        }
                        frame #3 {
                          n339 = Wait Until Next ms Multiple(millisecond multiple=u32 10) -> ()  [unwired: 1 out]
                        }
                        frame #4 {
                          n340 = for {
                            N: 4 -> [_]
                            shift-right: [w507] -> w502
                            shift-left: u32[] [] ("DATA") -> [w508]
                            i -> [w510]
                            n341 = Multiply(x=16, y=w510) -> (x*y=w511:i32)
                            n342 = Add(x=u32 128, y=w511) -> (x+y=w506:u32)
                            n343 = call "rd_lbne_BLK.vi"("ADDRESS 2"=w506) -> ("Array"=w505:u32[])
                            n344 = Build Array (concatenate)(w508, w505) -> (w507:u32[])
                          }
                        }
                      }
                    }
                    frame #2 {
                      n345 = Select(t=u32[] [4294967295, 4294967295, 4294967295, 4294967295, 4294967295, 4294967295, 4294967295, 4294967295, 4294967295, 4294967295, 4294967295, 4294967295, 4294967295, 4294967295, 4294967295, 4294967295, 4294967295, 4294967295, 4294967295, 4294967295, 4294967295, 4294967295, 4294967295, 4294967295, 4294967295, 4294967295, 4294967295, 4294967295, 4294967295, 4294967295, 4294967295, 4294967295, 4294967295, 4294967295, 4294967295, 4294967295, 4294967295, 4294967295, 4294967295, 4294967295, 4294967295, 4294967295, 4294967295, 4294967295, 4294967295, 4294967295, 4294967295, 4294967295, 4294967295, 4294967295, 4294967295, 4294967295, 4294967295, 4294967295, 4294967295, 4294967295, 4294967295, 4294967295, 4294967295, 4294967295, 4294967295, 4294967295, 4294967295, 4294967295] ("READ ARRAY 4"), s="blank check", f=w514) -> (s? t:f=w516:u32[])
                      "WRITE ARRAY 2" <- w516
                      n346 = Equal?(x=w517, y=w516) -> (x = y?=w518:bool)
                      "x = y? 2" <- w518
                      "READ ARRAY 3" <- w517
                    }
                  }
                  n347 = Not(x="STOP VERIFY") -> (.not. x?=w484:bool)
                  n348 = And(x=w482, y=w484) -> (x .and. y?=w483:bool)
                }
              }
            }
            n349 = case shown="True" "program \nFLASH" {
              frame False {
              }
              frame True {
                n350 = stacked-sequence {
                  frame #0 {
                    n351 = local write "NUM ATTEMP"(0 ("NUM ATTEMP")) -> ()
                    n352 = local write "PAGE 3"("START FROM") -> ()
                    n353 = call "wr_lbne.vi"("DATA"=u32 1, "ADDRESS"=u16 9) -> ()  [unwired: 1 out]
                    n354 = call "wr_lbne.vi"("DATA"=u32 1, "ADDRESS"=u16 13) -> ()  [unwired: 1 out]
                    "ONE_MORE" <- -1 ("ONE_MORE")
                  }
                  frame #1 {
                    n355 = local read "FROM FILE"() -> (w557:u32[][])
                    n356 = while {
                      tunnel: w557 -> [w565]
                      tunnel: "Numeric" -> [w566]
                      stop <- w558 continue-if-true
                      n357 = local read "PAGE 3"() -> (w559:i32)
                      n358 = Divide(x=w559, y=w566) -> (x/y=w568:dbl)
                      n359 = Multiply(x=100.0, y=w568) -> (x*y=→"Meter":dbl)
                      n360 = Index Array(array=w565, index (row)=w559) -> (element=w564:u32[])  [unwired: 1 in]
                      n361 = Multiply(x=256 ("length"), y=w559) -> (x*y=w570:i32)
                      n362 = stacked-sequence {
                        seq-local: [w571 _ _ _ _ _] -> [_ _ _ _ _ w643]
                        seq-local: [_ _ _ _ w621 _] -> [_ _ _ _ _ w642]
                        tunnel: w564 -> [w572 _ _ _ _ _]
                        tunnel: w570 -> [_ _ w599 _ _ _]
                        tunnel: [_ _ _ _ _ w641] -> w563
                        frame #0 {
                          n363 = while {
                            tunnel: w572 -> [w578]
                            tunnel: [w575] -> w571
                            stop <- w573 stop-if-true
                            (unwired) FALSE
                            # "load fifo"
                            n364 = for {
                              tunnel: w578 -> [w588] mode=indexing
                              tunnel: [w588] -> w575 mode=indexing
                              tunnel: [4] -> w574
                              i -> [w590]
                              n365 = Add(x=u32 64, y=w590) -> (x+y=w589:u32)
                              n366 = call "wr_lbne.vi"("DATA"=w588, "ADDRESS"=w589) -> ()  [unwired: 1 out]
                            }
                            n367 = for {
                              N: w574 -> [_]
                              shift-right: [w581] -> w576
                              shift-left: u32[] [] ("DATA") -> [w582]
                              i -> [w584]
                              n368 = Multiply(x=16, y=w584) -> (x*y=w585:i32)
                              n369 = Add(x=u32 64, y=w585) -> (x+y=w579:u32)
                              n370 = call "rd_lbne_BLK.vi"("ADDRESS 2"=w579) -> ("Array"=w580:u32[])
                              n371 = Build Array (concatenate)(w582, w580) -> (w581:u32[])
                            }
                            n372 = Equal?(x=w575, y=w576) -> (x = y?=w573:bool)
                            "x = y? 3" <- w573
                          }
                        }
                        frame #1 {
                          # "set write enable"
                          n373 = flat-sequence {
                            frame #0 {
                              n374 = call "wr_lbne.vi"("DATA"=u32 6, "ADDRESS"=u16 10) -> ()  [unwired: 1 out]
                            }
                            frame #1 {
                              n375 = stacked-sequence {
                                frame #0 {
                                n376 = call "wr_lbne.vi"("DATA"=u32 262, "ADDRESS"=u16 10) -> ()  [unwired: 1 out]
                                }
                                frame #1 {
                                n377 = Wait Until Next ms Multiple(millisecond multiple=u32 1) -> ()  [unwired: 1 out]
                                }
                                frame #2 {
                                n378 = call "wr_lbne.vi"("DATA"=u32 0, "ADDRESS"=u16 10) -> ()  [unwired: 1 out]
                                }
                              }
                            }
                          }
                        }
                        frame #2 {
                          n379 = call "wr_lbne.vi"("DATA"=w599, "ADDRESS"=u16 11) -> ()  [unwired: 1 out]
                        }
                        frame #3 {
                          # "write flash"
                          n380 = flat-sequence {
                            frame #0 {
                              n381 = call "wr_lbne.vi"("DATA"=u32 2, "ADDRESS"=u16 10) -> ()  [unwired: 1 out]
                            }
                            frame #1 {
                              n382 = while {
                                stop <- w605 continue-if-true
                                n383 = stacked-sequence {
                                tunnel: [_ _ w609 _] -> w604
                                frame #0 {
                                n384 = call "wr_lbne.vi"("DATA"=u32 258, "ADDRESS"=u16 10) -> ()  [unwired: 1 out]
                                }
                                frame #1 {
                                n385 = Wait Until Next ms Multiple(millisecond multiple=u32 1) -> ()  [unwired: 1 out]
                                }
                                frame #2 {
                                n386 = stacked-sequence {
                                tunnel: [_ _ w617] -> w609
                                frame #0 {
                                n387 = call "wr_lbne.vi"("DATA"=u32 5, "ADDRESS"=u16 10) -> ()  [unwired: 1 out]
                                }
                                frame #1 {
                                n388 = stacked-sequence {
                                frame #0 {
                                n389 = call "wr_lbne.vi"("DATA"=u32 261, "ADDRESS"=u16 10) -> ()  [unwired: 1 out]
                                }
                                frame #1 {
                                n390 = Wait Until Next ms Multiple(millisecond multiple=u32 1) -> ()  [unwired: 1 out]
                                }
                                frame #2 {
                                n391 = call "wr_lbne.vi"("DATA"=u32 5, "ADDRESS"=u16 10) -> ()  [unwired: 1 out]
                                }
                                }
                                }
                                frame #2 {
                                n392 = call "rd_lbne.vi"("ADDRESS 2"=i16 12) -> ("DATA 2"=w617:u32)
                                "DATA 6" <- w617
                                }
                                }
                                }
                                frame #3 {
                                n393 = call "wr_lbne.vi"("DATA"=u32 2, "ADDRESS"=u16 10) -> ()  [unwired: 1 out]
                                }
                                }
                                n394 = Equal?(x=w604, y=u32 3) -> (x = y?=w605:bool)
                              }
                            }
                          }
                        }
                        frame #4 {
                          n395 = stacked-sequence {
                            tunnel: [_ _ _ _ w629] -> w621
                            frame #0 {
                              w622 = u32 3  # opcode
                              n396 = call "wr_lbne.vi"("DATA"=w622, "ADDRESS"=u16 10) -> ()  [unwired: 1 out]
                            }
                            frame #1 {
                              w624 = u32 259  # opcode
                              n397 = call "wr_lbne.vi"("DATA"=w624, "ADDRESS"=u16 10) -> ()  [unwired: 1 out]
                            }
                            frame #2 {
                              w626 = u32 0  # opcode
                              n398 = call "wr_lbne.vi"("DATA"=w626, "ADDRESS"=u16 10) -> ()  [unwired: 1 out]
                            }
                            frame #3 {
                              n399 = Wait Until Next ms Multiple(millisecond multiple=u32 10) -> ()  [unwired: 1 out]
                            }
                            frame #4 {
                              n400 = for {
                                N: 4 -> [_]
                                shift-right: [w634] -> w629
                                shift-left: u32[] [] ("DATA") -> [w635]
                                i -> [w637]
                                n401 = Multiply(x=16, y=w637) -> (x*y=w638:i32)
                                n402 = Add(x=u32 128, y=w638) -> (x+y=w632:u32)
                                n403 = call "rd_lbne_BLK.vi"("ADDRESS 2"=w632) -> ("Array"=w633:u32[])
                                n404 = Build Array (concatenate)(w635, w633) -> (w634:u32[])
                              }
                            }
                          }
                        }
                        frame #5 {
                          n405 = Equal?(x=w642, y=w643) -> (x = y?=w640:bool)
                          "x = y?" <- w640
                          n406 = case shown="True" w640 {
                            tunnel: [TRUE ("x = y? 3") w647] -> w641
                            frame False {
                              n407 = local read "NUM ATTEMP"() -> (w646:i32)
                              n408 = Increment(x=w646) -> (x+1=w644:i32)
                              n409 = local write "NUM ATTEMP"(w644) -> ()
                            }
                            frame True {
                              n410 = local read "NUM ATTEMP"() -> (w650:i32)
                              n411 = local read "ONE_MORE"() -> (w649:i32)
                              n412 = Equal?(x=w650, y=w649) -> (x = y?=w648:bool)
                              n413 = case shown="True" w648 {
                                tunnel: [TRUE ("x = y? 3") w656] -> w647
                                frame False {
                                n414 = local read "NUM ATTEMP"() -> (w652:i32)
                                n415 = local write "ONE_MORE"(w652) -> ()
                                }
                                frame True {
                                n416 = local read "PAGE 3"() -> (w660:i32)
                                n417 = local read "Numeric"() -> (w653:i32)
                                n418 = local write "ONE_MORE"(-1 ("ONE_MORE")) -> ()
                                n419 = Increment(x=w660) -> (x+1=w658:i32)
                                "PAGE 3" <- w658
                                n420 = Equal?(x=w658, y=w653) -> (x = y?=w657:bool)
                                n421 = Select(t=FALSE ("x = y? 3"), s=w657, f=TRUE ("x = y? 3")) -> (s? t:f=w656:bool)
                                "NUM ATTEMP" <- 0 ("NUM ATTEMP")
                                }
                              }
                            }
                          }
                          "WRITE ARRAY" <- w643
                          "READ ARRAY 2" <- w642
                        }
                      }
                      n422 = Not(x="STOP WRITE") -> (.not. x?=w562:bool)
                      n423 = And(x=w563, y=w562) -> (x .and. y?=w558:bool)
                    }
                  }
                }
              }
            }
            n424 = case shown="False" "READ STATUS" {
              frame False {
              }
              frame True {
                n425 = flat-sequence {
                  frame #0 {
                    n426 = call "wr_lbne.vi"("DATA"=u32 1, "ADDRESS"=u16 13) -> ()  [unwired: 1 out]
                    n427 = call "wr_lbne.vi"("DATA"=u32 1, "ADDRESS"=u16 9) -> ()  [unwired: 1 out]
                  }
                  frame #1 {
                    n428 = call "wr_lbne.vi"("DATA"=u32 5, "ADDRESS"=u16 10) -> ()  [unwired: 1 out]
                  }
                  frame #2 {
                    n429 = stacked-sequence {
                      frame #0 {
                        n430 = call "wr_lbne.vi"("DATA"=u32 261, "ADDRESS"=u16 10) -> ()  [unwired: 1 out]
                      }
                      frame #1 {
                        n431 = Wait Until Next ms Multiple(millisecond multiple=u32 1) -> ()  [unwired: 1 out]
                      }
                      frame #2 {
                        n432 = call "wr_lbne.vi"("DATA"=u32 5, "ADDRESS"=u16 10) -> ()  [unwired: 1 out]
                      }
                    }
                  }
                  frame #3 {
                    n433 = call "rd_lbne.vi"("ADDRESS 2"=i16 12) -> ("DATA 2"=→"DATA 5":u32)
                  }
                }
              }
            }
            n434 = case shown="False" "LOAD RPD" {
              frame False {
              }
              frame True {
                w531 = "Choose Binary File"  # Prompt
                n435 = File Dialog(6:"*.rpd" ("pattern (all files)"), 7:w531) -> (0:w535:errorcluster, 3:w530:path)  [unwired: 5 in, 2 out]
                n436 = Open/Create/Replace File(file path (use dialog)=w530, error in=w535, operation (0:open)=T10."open", access (0:read/write)=enum16{"read/write", "read-only", "write-only"}."read-only") -> (refnum out=w538:refnum<file>, error out=w537:errorcluster)  [unwired: 2 in, 1 out]
                n437 = Deny Access(4:w537, 6:T11."deny write-only" ("deny mode (0:deny read/write)"), 7:w538) -> (0:w539:errorcluster, 3:w540:refnum<file>)
                n438 = Get File Size(file=w540, error in=w539) -> (refnum out=w528:refnum<file>, size (in bytes)=w523:i64, 0:w533:errorcluster)
                n439 = Divide(x=w523, y=i64 4) -> (x/y=w521:dbl)
                n440 = Read from Binary File(5:u32 0 ("y"), 8:w533, 10:w521, 11:w528) -> (0:w532:errorcluster, 2:w519:u32[], 3:w529:refnum<file>)  [unwired: 2 in, 1 out]
                n441 = Divide(x=w521, y=u32 64) -> (x/y=w525:dbl)
                n442 = Close File(refnum=w529, error in=w532) -> (error out=→"error out 2":errorcluster)  [unwired: 1 out]
                n443 = Increment(x=w525) -> (x+1=w520:dbl)
                "pages 2" <- w520
                n444 = for {
                  N: w520 -> [_]
                  tunnel: w519 -> [w548]
                  tunnel: [w547] -> w526 mode=indexing
                  i -> [w546]
                  w545 = 64 ("length")
                  n445 = Multiply(x=w545, y=w546) -> (x*y=w544:i32)
                  n446 = Array Subset(array=w548, index=w544, length=w545) -> (w547:u32[])
                }
                "FROM FILE" <- w526
              }
            }
            n447 = case shown="False" "read flash" {
              frame False {
              }
              frame True {
                n448 = for {
                  N: "PAGES" -> [_]
                  tunnel: "P OFFSET" -> [w448]
                  shift-right: [w447] -> _
                  shift-left: u32[][] [] -> [w446]
                  i -> [w449]
                  n449 = Add(x=w448, y=w449) -> (x+y=w450:i32)
                  "PAGE" <- w450
                  n450 = Multiply(x=256 ("length"), y=w450) -> (x*y=w452:i32)
                  n451 = stacked-sequence {
                    tunnel: w452 -> [w453 _ _]
                    tunnel: [_ _ w462] -> w447
                    tunnel: w446 -> [_ _ w463]
                    frame #0 {
                      n452 = call "wr_lbne.vi"("DATA"=w453, "ADDRESS"=u16 11) -> ()  [unwired: 1 out]
                    }
                    frame #1 {
                      n453 = flat-sequence {
                        frame #0 {
                          w455 = u32 3  # opcode
                          n454 = call "wr_lbne.vi"("DATA"=w455, "ADDRESS"=u16 10) -> ()  [unwired: 1 out]
                        }
                        frame #1 {
                          w457 = u32 259  # opcode
                          n455 = call "wr_lbne.vi"("DATA"=w457, "ADDRESS"=u16 10) -> ()  [unwired: 1 out]
                        }
                        frame #2 {
                          w459 = u32 0  # opcode
                          n456 = call "wr_lbne.vi"("DATA"=w459, "ADDRESS"=u16 10) -> ()  [unwired: 1 out]
                        }
                        frame #3 {
                          n457 = Wait Until Next ms Multiple(millisecond multiple=u32 1) -> ()  [unwired: 1 out]
                        }
                      }
                    }
                    frame #2 {
                      n458 = for {
                        N: 4 -> [_]
                        shift-right: [w469] -> w464
                        shift-left: u32[] [] ("DATA") -> [w470]
                        i -> [w472]
                        n459 = Multiply(x=16, y=w472) -> (x*y=w473:i32)
                        n460 = Add(x=u32 128, y=w473) -> (x+y=w467:u32)
                        n461 = call "rd_lbne_BLK.vi"("ADDRESS 2"=w467) -> ("Array"=w468:u32[])
                        n462 = Build Array (concatenate)(w470, w468) -> (w469:u32[])
                      }
                      n463 = Build Array (concatenate)(w463, w464) -> (w462:u32[][])
                      "READ FROM FLASH" <- w462
                    }
                  }
                }
              }
            }
            n464 = case shown="False" "erase flash" {
              frame False {
              }
              frame True {
                n465 = flat-sequence {
                  frame #0 {
                    n466 = call "wr_lbne.vi"("DATA"=u32 1, "ADDRESS"=u16 9) -> ()  [unwired: 1 out]
                    n467 = call "wr_lbne.vi"("DATA"=u32 1, "ADDRESS"=u16 13) -> ()  [unwired: 1 out]
                  }
                  frame #1 {
                    # "erase flash"
                    n468 = stacked-sequence {
                      frame #0 {
                        n469 = call "wr_lbne.vi"("DATA"=u32 6, "ADDRESS"=u16 10) -> ()  [unwired: 1 out]
                      }
                      frame #1 {
                        n470 = call "wr_lbne.vi"("DATA"=u32 262, "ADDRESS"=u16 10) -> ()  [unwired: 1 out]
                      }
                      frame #2 {
                        n471 = call "wr_lbne.vi"("DATA"=u32 0, "ADDRESS"=u16 10) -> ()  [unwired: 1 out]
                      }
                    }
                  }
                  frame #2 {
                    w685 = u32 199  # opcode
                    # "wait for clear flash"
                    n472 = Wait Until Next ms Multiple(millisecond multiple=u32 5) -> ()  [unwired: 1 out]
                    n473 = call "wr_lbne.vi"("DATA"=w685, "ADDRESS"=u16 10) -> ()  [unwired: 1 out]
                  }
                  frame #3 {
                    n474 = stacked-sequence {
                      frame #0 {
                        w688 = u32 455  # opcode
                        n475 = call "wr_lbne.vi"("DATA"=w688, "ADDRESS"=u16 10) -> ()  [unwired: 1 out]
                      }
                      frame #1 {
                        n476 = Wait Until Next ms Multiple(millisecond multiple=u32 1) -> ()  [unwired: 1 out]
                      }
                      frame #2 {
                        w691 = u32 199  # opcode
                        n477 = call "wr_lbne.vi"("DATA"=w691, "ADDRESS"=u16 10) -> ()  [unwired: 1 out]
                      }
                    }
                  }
                  frame #4 {
                    n478 = call "wr_lbne.vi"("DATA"=u32 0, "ADDRESS"=u16 10) -> ()  [unwired: 1 out]
                    n479 = Wait Until Next ms Multiple(millisecond multiple=u32 1000) -> ()  [unwired: 1 out]
                  }
                }
              }
            }
          }
          frame "ASIC SPI" {
            n480 = event shown="[2] \"QUICK SET\": Value Change" {
              selector: _ -> [_ _ _]
              dyn-events: _ -> [_ _ _]
              timeout: 100 -> [_ _ _]
              event Timeout {
                n481 = event-data() -> ()  [unwired: 1 in, 3 out]
              }
              event "Slide": Value Change {
                n482 = event-data() -> ()  [unwired: 1 in, 4 out]
                n483 = Build Array(u8 0 ("element"), "Slide") -> (w783:u8[])
                n484 = Build Array("Slide") -> (w782:u8[])
                n485 = property on="Array 3" class="Arr"("Index Values"=w783) -> ()  [unwired: 2 in, 2 out]
                n486 = property on="Array 4" class="Arr (strict)"("Index Values"=w782) -> ()  [unwired: 2 in, 2 out]
                n487 = property on="CHANNEL 3" class="Arr (strict)"("Index Values"=w783) -> ()  [unwired: 2 in, 2 out]
              }
              event "QUICK SET": Value Change {
                n488 = event-data() -> ()  [unwired: 1 in, 6 out]
                n489 = local read "CHANNEL 3"() -> (w798:T4)
                n490 = local read "Array 3"() -> (w790:T5)
                n491 = local read "Slide"() -> (w793:u8)
                n492 = Index Array(array=w798, index (col)=w793) -> (element=w794:T12)  [unwired: 1 in]
                n493 = Index Array(array=w790, index (col)=w793) -> (element=w789:T13)  [unwired: 1 in]
                n494 = for {
                  tunnel: w794 -> [w848] mode=indexing
                  tunnel: "CHANNEL 4" -> [w850]
                  tunnel: [w849] -> w796 mode=indexing
                  tunnel: w794 -> [w847] mode=indexing
                  tunnel: "channel" -> [w831]
                  tunnel: w789 -> [w830] mode=indexing
                  tunnel: w789 -> [w829] mode=indexing
                  tunnel: [w804] -> w788 mode=indexing
                  n495 = Unbundle By Name(w850) -> ("D_offset"=w840:u16, "PDSR"=w839:bool, "PCSR"=w837:bool, "slp"=w836:bool, "tst"=w800:bool)
                  n496 = Unbundle By Name(w847) -> ("D_offset"=w843:u16, "PDSR"=w842:bool, "PCSR"=w838:bool, "slp"=w841:bool, "tst"=w801:bool)
                  n497 = Unbundle By Name(w831) -> ("sts"=w816:bool, "snc"=w815:bool, "SG"=w814:u16, "ST"=w813:u16, "SDC"=w812:bool, "SDF"=w811:bool)
                  n498 = Unbundle By Name(w830) -> ("sts"=w828:bool, "snc"=w827:bool, "SG"=w826:u16, "ST"=w825:u16, "SDC"=w824:bool, "SDF"=w823:bool)
                  n499 = Select(t=w840, s="s", f=w843) -> (s? t:f=w846:u16)
                  n500 = Select(t=w839, s="s 2", f=w842) -> (s? t:f=w845:bool)
                  n501 = Select(t=w837, s="s 3", f=w838) -> (s? t:f=w844:bool)
                  n502 = Select(t=w836, s="s 4", f=w841) -> (s? t:f=w803:bool)
                  n503 = Select(t=w800, s="s 11", f=w801) -> (s? t:f=w802:bool)
                  n504 = Select(t=w816, s="s 5", f=w828) -> (s? t:f=w805:bool)
                  n505 = Select(t=w815, s="s 6", f=w827) -> (s? t:f=w806:bool)
                  n506 = Select(t=w814, s="s 7", f=w826) -> (s? t:f=w807:u16)
                  n507 = Select(t=w813, s="s 8", f=w825) -> (s? t:f=w808:u16)
                  n508 = Select(t=w812, s="s 9", f=w824) -> (s? t:f=w809:bool)
                  n509 = Select(t=w811, s="s 10", f=w823) -> (s? t:f=w810:bool)
                  n510 = Bundle By Name(cluster=w848, "D_offset"=w846, "PDSR"=w845, "PCSR"=w844, "slp"=w803, "tst"=w802) -> (w849:T3)
                  n511 = Bundle By Name(cluster=w829, "sts"=w805, "snc"=w806, "SG"=w807, "ST"=w808, "SDC"=w809, "SDF"=w810) -> (w804:T2)
                }
                n512 = local read "CHANNEL 3"() -> (w797:T4)
                n513 = local read "Array 3"() -> (w786:T5)
                n514 = local read "Slide"() -> (w787:u8)
                n515 = Replace Array Subset(array=w797, new element=w796, index (col)=w787) -> (w795:T4)  [unwired: 1 in]
                n516 = Replace Array Subset(array=w786, new element=w788, index (col)=w787) -> (w785:T5)  [unwired: 1 in]
                n517 = local write "CHANNEL 3"(w795) -> ()
                n518 = local write "Array 3"(w785) -> ()
              }
            }
            n519 = stacked-sequence {
              tunnel: 8 ("NUMBER OF ASICS") -> [w703 w745]
              frame #0 {
                n520 = for {
                  N: w703 -> [_]
                  tunnel: [w719] -> _ mode=indexing
                  shift-right: [w720] -> w701
                  shift-left: bool[] [] -> [w718]
                  i -> [w712]
                  n521 = Index Array(array="CHANNEL 3", index (col)=w712) -> (element=w716:T12)  [unwired: 1 in]
                  n522 = Reverse 1D Array(array=w716) -> (reversed array=w728:T12)
                  n523 = for {
                    tunnel: w728 -> [w742] mode=indexing
                    shift-right: [w738] -> w715
                    shift-left: bool[] [] -> [w732]
                    n524 = Unbundle By Name(w742) -> ("tst"=w730:bool, "slp"=w731:bool, "PDSR"=w737:bool, "PCSR"=w736:bool, "D_offset"=w735:u16)
                    n525 = Number To Boolean Array(number=w735) -> (Boolean array=w741:bool[])
                    n526 = Array Subset(array=w741, index=0, length=4) -> (w734:bool[])
                    n527 = Reverse 1D Array(array=w734) -> (reversed array=w733:bool[])
                    n528 = Build Array (concatenate)(w732, w730, w731, w737, w736, w733) -> (w738:bool[])
                  }
                  n529 = Index Array(array="Array 4", index=w712) -> (element=w711:T14)
                  n530 = Unbundle By Name(w711) -> ("EN_GR"=w710:u16, "FRQC"=w709:u16, "CLKG"=w708:u16, "F1"=w707:u16)  [unwired: 1 out]
                  n531 = Number To Boolean Array(number=w708) -> (Boolean array=w723:bool[])
                  n532 = Not Equal To 0?(x=w710) -> (x != 0?=w727:bool)
                  n533 = Not Equal To 0?(x=w709) -> (x != 0?=w726:bool)
                  n534 = Not Equal To 0?(x=w707) -> (x != 0?=w714:bool)
                  n535 = Index Array(array=w723, index=1) -> (element=w722:bool)
                  n536 = Index Array(array=w723, index=0) -> (element=w721:bool)
                  n537 = Not(x="EN V6") -> (.not. x?=w706:bool)
                  n538 = Build Array (concatenate)(w715, "EN V6", w706, "EN V6", w727, w726, w722, w721, w714, "EN V6") -> (w719:bool[])
                  n539 = Build Array (concatenate)(w718, w719) -> (w720:bool[])
                }
                "ADC ARRAY" <- w701
                n540 = Array Size(array=w701) -> (size(s)=→"size(s)":i32)
              }
              frame #1 {
                n541 = for {
                  N: w745 -> [_]
                  shift-right: [w750] -> w744
                  shift-left: bool[] [] -> [w748]
                  i -> [w747]
                  w753 = FALSE ("SLK 2")
                  n542 = Index Array(array="Array 3", index (col)=w747) -> (element=w751:T13)  [unwired: 1 in]
                  n543 = for {
                    tunnel: w751 -> [w780] mode=indexing
                    shift-right: [w776] -> w759
                    shift-left: bool[] [] -> [w777]
                    n544 = Unbundle By Name(w780) -> ("sts"=w779:bool, "snc"=w778:bool, "SG"=w769:u16, "ST"=w768:u16, "SDC"=w765:bool, "SDF"=w764:bool)
                    n545 = Number To Boolean Array(number=w769) -> (Boolean array=w775:bool[])
                    n546 = Number To Boolean Array(number=w768) -> (Boolean array=w770:bool[])
                    n547 = Array Subset(array=w775, index=0, length=2) -> (w767:bool[])
                    n548 = Array Subset(array=w770, index=0, length=2) -> (w766:bool[])
                    n549 = Build Array (concatenate)(w777, w779, w778, w767, w766, w765, w764) -> (w776:bool[])
                  }
                  n550 = Number To Boolean Array(number="STB") -> (Boolean array=w755:bool[])
                  n551 = Array Subset(array=w755, index=0, length=2) -> (w762:bool[])
                  n552 = Reverse 1D Array(array=w759) -> (reversed array=w760:bool[])
                  n553 = Reverse 1D Array(array=w762) -> (reversed array=w763:bool[])
                  n554 = Build Array (concatenate)(w760, "SLK", w763, w753, w753, w753, w753, w753) -> (w749:bool[])
                  n555 = Build Array (concatenate)(w748, w749) -> (w750:bool[])
                }
                "FE ARRAY" <- w744
                n556 = Array Size(array=w744) -> (size(s)=→"size(s) 2":i32)
              }
            }
            n557 = case shown="True" "write_string" {
              frame False {
              }
              frame True {
                n558 = stacked-sequence {
                  frame #0 {
                    # "ADC ASIC"
                    n559 = stacked-sequence {
                      frame #0 {
                        n560 = local read "ADC ARRAY"() -> (w863:bool[])
                        n561 = Array Size(array=w863) -> (size(s)=w862:i32)
                        n562 = local read "ADC ARRAY"() -> (w860:bool[])
                        n563 = Divide(x=w862, y=2) -> (x/y=w855:dbl)
                        n564 = Array Subset(array=w860, index=w855) -> (w858:bool[])  [unwired: 1 in]
                        n565 = Array Subset(array=w863, length=w855) -> (w859:bool[])  [unwired: 1 in]
                        n566 = for {
                          N: 35 -> [_]
                          tunnel: w859 -> [w878]
                          tunnel: w858 -> [w876]
                          tunnel: [w865] -> w856 mode=indexing
                          i -> [w867]
                          (unwired) 64 ("y")
                          w877 = 16 ("length")
                          n567 = Multiply(x=w877, y=w867) -> (x*y=w874:i32)
                          n568 = Array Subset(array=w878, index=w874, length=w877) -> (w870:bool[])
                          n569 = Array Subset(array=w876, index=w874, length=16) -> (w871:bool[])
                          n570 = Boolean Array To Number(Boolean array=w870) -> (number=w872:u32)
                          n571 = Boolean Array To Number(Boolean array=w871) -> (number=w873:u32)
                          n572 = To Unsigned Word Integer(number=w872) -> (unsigned 16bit integer=w869:u16)
                          n573 = To Unsigned Word Integer(number=w873) -> (unsigned 16bit integer=w868:u16)
                          n574 = Join Numbers(hi=w868, lo=w869) -> ((hi.lo)=w865:u32)
                          n575 = Add(x=w867, y=512) -> (x+y=w864:i32)
                          n576 = call "wr_lbne.vi"("DATA"=w865, "ADDRESS"=w864) -> ()  [unwired: 1 out]
                        }
                        "Array" <- w856
                      }
                      frame #1 {
                        n577 = flat-sequence {
                          frame #0 {
                            n578 = call "wr_lbne.vi"("DATA"=u32 1, "ADDRESS"=u16 2) -> ()  [unwired: 1 out]
                          }
                          frame #1 {
                            n579 = Wait Until Next ms Multiple(millisecond multiple=u32 10) -> ()  [unwired: 1 out]
                          }
                          frame #2 {
                            n580 = for {
                              N: 35 -> [_]
                              tunnel: [w887] -> w884 mode=indexing
                              i -> [w889]
                              (unwired) 104 ("y")
                              n581 = Wait Until Next ms Multiple(millisecond multiple=u32 1) -> ()  [unwired: 1 out]
                              n582 = Add(x=w889, y=552) -> (x+y=w888:i32)
                              n583 = call "rd_lbne.vi"("ADDRESS 2"=w888) -> ("DATA 2"=w887:u32)
                            }
                            "ADC RB" <- w884
                            n584 = local read "Array"() -> (w883:u32[])
                            n585 = Equal?(x=w884, y=w883) -> (x = y?=→"ADC SPI OK":bool)
                          }
                        }
                      }
                    }
                  }
                  frame #1 {
                    # "FE ASIC"
                    n586 = stacked-sequence {
                      frame #0 {
                        n587 = local read "FE ARRAY"() -> (w898:bool[])
                        n588 = Array Size(array=w898) -> (size(s)=w897:i32)
                        n589 = Divide(x=w897, y=2) -> (x/y=w895:dbl)
                        n590 = Array Subset(array=w898, index=w895) -> (w892:bool[])  [unwired: 1 in]
                        n591 = Array Subset(array=w898) -> (w893:bool[])  [unwired: 2 in]
                        n592 = for {
                          N: 34 -> [_]
                          tunnel: w893 -> [w913]
                          tunnel: w892 -> [w911]
                          tunnel: [w900] -> w891 mode=indexing
                          i -> [w901]
                          (unwired) 64 ("y")
                          w912 = 16 ("length")
                          n593 = Multiply(x=w912, y=w901) -> (x*y=w909:i32)
                          n594 = Array Subset(array=w913, index=w909, length=w912) -> (w905:bool[])
                          n595 = Array Subset(array=w911, index=w909, length=16) -> (w906:bool[])
                          n596 = Boolean Array To Number(Boolean array=w905) -> (number=w907:u32)
                          n597 = Boolean Array To Number(Boolean array=w906) -> (number=w908:u32)
                          n598 = To Unsigned Word Integer(number=w908) -> (unsigned 16bit integer=w903:u16)
                          n599 = To Unsigned Word Integer(number=w907) -> (unsigned 16bit integer=w904:u16)
                          n600 = Join Numbers(hi=w903, lo=w904) -> ((hi.lo)=w900:u32)
                          n601 = Add(x=w901, y=592) -> (x+y=w902:i32)
                          n602 = call "wr_lbne.vi"("DATA"=w900, "ADDRESS"=w902) -> ()  [unwired: 1 out]
                        }
                        "Array 2" <- w891
                      }
                      frame #1 {
                        n603 = flat-sequence {
                          frame #0 {
                            n604 = call "wr_lbne.vi"("DATA"=u32 2, "ADDRESS"=u16 2) -> ()  [unwired: 1 out]
                          }
                          frame #1 {
                            n605 = Wait Until Next ms Multiple(millisecond multiple=u32 10) -> ()  [unwired: 1 out]
                          }
                          frame #2 {
                            n606 = for {
                              N: 34 -> [_]
                              tunnel: [w923] -> w918 mode=indexing
                              i -> [w925]
                              (unwired) 104 ("y")
                              n607 = Wait Until Next ms Multiple(millisecond multiple=u32 1) -> ()  [unwired: 1 out]
                              n608 = Add(x=w925, y=632) -> (x+y=w924:i32)
                              n609 = call "rd_lbne.vi"("ADDRESS 2"=w924) -> ("DATA 2"=w923:u32)
                            }
                            "FE RB" <- w918
                            n610 = local read "Array 2"() -> (w917:u32[])
                            n611 = Equal?(x=w918, y=w917) -> (x = y?=→"FE SPI OK":bool)
                          }
                        }
                      }
                    }
                  }
                  frame #2 {
                    n612 = local read "EN V6"() -> (w928:bool)
                    n613 = call "rd_lbne.vi"("ADDRESS 2"=i16 6) -> ("DATA 2"=w930:u32)
                    n614 = Split Number(x=w930) -> (hi(x)=→"ADC FIFO SYNC":u16)  [unwired: 1 out]
                    n615 = Boolean To (0,1)(Boolean=w928) -> (0, 1=w927:i16)
                    n616 = call "wr_lbne.vi"("DATA"=w927, "ADDRESS"=u16 18) -> ()  [unwired: 1 out]
                  }
                }
              }
            }
            n617 = case shown="True" "OK Button 2" {
              frame False {
              }
              frame True {
                n618 = flat-sequence {
                  frame #0 {
                    n619 = call "wr_lbne.vi"("DATA"=u16 1 ("ADDRESS"), "ADDRESS"=u16 1) -> ()  [unwired: 1 out]
                  }
                  frame #1 {
                    n620 = call "wr_lbne.vi"("DATA"=u16 2 ("ADDRESS"), "ADDRESS"=u16 1) -> ()  [unwired: 1 out]
                  }
                }
              }
            }
            n621 = Wait Until Next ms Multiple(millisecond multiple=u32 10) -> ()  [unwired: 1 out]
          }
        }
      }
    }
    frame #2 {
      n622 = flat-sequence {
        frame #0 {
          n623 = global read "LBNE_Global .vi" "LBNE_REF"() -> (w934:refnum<k24>)
          n624 = invoke class="LBNE_COMM" method="UDP_CLEANUP"(reference=w934) -> ("UDP_CLEANUP"=→"UDP_CLEANUP":string)  [unwired: 2 in, 2 out]
        }
        frame #1 {
          n625 = Wait Until Next ms Multiple(millisecond multiple=u32 1200) -> ()  [unwired: 1 out]
        }
        frame #2 {
        }
        frame #3 {
        }
      }
      n626 = Request Deallocation(TRUE ("flag")) -> ()
    }
  }
